vi "Beampointing_Multi_Pico3.vi"() -> ()   [LabVIEW 2013]
uses:
  shared programs/GUI_Template/GUI_master/tcp new data cluster.ctl
  <vilib>/Analysis/NI_AALBase.lvlib
  <userlib>/_OpenG.lib/array/array.llb/Filter 1D Array with Scalar (String)__ogtk.vi
  Ctrs/beam detection.ctl
  GUI_Beampointing_single_TRA/Ctrs/move.ctl
  <vilib>/Utility/file.llb/Write To Spreadsheet File (string).vi
  <userlib>/_OpenG.lib/array/array.llb/Filter 1D Array (String)__ogtk.vi
  <vilib>/Utility/file.llb/Read From Spreadsheet File (string).vi
  <vilib>/Utility/error.llb/DialogType.ctl
  shared programs/GUI_Template/GUI_master/tcp_new_data_event.ctl
panel:
  out "x-y*floor(x/y)":dbl
  out "error out":errorcluster
  out "config path":string
  out "Array 3":bool[](array[boolean])
  out "Array 2":u16[](array[numeric])
  out "Array":u16[](array[numeric])
  out "Moving Y":string
  out "Moving X":string
  out "particles":T1(array[cluster])
  out "millisecond timer value":u32
  out "appended path":path
  out "millisecond timer 2":u32
  in  "GUIdevice 98":string="PicoPad4"
  in  "Position.Axis 111::98":dbl=77.0 caption="Motor Axis 1" min=-30000.0 max=30000.0 format="%#_6f"
  in  "Position.Axis 112::98":dbl=77.0 caption="Motor Axis 1" min=-20000.0 max=20000.0 format="%#_6f"
  in  "Position.Axis 113::98":dbl=77.0 caption="Motor Axis 1" min=-20000.0 max=20000.0 format="%#_6f"
  in  "Position.Axis 121::98":dbl=77.0 caption="Motor Axis 1" min=-999999.0 max=999999.0 format="%#_6f"
  in  "Position.Axis 122::98":dbl=77.0 caption="Motor Axis 1" min=-999999.0 max=999999.0 format="%#_6f"
  in  "Position.Axis 123::98":dbl=77.0 caption="Motor Axis 1" min=-999999.0 max=999999.0 format="%#_6f"
  in  "Position.Axis 131::98":dbl=77.0 caption="Motor Axis 1" min=-999999.0 max=999999.0 format="%#_6f"
  in  "Position.Axis 132::98":dbl=77.0 caption="Motor Axis 1" min=-999999.0 max=999999.0 format="%#_6f"
  in  "Position.Axis 133::98":dbl=77.0 caption="Motor Axis 1" min=-999999.0 max=999999.0 format="%#_6f"
  in  "Position.Axis 141::98":dbl=77.0 caption="Motor Axis 1" min=-999999.0 max=999999.0 format="%#_6f"
  in  "Position.Axis 142::98":dbl=77.0 caption="Motor Axis 1" min=-999999.0 max=999999.0 format="%#_6f"
  in  "Position.Axis 143::98":dbl=77.0 caption="Motor Axis 1" min=-999999.0 max=999999.0 format="%#_6f"
  in  "Position.Axis 211::98":dbl=77.0 caption="Motor Axis 1" min=-999999.0 max=999999.0 format="%#_6f"
  in  "Position.Axis 212::98":dbl=77.0 caption="Motor Axis 1" min=-999999.0 max=999999.0 format="%#_6f"
  in  "Position.Axis 213::98":dbl=77.0 caption="Motor Axis 1" min=-999999.0 max=999999.0 format="%#_6f"
  in  "Position.Axis 221::98":dbl=77.0 caption="Motor Axis 1" min=-999999.0 max=999999.0 format="%#_6f"
  in  "Position.Axis 222::98":dbl=77.0 caption="Motor Axis 1" min=-999999.0 max=999999.0 format="%#_6f"
  in  "Position.Axis 223::98":dbl=77.0 caption="Motor Axis 1" min=-999999.0 max=999999.0 format="%#_6f"
  in  "Position.Axis 231::98":dbl=77.0 caption="Motor Axis 1" min=-999999.0 max=999999.0 format="%#_6f"
  in  "Position.Axis 232::98":dbl=77.0 caption="Motor Axis 1" min=-999999.0 max=999999.0 format="%#_6f"
  in  "Position.Axis 233::98":dbl=77.0 caption="Motor Axis 1" min=-999999.0 max=999999.0 format="%#_6f"
  in  "Position.Axis 241::98":dbl=77.0 caption="Motor Axis 1" min=-999999.0 max=999999.0 format="%#_6f"
  in  "Position.Axis 242::98":dbl=77.0 caption="Motor Axis 1" min=-999999.0 max=999999.0 format="%#_6f"
  in  "Position.Axis 243::98":dbl=77.0 caption="Motor Axis 1" min=-999999.0 max=999999.0 format="%#_6f"
  in  "Position.Axis 311::98":dbl=77.0 caption="Motor Axis 1" min=-999999.0 max=999999.0 format="%#_6f"
  in  "Position.Axis 312::98":dbl=77.0 caption="Motor Axis 1" min=-999999.0 max=999999.0 format="%#_6f"
  in  "Position.Axis 313::98":dbl=77.0 caption="Motor Axis 1" min=-999999.0 max=999999.0 format="%#_6f"
  in  "Position.Axis 321::98":dbl=77.0 caption="Motor Axis 1" min=-999999.0 max=999999.0 format="%#_6f"
  in  "Position.Axis 322::98":dbl=77.0 caption="Motor Axis 1" min=-999999.0 max=999999.0 format="%#_6f"
  in  "Position.Axis 323::98":dbl=77.0 caption="Motor Axis 1" min=-999999.0 max=999999.0 format="%#_6f"
  in  "Position.Axis 331::98":dbl=77.0 caption="Motor Axis 1" min=-999999.0 max=999999.0 format="%#_6f"
  in  "Position.Axis 332::98":dbl=77.0 caption="Motor Axis 1" min=-999999.0 max=999999.0 format="%#_6f"
  in  "Position.Axis 333::98":dbl=77.0 caption="Motor Axis 1" min=-999999.0 max=999999.0 format="%#_6f"
  in  "Position.Axis 341::98":dbl=77.0 caption="Motor Axis 1" min=-999999.0 max=999999.0 format="%#_6f"
  in  "Position.Axis 342::98":dbl=77.0 caption="Motor Axis 1" min=-999999.0 max=999999.0 format="%#_6f"
  in  "Position.Axis 343::98":dbl=77.0 caption="Motor Axis 1" min=-999999.0 max=999999.0 format="%#_6f"
  in  "Position.Axis 411::98":dbl=77.0 caption="Motor Axis 1" min=-999999.0 max=999999.0 format="%#_6f"
  in  "Position.Axis 412::98":dbl=77.0 caption="Motor Axis 1" min=-999999.0 max=999999.0 format="%#_6f"
  in  "Position.Axis 413::98":dbl=77.0 caption="Motor Axis 1" min=-999999.0 max=999999.0 format="%#_6f"
  in  "Position.Axis 421::98":dbl=77.0 caption="Motor Axis 1" min=-999999.0 max=999999.0 format="%#_6f"
  in  "Position.Axis 422::98":dbl=77.0 caption="Motor Axis 1" min=-999999.0 max=999999.0 format="%#_6f"
  in  "Position.Axis 423::98":dbl=77.0 caption="Motor Axis 1" min=-999999.0 max=999999.0 format="%#_6f"
  in  "Position.Axis 431::98":dbl=77.0 caption="Motor Axis 1" min=-999999.0 max=999999.0 format="%#_6f"
  in  "Position.Axis 432::98":dbl=77.0 caption="Motor Axis 1" min=-999999.0 max=999999.0 format="%#_6f"
  in  "Position.Axis 433::98":dbl=77.0 caption="Motor Axis 1" min=-999999.0 max=999999.0 format="%#_6f"
  in  "Position.Axis 441::98":dbl=77.0 caption="Motor Axis 1" min=-999999.0 max=999999.0 format="%#_6f"
  in  "Position.Axis 442::98":dbl=77.0 caption="Motor Axis 1" min=-999999.0 max=999999.0 format="%#_6f"
  in  "Position.Axis 443::98":dbl=77.0 caption="Motor Axis 1" min=-999999.0 max=999999.0 format="%#_6f"
  in  "Position.Axis 511::98":dbl=77.0 caption="Motor Axis 1" min=-999999.0 max=999999.0 format="%#_6f"
  in  "Position.Axis 512::98":dbl=77.0 caption="Motor Axis 1" min=-999999.0 max=999999.0 format="%#_6f"
  in  "Position.Axis 513::98":dbl=77.0 caption="Motor Axis 1" min=-999999.0 max=999999.0 format="%#_6f"
  in  "Position.Axis 521::98":dbl=77.0 caption="Motor Axis 1" min=-999999.0 max=999999.0 format="%#_6f"
  in  "Position.Axis 522::98":dbl=77.0 caption="Motor Axis 1" min=-999999.0 max=999999.0 format="%#_6f"
  in  "Position.Axis 523::98":dbl=77.0 caption="Motor Axis 1" min=-999999.0 max=999999.0 format="%#_6f"
  in  "Position.Axis 531::98":dbl=77.0 caption="Motor Axis 1" min=-999999.0 max=999999.0 format="%#_6f"
  in  "Position.Axis 532::98":dbl=77.0 caption="Motor Axis 1" min=-999999.0 max=999999.0 format="%#_6f"
  in  "Position.Axis 533::98":dbl=77.0 caption="Motor Axis 1" min=-999999.0 max=999999.0 format="%#_6f"
  in  "Position.Axis 541::98":dbl=77.0 caption="Motor Axis 1" min=-999999.0 max=999999.0 format="%#_6f"
  in  "Position.Axis 542::98":dbl=77.0 caption="Motor Axis 1" min=-999999.0 max=999999.0 format="%#_6f"
  in  "Position.Axis 543::98":dbl=77.0 caption="Motor Axis 1" min=-999999.0 max=999999.0 format="%#_6f"
  in  "Numeric":dbl
  out "Current State":string
  in  "output cluster 2":T5 {"detection para"."smal para"."Measurement Parameter" items=["Center of Mass X", "Center of Mass Y", "First Pixel X", "First Pixel Y", "Bounding Rect Left", "Bounding Rect Top", "Bounding Rect Right", "Bounding Rect Bottom", "Max Feret Diameter Start X", "Max Feret Diameter Start Y", "Max Feret Diameter End X", "Max Feret Diameter End Y", "Max Horiz. Segment Length Left", "Max Horiz. Segment Length Right", "Max Horiz. Segment Length Row", "-", "Bounding Rect Width", "Bounding Rect Height", "Bounding Rect Diagonal", "Perimeter", "Convex Hull Perimeter", "Holes' Perimeter", "Max Feret Diameter", "Equivalent Ellipse Major Axis", "Equivalent Ellipse Minor Axis", "Equivalent Ellipse Minor Axis (Feret)", "Equivalent Rect Long Side", "Equivalent Rect Short Side", "Equivalent Rect Diagonal", "Equivalent Rect Short Side (Feret)", "Average Horiz. Segment Length", "Average Vert. Segment Length", "Hydraulic Radius", "Waddel Disk Diameter", "-", "Area", "Holes' Area", "Particle & Holes' Area", "Convex Hull Area", "Image Area", "-", "Number of Holes", "Number of Horiz. Segments", "Number of Vert. Segments", "-", "Orientation", "Max Feret Diameter Orientation", "-", "% Area/Image Area", "% Area/(Particle & Holes' Area)", "Ratio of Equivalent Ellipse Axes", "Ratio of Equivalent Rect Sides", "-", "Elongation Factor", "Compactness Factor", "Heywood Circularity Factor", "Type Factor", "-", "Sum X", "Sum Y", "Sum XX", "Sum XY", "Sum YY", "Sum XXX", "Sum XXY", "Sum XYY", "Sum YYY", "-", "Moment of Inertia XX", "Moment of Inertia XY", "Moment of Inertia YY", "Moment of Inertia XXX", "Moment of Inertia XXY", "Moment of Inertia XYY", "Moment of Inertia YYY", "Norm. Moment of Inertia XX", "Norm. Moment of Inertia XY", "Norm. Moment of Inertia YY", "Norm. Moment of Inertia XXX", "Norm. Moment of Inertia XXY", "Norm. Moment of Inertia XYY", "Norm. Moment of Inertia YYY", "Hu Moment 1", "Hu Moment 2", "Hu Moment 3", "Hu Moment 4", "Hu Moment 5", "Hu Moment 6", "Hu Moment 7"]; "detection para"."smal para"."Range Lower Value" format="%.2f"; "detection para"."smal para"."Range Upper Value" format="%.2f"; "detection para"."detection method" items=["clustering", "entropy", "metric", "moments", "inter-class variance"]; "detection para"."Filter" items=["No Filter", "Median Filter", "Low Pass Filter"]}
  out "CCDs":string[](array[string])
  in  "GUIdevice 12":string
  in  "GUIdevice 11":string
  in  "GUIdevice 10":string
  in  "GUIdevice 9":string
  out "error out 2":errorcluster
  in  "active cams":string[](array[string])
  in  "Motor Y":dbl[][](array[numeric])
  in  "Motor X":dbl[][](array[numeric])
  out "Names":string[](array[string])
  in  "Offset X stats":dbl[][](array[numeric])
  in  "Offset Y stats":dbl[][](array[numeric])
  out "Box":T6(array[cluster])
  in  "Tab Control 2":enum32{"Config ", "Main", "History"}(tab)=enum."Main"
  out "Waveform Chart":u32(graph)
  in  "associated motors":T7
  out "Cameras":T8
  out "Status":cluster{i32, i32, "Centroid X":dbl[][]}(graph)
  in  "Exposure:12":dbl=0.095 min=0.0001 max=1.0 format="%#_6f"
  in  "Triggerdelay::12":dbl=0.003 min=0.0 max=0.09 format="%#_6f"
  in  "Exposure::11":dbl=0.095 min=0.0001 max=1.0 format="%#_6f"
  in  "Triggerdelay::11":dbl=0.003 min=0.0 max=0.09 format="%#_6f"
  in  "Exposure::10":dbl=0.095 min=0.0001 max=1.0 format="%#_6f"
  in  "Triggerdelay::10":dbl=0.003 min=0.0 max=0.09 format="%#_6f"
  in  "Exposure::9":dbl=0.095 min=0.0001 max=1.0 format="%#_6f"
  in  "Triggerdelay::9":dbl=0.003 min=0.0 max=0.09 format="%#_6f"
  in  "Trigger::9":bool
  in  "Trigger::10":bool caption="Trigger:10"
  in  "Trigger::11":bool
  in  "Trigger::12":bool
  in  "Target.Y::9":dbl=45.0 caption="T9y" min=0.0 max=2000.0 format="%#_6f"
  in  "Target.X::9":dbl=47.0 caption="Tx9" min=0.0 max=2000.0 format="%#_6f"
  in  "Target.Y::10":dbl=45.0 caption="T10y" min=0.0 max=2000.0 format="%#_6f"
  in  "Target.X::10":dbl=47.0 caption="T10x" min=0.0 max=2000.0 format="%#_6f"
  in  "Target.Y::11":dbl=45.0 caption="T11y" min=0.0 max=2000.0 format="%#_6f"
  in  "Target.X::11":dbl=47.0 caption="T11x" min=0.0 max=2000.0 format="%#_6f"
  in  "Target.Y::12":dbl=45.0 caption="T12y" min=0.0 max=2000.0 format="%#_6f"
  in  "Target.X::12":dbl=47.0 caption="T12x" min=0.0 max=2000.0 format="%#_6f"
  in  "Exposure::8":dbl=0.095 min=0.01 max=1.0 format="%#_6f"
  in  "Triggerdelay::8":dbl=0.003 min=0.0 max=0.09 format="%#_6f"
  in  "Trigger::8":bool
  in  "Target.Y::8":dbl=45.0 caption="T8y" min=0.0 max=2000.0 format="%#_6f"
  in  "Target.X::8":dbl=47.0 caption="T8x" min=0.0 max=2000.0 format="%#_6f"
  in  "Target.Y::7":dbl=45.0 caption="T7x" min=0.0 max=2000.0 format="%#_6f"
  in  "Target.X::7":dbl=47.0 caption="T7y" min=0.0 max=2000.0 format="%#_6f"
  in  "Target.Y::6":dbl=45.0 caption="T6y" min=0.0 max=2000.0 format="%#_6f"
  in  "Target.X::6":dbl=47.0 caption="T6x" min=0.0 max=2000.0 format="%#_6f"
  in  "Target.Y::5":dbl=45.0 caption="T5y" min=0.0 max=2000.0 format="%#_6f"
  in  "Target.X::5":dbl=47.0 caption="T5x" min=0.0 max=2000.0 format="%#_6f"
  in  "Target.Y::4":dbl=45.0 caption="T4y" min=0.0 max=2000.0 format="%#_6f"
  in  "Target.X::4":dbl=47.0 caption="T4x" min=0.0 max=2000.0 format="%#_6f"
  in  "Target.Y::3":dbl=163.0 caption="T3y" min=0.0 max=2000.0 format="%#_6f"
  in  "Target.X::3":dbl=152.0 caption="T3x" min=0.0 max=2000.0 format="%#_6f"
  in  "Target.Y::2":dbl=74.0 caption="T2y" min=1.0 max=600.0 format="%#_6f"
  in  "Target.X::2":dbl=75.0 caption="T2x" min=1.0 max=800.0 format="%#_6f"
  in  "Target.Y::1":dbl=61.0 caption="T1y" min=1.0 max=600.0 format="%#_6f"
  in  "Target.X::1":dbl=77.0 caption="T1x" min=1.0 max=800.0 format="%#_6f"
  in  "Exposure::7":dbl=0.095 min=0.0001 max=1.0 format="%#_6f"
  in  "Triggerdelay::7":dbl=0.003 min=0.0 max=0.09 format="%#_6f"
  in  "Trigger::7":bool
  in  "Exposure::6":dbl=0.095 min=0.0001 max=1.0 format="%#_6f"
  in  "Triggerdelay::6":dbl=0.003 min=0.0 max=0.09 format="%#_6f"
  in  "Trigger::6":bool
  in  "Exposure::5":dbl=0.095 min=0.0001 max=1.0 format="%#_6f"
  in  "Triggerdelay::5":dbl=0.003 min=0.0 max=0.09 format="%#_6f"
  in  "Trigger::5":bool
  in  "Exposure::4":dbl=0.095 min=0.0001 max=1.0 format="%#_6f"
  in  "Triggerdelay::4":dbl=0.003 min=0.0 max=0.09 format="%#_6f"
  in  "Trigger::4":bool
  in  "Exposure::3":dbl=0.095 min=0.0001 max=1.0 format="%#_6f"
  in  "Triggerdelay::3":dbl=0.003 min=0.0 max=0.09 format="%#_6f"
  in  "Trigger::3":bool
  in  "Exposure::2":dbl=0.095 min=0.0001 max=1.0 format="%#_6f"
  in  "Triggerdelay::2":dbl=0.003 min=0.0 max=0.09 format="%#_6f"
  in  "Trigger::2":bool
  out "image::1":T9(plugin-control) caption="PA2_Input1"
  out "image::2":T9(plugin-control) caption="PA2_Input2"
  out "image::3":T9(plugin-control) caption="L1_TelInpNear"
  out "image::4":T9(plugin-control) caption="L2_TelInpFar"
  out "image::5":T9(plugin-control) caption="L4_TREXpass1"
  out "image::6":T9(plugin-control) caption="L5_TREXPass2"
  out "image::7":T9(plugin-control) caption="L6_TREXpass3"
  out "image::8":T9(plugin-control) caption="L7_TREXPass4"
  in  "Exposure::1":dbl=0.095 min=0.0001 max=1.0 format="%#_6f"
  in  "Triggerdelay::1":dbl=0.003 min=0.0 max=0.09 format="%#_6f"
  in  "Trigger::1":bool
  in  "UDP error message":string
  out "required Y":bool[](array[boolean])
  out "required X":bool[](array[boolean])
  out "detected":bool[](array[boolean])
  out "name array":string[](array[string])
  out "image::9":T9(plugin-control) caption="L8_M10Leak"
  out "image::10":T9(plugin-control) caption="B1_TelInput"
  out "image::11":T9(plugin-control) caption="B2_TelLens1"
  out "image::12":T9(plugin-control) caption="B3_TelLens2"
  out "speedmode X":bool[](array[boolean])
  out "speedmode Y":bool[](array[boolean])
  out "CCD 9":cluster{timestamp[], dbl[]}[](graph)
  out "CCD 10":cluster{timestamp[], dbl[]}[](graph)
  out "CCD 11":cluster{timestamp[], dbl[]}[](graph)
  out "CCD 12":cluster{timestamp[], dbl[]}[](graph)
  out "CCD 5":cluster{timestamp[], dbl[]}[](graph)
  out "CCD 6":cluster{timestamp[], dbl[]}[](graph)
  out "CCD 7":cluster{timestamp[], dbl[]}[](graph)
  out "CCD 8":cluster{timestamp[], dbl[]}[](graph)
  out "CCD 2":cluster{timestamp[], dbl[]}[](graph)
  out "CCD 1":cluster{timestamp[], dbl[]}[](graph)
  out "CCD 3":cluster{timestamp[], dbl[]}[](graph)
  out "CCD 4":cluster{timestamp[], dbl[]}[](graph)
  out "History index":i32
  in  "History Size":i32=500
  out "Particle Reports (Pixels)":T10(array[cluster])
  in  "Feedback Global":bool
  in  "detection para":T3[](array[typedef])=[{"Filter"=1, "Filter Para"={"X Size"=5, "Y Size"=5, "% Tolerance"=1}, "detection method"=4, "smal para"=[{"Measurement Parameter"=35, "Range Lower Value"=0.0, "Range Upper Value"=0.0, "Range"=TRUE, "Measurement Type"=FALSE}], "Remove small Objects"=TRUE, "Restrict to round Objects"=FALSE}, {"Filter"=1, "Filter Para"={"X Size"=5, "Y Size"=5, "% Tolerance"=1}, "detection method"=4, "smal para"=[{"Measurement Parameter"=35, "Range Lower Value"=0.0, "Range Upper Value"=500.0, "Range"=FALSE, "Measurement Type"=FALSE}], "Remove small Objects"=TRUE, "Restrict to round Objects"=FALSE}, {"Filter"=1, "Filter Para"={"X Size"=5, "Y Size"=5, "% Tolerance"=1}, "detection method"=4, "smal para"=[{"Measurement Parameter"=35, "Range Lower Value"=0.0, "Range Upper Value"=500.0, "Range"=TRUE, "Measurement Type"=FALSE}], "Remove small Objects"=TRUE, "Restrict to round Objects"=FALSE}, {"Filter"=1, "Filter Para"={"X Size"=5, "Y Size"=5, "% Tolerance"=1}, "detection method"=4, "smal para"=[{"Measurement Parameter"=35, "Range Lower Value"=0.0, "Range Upper Value"=500.0, "Range"=TRUE, "Measurement Type"=FALSE}], "Remove small Objects"=TRUE, "Restrict to round Objects"=FALSE}, {"Filter"=1, "Filter Para"={"X Size"=5, "Y Size"=5, "% Tolerance"=1}, "detection method"=4, "smal para"=[{"Measurement Parameter"=35, "Range Lower Value"=0.0, "Range Upper Value"=500.0, "Range"=TRUE, "Measurement Type"=FALSE}], "Remove small Objects"=TRUE, "Restrict to round Objects"=FALSE}, {"Filter"=1, "Filter Para"={"X Size"=5, "Y Size"=5, "% Tolerance"=1}, "detection method"=4, "smal para"=[{"Measurement Parameter"=35, "Range Lower Value"=0.0, "Range Upper Value"=500.0, "Range"=TRUE, "Measurement Type"=FALSE}], "Remove small Objects"=TRUE, "Restrict to round Objects"=FALSE}, {"Filter"=1, "Filter Para"={"X Size"=5, "Y Size"=5, "% Tolerance"=1}, "detection method"=4, "smal para"=[{"Measurement Parameter"=35, "Range Lower Value"=0.0, "Range Upper Value"=500.0, "Range"=TRUE, "Measurement Type"=FALSE}], "Remove small Objects"=TRUE, "Restrict to round Objects"=FALSE}, {"Filter"=1, "Filter Para"={"X Size"=5, "Y Size"=5, "% Tolerance"=1}, "detection method"=3, "smal para"=[{"Measurement Parameter"=35, "Range Lower Value"=0.0, "Range Upper Value"=0.0, "Range"=FALSE, "Measurement Type"=FALSE}], "Remove small Objects"=TRUE, "Restrict to round Objects"=FALSE}, {"Filter"=1, "Filter Para"={"X Size"=5, "Y Size"=5, "% Tolerance"=1}, "detection method"=4, "smal para"=[{"Measurement Parameter"=35, "Range Lower Value"=0.0, "Range Upper Value"=0.0, "Range"=FALSE, "Measurement Type"=FALSE}], "Remove small Objects"=TRUE, "Restrict to round Objects"=FALSE}, {"Filter"=1, "Filter Para"={"X Size"=5, "Y Size"=5, "% Tolerance"=1}, "detection method"=4, "smal para"=[{"Measurement Parameter"=35, "Range Lower Value"=0.0, "Range Upper Value"=500.0, "Range"=TRUE, "Measurement Type"=FALSE}], "Remove small Objects"=TRUE, "Restrict to round Objects"=FALSE}, {"Filter"=1, "Filter Para"={"X Size"=5, "Y Size"=5, "% Tolerance"=1}, "detection method"=4, "smal para"=[{"Measurement Parameter"=35, "Range Lower Value"=0.0, "Range Upper Value"=500.0, "Range"=TRUE, "Measurement Type"=FALSE}], "Remove small Objects"=TRUE, "Restrict to round Objects"=FALSE}, {"Filter"=1, "Filter Para"={"X Size"=5, "Y Size"=5, "% Tolerance"=1}, "detection method"=4, "smal para"=[{"Measurement Parameter"=35, "Range Lower Value"=0.0, "Range Upper Value"=500.0, "Range"=TRUE, "Measurement Type"=FALSE}], "Remove small Objects"=TRUE, "Restrict to round Objects"=FALSE}] {"smal para"."Measurement Parameter" items=["Center of Mass X", "Center of Mass Y", "First Pixel X", "First Pixel Y", "Bounding Rect Left", "Bounding Rect Top", "Bounding Rect Right", "Bounding Rect Bottom", "Max Feret Diameter Start X", "Max Feret Diameter Start Y", "Max Feret Diameter End X", "Max Feret Diameter End Y", "Max Horiz. Segment Length Left", "Max Horiz. Segment Length Right", "Max Horiz. Segment Length Row", "-", "Bounding Rect Width", "Bounding Rect Height", "Bounding Rect Diagonal", "Perimeter", "Convex Hull Perimeter", "Holes' Perimeter", "Max Feret Diameter", "Equivalent Ellipse Major Axis", "Equivalent Ellipse Minor Axis", "Equivalent Ellipse Minor Axis (Feret)", "Equivalent Rect Long Side", "Equivalent Rect Short Side", "Equivalent Rect Diagonal", "Equivalent Rect Short Side (Feret)", "Average Horiz. Segment Length", "Average Vert. Segment Length", "Hydraulic Radius", "Waddel Disk Diameter", "-", "Area", "Holes' Area", "Particle & Holes' Area", "Convex Hull Area", "Image Area", "-", "Number of Holes", "Number of Horiz. Segments", "Number of Vert. Segments", "-", "Orientation", "Max Feret Diameter Orientation", "-", "% Area/Image Area", "% Area/(Particle & Holes' Area)", "Ratio of Equivalent Ellipse Axes", "Ratio of Equivalent Rect Sides", "-", "Elongation Factor", "Compactness Factor", "Heywood Circularity Factor", "Type Factor", "-", "Sum X", "Sum Y", "Sum XX", "Sum XY", "Sum YY", "Sum XXX", "Sum XXY", "Sum XYY", "Sum YYY", "-", "Moment of Inertia XX", "Moment of Inertia XY", "Moment of Inertia YY", "Moment of Inertia XXX", "Moment of Inertia XXY", "Moment of Inertia XYY", "Moment of Inertia YYY", "Norm. Moment of Inertia XX", "Norm. Moment of Inertia XY", "Norm. Moment of Inertia YY", "Norm. Moment of Inertia XXX", "Norm. Moment of Inertia XXY", "Norm. Moment of Inertia XYY", "Norm. Moment of Inertia YYY", "Hu Moment 1", "Hu Moment 2", "Hu Moment 3", "Hu Moment 4", "Hu Moment 5", "Hu Moment 6", "Hu Moment 7"]; "smal para"."Range Lower Value" format="%.2f"; "smal para"."Range Upper Value" format="%.2f"; "detection method" items=["clustering", "entropy", "metric", "moments", "inter-class variance"]; "Filter" items=["No Filter", "Median Filter", "Low Pass Filter"]}
  in  "GUIdevice 8":string="B5_CompressorOut"
  in  "Tab Control":T11(tab)
  in  "Center":bool
  in  "Save Stats":bool
  in  "Save Config":bool
  in  "Load Config":bool
  in  "update speed [ms]":i32=200
  in  "Img to avg":i32=20 min=3 max=200
  in  "Reset History":bool
  in  "save path":path=path "W:/BP_DATA"
  in  "autodetect":bool
  in  "Detection Rate":dbl=0.8 min=0.001 max=1.0
  in  "new tdms":bool
  in  "Speedmode @":dbl=3.0 min=1.0 max=20.0
  in  "Align":bool
  in  "deivice ini":bool
  in  "beam detection para":T3={"Filter"=1, "Filter Para"={"X Size"=5, "Y Size"=5, "% Tolerance"=1}, "detection method"=4, "smal para"=[{"Measurement Parameter"=35, "Range Lower Value"=0.0, "Range Upper Value"=500.0, "Range"=FALSE, "Measurement Type"=FALSE}], "Remove small Objects"=TRUE, "Restrict to round Objects"=FALSE} {"smal para"."Measurement Parameter" items=["Center of Mass X", "Center of Mass Y", "First Pixel X", "First Pixel Y", "Bounding Rect Left", "Bounding Rect Top", "Bounding Rect Right", "Bounding Rect Bottom", "Max Feret Diameter Start X", "Max Feret Diameter Start Y", "Max Feret Diameter End X", "Max Feret Diameter End Y", "Max Horiz. Segment Length Left", "Max Horiz. Segment Length Right", "Max Horiz. Segment Length Row", "-", "Bounding Rect Width", "Bounding Rect Height", "Bounding Rect Diagonal", "Perimeter", "Convex Hull Perimeter", "Holes' Perimeter", "Max Feret Diameter", "Equivalent Ellipse Major Axis", "Equivalent Ellipse Minor Axis", "Equivalent Ellipse Minor Axis (Feret)", "Equivalent Rect Long Side", "Equivalent Rect Short Side", "Equivalent Rect Diagonal", "Equivalent Rect Short Side (Feret)", "Average Horiz. Segment Length", "Average Vert. Segment Length", "Hydraulic Radius", "Waddel Disk Diameter", "-", "Area", "Holes' Area", "Particle & Holes' Area", "Convex Hull Area", "Image Area", "-", "Number of Holes", "Number of Horiz. Segments", "Number of Vert. Segments", "-", "Orientation", "Max Feret Diameter Orientation", "-", "% Area/Image Area", "% Area/(Particle & Holes' Area)", "Ratio of Equivalent Ellipse Axes", "Ratio of Equivalent Rect Sides", "-", "Elongation Factor", "Compactness Factor", "Heywood Circularity Factor", "Type Factor", "-", "Sum X", "Sum Y", "Sum XX", "Sum XY", "Sum YY", "Sum XXX", "Sum XXY", "Sum XYY", "Sum YYY", "-", "Moment of Inertia XX", "Moment of Inertia XY", "Moment of Inertia YY", "Moment of Inertia XXX", "Moment of Inertia XXY", "Moment of Inertia XYY", "Moment of Inertia YYY", "Norm. Moment of Inertia XX", "Norm. Moment of Inertia XY", "Norm. Moment of Inertia YY", "Norm. Moment of Inertia XXX", "Norm. Moment of Inertia XXY", "Norm. Moment of Inertia XYY", "Norm. Moment of Inertia YYY", "Hu Moment 1", "Hu Moment 2", "Hu Moment 3", "Hu Moment 4", "Hu Moment 5", "Hu Moment 6", "Hu Moment 7"]; "smal para"."Range Lower Value" format="%.2f"; "smal para"."Range Upper Value" format="%.2f"; "detection method" items=["clustering", "entropy", "metric", "moments", "inter-class variance"]; "Filter" items=["No Filter", "Median Filter", "Low Pass Filter"]}
  in  "move config":T2={"Tolerance [%]"=0.1, "Stepsize"=0.0001, "Invert Axis"=TRUE, "Invert Direction X"=FALSE, "Invert Direction Y"=TRUE, "enable feedback"=FALSE, "Set Centriod Target"=FALSE}
  in  "ActiveMotor":u16(ring)=7 items=["PA2_Input1", "PA2_Input2", "L2_TelInpFar", "L1_TelInpNear", "L4_TREXPASS1", "L5_TREXPass2", "L6_TREXPass3", "L7_TREXPass4", "L8_M10Leak", "B1_TelInput", "B2_TelLens1", "NoName", "NoName", "NoName", "MBeamSplitterL", "Mdiode", "NoName", "NoName", "NoName", "NoName"]
  in  "ActiveMotorName::99":string
  in  "RelativeMove.Axis 1.CCW::99":bool caption="RelativeMove.Axis 1.CCW::1"
  in  "RelativeMove.Axis 1.CW::99":bool caption="RelativeMove.Axis 1.CW::1"
  in  "RelativeMove.Axis 2.CCW::99":bool caption="RelativeMove.Axis. 2.CCW::1"
  in  "RelativeMove.Axis 2.CW::99":bool caption="RelativeMove.Axis 2.CW::1"
  in  "RelativeSettings.Axis 1.Position::99":dbl caption="Axis 1 Position" min=-999999.0 max=999999.0 format="%_4p"
  in  "RelativeSettings.Axis 2.Position::99":dbl caption="Axis 2 Position" min=-999999.0 max=999999.0 format="%_4p"
  in  "RelativeSettings.Axis 2.StepSize::99":dbl=50.0 caption="Axis 2 StepSize" min=0.0 max=999999.0 format="%_4p"
  in  "RelativeSettings.Axis 1.StepSize::99":dbl=50.0 caption="Axis 1 Stepsize" min=0.0 max=999999.0 format="%_4p"
  in  "ActiveMotor 2":u16(ring)=7
  in  "ActiveMotorName::98":string
  in  "RelativeMove.Axis 1.CCW::98":bool caption="RelativeMove.Axis 1.CCW::1"
  in  "RelativeMove.Axis 1.CW::98":bool caption="RelativeMove.Axis 1.CW::1"
  in  "RelativeMove.Axis 2.CCW::98":bool caption="RelativeMove.Axis. 2.CCW::1"
  in  "RelativeMove.Axis 2.CW::98":bool caption="RelativeMove.Axis 2.CW::1"
  in  "RelativeSettings.Axis 1.Position::98":dbl caption="Axis 1 Position" min=-999999.0 max=999999.0 format="%_4p"
  in  "RelativeSettings.Axis 2.Position::98":dbl caption="Axis 2 Position" min=-999999.0 max=999999.0 format="%_4p"
  in  "RelativeSettings.Axis 2.StepSize::98":dbl=50.0 caption="Axis 2 StepSize" min=0.0 max=999999.0 format="%_4p"
  in  "RelativeSettings.Axis 1.StepSize::98":dbl=50.0 caption="Axis 1 Stepsize" min=0.0 max=999999.0 format="%_4p"
  out "Arguments Y":string
  in  "active axis refs 2":T12(array[cluster])
  in  "active Axis ref":cluster{"Ref X":refnum<vi>, "Ref Y":refnum<vi>}
  in  "CCDs":u16(ring) items=["PA2_Input1", "PA2_Input2", "L1_TelInpNear", "L2_TelInpFar", "L4_TREXpass1", "L5_TREXPass2", "L6_TREXpass3", "L7_TREXPass4", "L8_M10Leak", "B1_TelInput", "B2_TelLens1", "B3_TelLens2"]
  out "motor refs":refnum<vi>[](array[refnum])
  in  "Position.Axis 511::99":dbl=77.0 caption="Motor Axis 1" min=-20000.0 max=20000.0 format="%#_6f"
  in  "Position.Axis 512::99":dbl=77.0 caption="Motor Axis 1" min=-20000.0 max=20000.0 format="%#_6f"
  in  "Position.Axis 513::99":dbl=77.0 caption="Motor Axis 1" min=-20000.0 max=20000.0 format="%#_6f"
  in  "Position.Axis 521::99":dbl=77.0 caption="Motor Axis 1" min=-20000.0 max=20000.0 format="%#_6f"
  in  "Position.Axis 522::99":dbl=77.0 caption="Motor Axis 1" min=-20000.0 max=20000.0 format="%#_6f"
  in  "Position.Axis 523::99":dbl=77.0 caption="Motor Axis 1" min=-20000.0 max=20000.0 format="%#_6f"
  in  "Position.Axis 531::99":dbl=77.0 caption="Motor Axis 1" min=-20000.0 max=20000.0 format="%#_6f"
  in  "Position.Axis 532::99":dbl=77.0 caption="Motor Axis 1" min=-20000.0 max=20000.0 format="%#_6f"
  in  "Position.Axis 533::99":dbl=77.0 caption="Motor Axis 1" min=-20000.0 max=20000.0 format="%#_6f"
  in  "Position.Axis 541::99":dbl=77.0 caption="Motor Axis 1" min=-20000.0 max=20000.0 format="%#_6f"
  in  "Position.Axis 542::99":dbl=77.0 caption="Motor Axis 1" min=-20000.0 max=20000.0 format="%#_6f"
  in  "Position.Axis 543::99":dbl=77.0 caption="Motor Axis 1" min=-20000.0 max=20000.0 format="%#_6f"
  in  "Position.Axis 411::99":dbl=77.0 caption="Motor Axis 1" min=-20000.0 max=20000.0 format="%#_6f"
  in  "Position.Axis 412::99":dbl=77.0 caption="Motor Axis 1" min=-20000.0 max=20000.0 format="%#_6f"
  in  "Position.Axis 413::99":dbl=77.0 caption="Motor Axis 1" min=-20000.0 max=20000.0 format="%#_6f"
  in  "Position.Axis 421::99":dbl=77.0 caption="Motor Axis 1" min=-20000.0 max=20000.0 format="%#_6f"
  in  "Position.Axis 422::99":dbl=77.0 caption="Motor Axis 1" min=-20000.0 max=20000.0 format="%#_6f"
  in  "Position.Axis 423::99":dbl=77.0 caption="Motor Axis 1" min=-20000.0 max=20000.0 format="%#_6f"
  in  "Position.Axis 431::99":dbl=77.0 caption="Motor Axis 1" min=-20000.0 max=20000.0 format="%#_6f"
  in  "Position.Axis 432::99":dbl=77.0 caption="Motor Axis 1" min=-20000.0 max=20000.0 format="%#_6f"
  in  "Position.Axis 433::99":dbl=77.0 caption="Motor Axis 1" min=-20000.0 max=20000.0 format="%#_6f"
  in  "Position.Axis 441::99":dbl=77.0 caption="Motor Axis 1" min=-20000.0 max=20000.0 format="%#_6f"
  in  "Position.Axis 442::99":dbl=77.0 caption="Motor Axis 1" min=-20000.0 max=20000.0 format="%#_6f"
  in  "Position.Axis 443::99":dbl=77.0 caption="Motor Axis 1" min=-20000.0 max=20000.0 format="%#_6f"
  in  "Position.Axis 311::99":dbl=77.0 caption="Motor Axis 1" min=-50000.0 max=50000.0 format="%#_6f"
  in  "Position.Axis 312::99":dbl=77.0 caption="Motor Axis 1" min=-50000.0 max=50000.0 format="%#_6f"
  in  "Position.Axis 313::99":dbl=77.0 caption="Motor Axis 1" min=-999999.0 max=999999.0 format="%#_6f"
  in  "Position.Axis 321::99":dbl=77.0 caption="Motor Axis 1" min=-20000.0 max=20000.0 format="%#_6f"
  in  "Position.Axis 322::99":dbl=77.0 caption="Motor Axis 1" min=-20000.0 max=20000.0 format="%#_6f"
  in  "Position.Axis 323::99":dbl=77.0 caption="Motor Axis 1" min=-20000.0 max=20000.0 format="%#_6f"
  in  "Position.Axis 331::99":dbl=77.0 caption="Motor Axis 1" min=-20000.0 max=20000.0 format="%#_6f"
  in  "Position.Axis 332::99":dbl=77.0 caption="Motor Axis 1" min=-20000.0 max=20000.0 format="%#_6f"
  in  "Position.Axis 333::99":dbl=77.0 caption="Motor Axis 1" min=-20000.0 max=20000.0 format="%#_6f"
  in  "Position.Axis 341::99":dbl=77.0 caption="Motor Axis 1" min=-20000.0 max=20000.0 format="%#_6f"
  in  "Position.Axis 342::99":dbl=77.0 caption="Motor Axis 1" min=-20000.0 max=20000.0 format="%#_6f"
  in  "Position.Axis 343::99":dbl=77.0 caption="Motor Axis 1" min=-20000.0 max=20000.0 format="%#_6f"
  in  "Position.Axis 241::99":dbl=77.0 caption="Motor Axis 1" min=-20000.0 max=20000.0 format="%#_6f"
  in  "Position.Axis 242::99":dbl=77.0 caption="Motor Axis 1" min=-20000.0 max=20000.0 format="%#_6f"
  in  "Position.Axis 243::99":dbl=77.0 caption="Motor Axis 1" min=-20000.0 max=20000.0 format="%#_6f"
  in  "Position.Axis 231::99":dbl=77.0 caption="Motor Axis 1" min=-20000.0 max=20000.0 format="%#_6f"
  in  "Position.Axis 232::99":dbl=77.0 caption="Motor Axis 1" min=-20000.0 max=20000.0 format="%#_6f"
  in  "Position.Axis 233::99":dbl=77.0 caption="Motor Axis 1" min=-20000.0 max=20000.0 format="%#_6f"
  in  "Position.Axis 221::99":dbl=77.0 caption="Motor Axis 1" min=-20000.0 max=20000.0 format="%#_6f"
  in  "Position.Axis 222::99":dbl=77.0 caption="Motor Axis 1" min=-20000.0 max=200000.0 format="%#_6f"
  in  "Position.Axis 223::99":dbl=77.0 caption="Motor Axis 1" min=-20000.0 max=20000.0 format="%#_6f"
  in  "Position.Axis 211::99":dbl=77.0 caption="Motor Axis 1" min=-20000.0 max=200000.0 format="%#_6f"
  in  "Position.Axis 212::99":dbl=77.0 caption="Motor Axis 1" min=-20000.0 max=20000.0 format="%#_6f"
  in  "Position.Axis 213::99":dbl=77.0 caption="Motor Axis 1" min=-20000.0 max=20000.0 format="%#_6f"
  in  "Position.Axis 141::99":dbl=77.0 caption="Motor Axis 1" min=-20000.0 max=20000.0 format="%#_6f"
  in  "Position.Axis 142::99":dbl=77.0 caption="Motor Axis 1" min=-20000.0 max=20000.0 format="%#_6f"
  in  "Position.Axis 143::99":dbl=77.0 caption="Motor Axis 1" min=-20000.0 max=20000.0 format="%#_6f"
  in  "Position.Axis 131::99":dbl=77.0 caption="Motor Axis 1" min=-20000.0 max=20000.0 format="%#_6f"
  in  "Position.Axis 132::99":dbl=77.0 caption="Motor Axis 1" min=-20000.0 max=20000.0 format="%#_6f"
  in  "Position.Axis 133::99":dbl=77.0 caption="Motor Axis 1" min=-20000.0 max=20000.0 format="%#_6f"
  in  "Position.Axis 121::99":dbl=77.0 caption="Motor Axis 1" min=-20000.0 max=20000.0 format="%#_6f"
  in  "Position.Axis 122::99":dbl=77.0 caption="Motor Axis 1" min=-20000.0 max=20000.0 format="%#_6f"
  in  "Position.Axis 123::99":dbl=77.0 caption="Motor Axis 1" min=-20000.0 max=20000.0 format="%#_6f"
  in  "Position.Axis 113::99":dbl=77.0 caption="Motor Axis 1" min=-20000.0 max=20000.0 format="%#_6f"
  in  "Position.Axis 112::99":dbl=77.0 caption="Motor Axis 1" min=-20000.0 max=20000.0 format="%#_6f"
  in  "Position.Axis 111::99":dbl=77.0 caption="Motor Axis 1" min=-20000.0 max=20000.0 format="%#_6f"
  out "Arguments X":string
  in  "GUIdevice 99":string="PicoPad3"
  in  "move properties":T2[](array[typedef])=[{"Tolerance [%]"=0.1, "Stepsize"=0.0001, "Invert Axis"=TRUE, "Invert Direction X"=FALSE, "Invert Direction Y"=TRUE, "enable feedback"=FALSE, "Set Centriod Target"=FALSE}, {"Tolerance [%]"=0.1, "Stepsize"=0.0001, "Invert Axis"=TRUE, "Invert Direction X"=FALSE, "Invert Direction Y"=TRUE, "enable feedback"=FALSE, "Set Centriod Target"=FALSE}, {"Tolerance [%]"=0.1, "Stepsize"=0.0001, "Invert Axis"=TRUE, "Invert Direction X"=FALSE, "Invert Direction Y"=TRUE, "enable feedback"=FALSE, "Set Centriod Target"=FALSE}, {"Tolerance [%]"=0.1, "Stepsize"=0.0001, "Invert Axis"=TRUE, "Invert Direction X"=FALSE, "Invert Direction Y"=TRUE, "enable feedback"=FALSE, "Set Centriod Target"=FALSE}, {"Tolerance [%]"=0.1, "Stepsize"=0.0001, "Invert Axis"=TRUE, "Invert Direction X"=FALSE, "Invert Direction Y"=TRUE, "enable feedback"=FALSE, "Set Centriod Target"=FALSE}, {"Tolerance [%]"=0.1, "Stepsize"=0.0001, "Invert Axis"=TRUE, "Invert Direction X"=FALSE, "Invert Direction Y"=TRUE, "enable feedback"=FALSE, "Set Centriod Target"=FALSE}, {"Tolerance [%]"=0.1, "Stepsize"=0.0001, "Invert Axis"=TRUE, "Invert Direction X"=FALSE, "Invert Direction Y"=TRUE, "enable feedback"=FALSE, "Set Centriod Target"=FALSE}, {"Tolerance [%]"=0.1, "Stepsize"=0.0001, "Invert Axis"=TRUE, "Invert Direction X"=FALSE, "Invert Direction Y"=TRUE, "enable feedback"=FALSE, "Set Centriod Target"=FALSE}, {"Tolerance [%]"=0.1, "Stepsize"=0.0001, "Invert Axis"=TRUE, "Invert Direction X"=FALSE, "Invert Direction Y"=TRUE, "enable feedback"=FALSE, "Set Centriod Target"=FALSE}, {"Tolerance [%]"=0.1, "Stepsize"=0.0001, "Invert Axis"=TRUE, "Invert Direction X"=FALSE, "Invert Direction Y"=TRUE, "enable feedback"=FALSE, "Set Centriod Target"=FALSE}, {"Tolerance [%]"=0.1, "Stepsize"=0.0001, "Invert Axis"=TRUE, "Invert Direction X"=FALSE, "Invert Direction Y"=TRUE, "enable feedback"=FALSE, "Set Centriod Target"=FALSE}, {"Tolerance [%]"=0.1, "Stepsize"=0.0001, "Invert Axis"=TRUE, "Invert Direction X"=FALSE, "Invert Direction Y"=TRUE, "enable feedback"=FALSE, "Set Centriod Target"=FALSE}, {"Tolerance [%]"=0.1, "Stepsize"=0.0001, "Invert Axis"=TRUE, "Invert Direction X"=FALSE, "Invert Direction Y"=TRUE, "enable feedback"=FALSE, "Set Centriod Target"=FALSE}]
  in  "Time":timestamp[][](array[timestamp])
  in  "Mean Size":dbl[][](array[numeric])
  in  "Size":dbl[][](array[numeric])
  in  "active CCDs":i32(listbox)=1
  in  "Offset Y":dbl[][](array[numeric])
  in  "Offset X":dbl[][](array[numeric])
  in  "Mean Centroid X":dbl[][](array[numeric])
  in  "Mean Centroid Y":dbl[][](array[numeric])
  in  "Centroid Y":dbl[][](array[numeric])
  in  "Centroid X":dbl[][](array[numeric])
  in  "GUIdevice 7":string="B2_TelLens1"
  in  "GUIdevice 6":string="B1_TelInput"
  in  "GUIdevice 5":string="L8_M10Leak"
  in  "GUIdevice 4":string="L7_TREXPass4"
  in  "GUIdevice 3":string="L6_TREXpass3"
  in  "GUIdevice 2":string="L5_TREXPass2"
  in  "insert tag":bool=TRUE
  in  "stop":bool
  in  "GUIdevice 1":string="L4_TREXpass1"
  out "tcp data event":T13
  out "error IO 2":errorcluster
  # "x [Tolerance]"
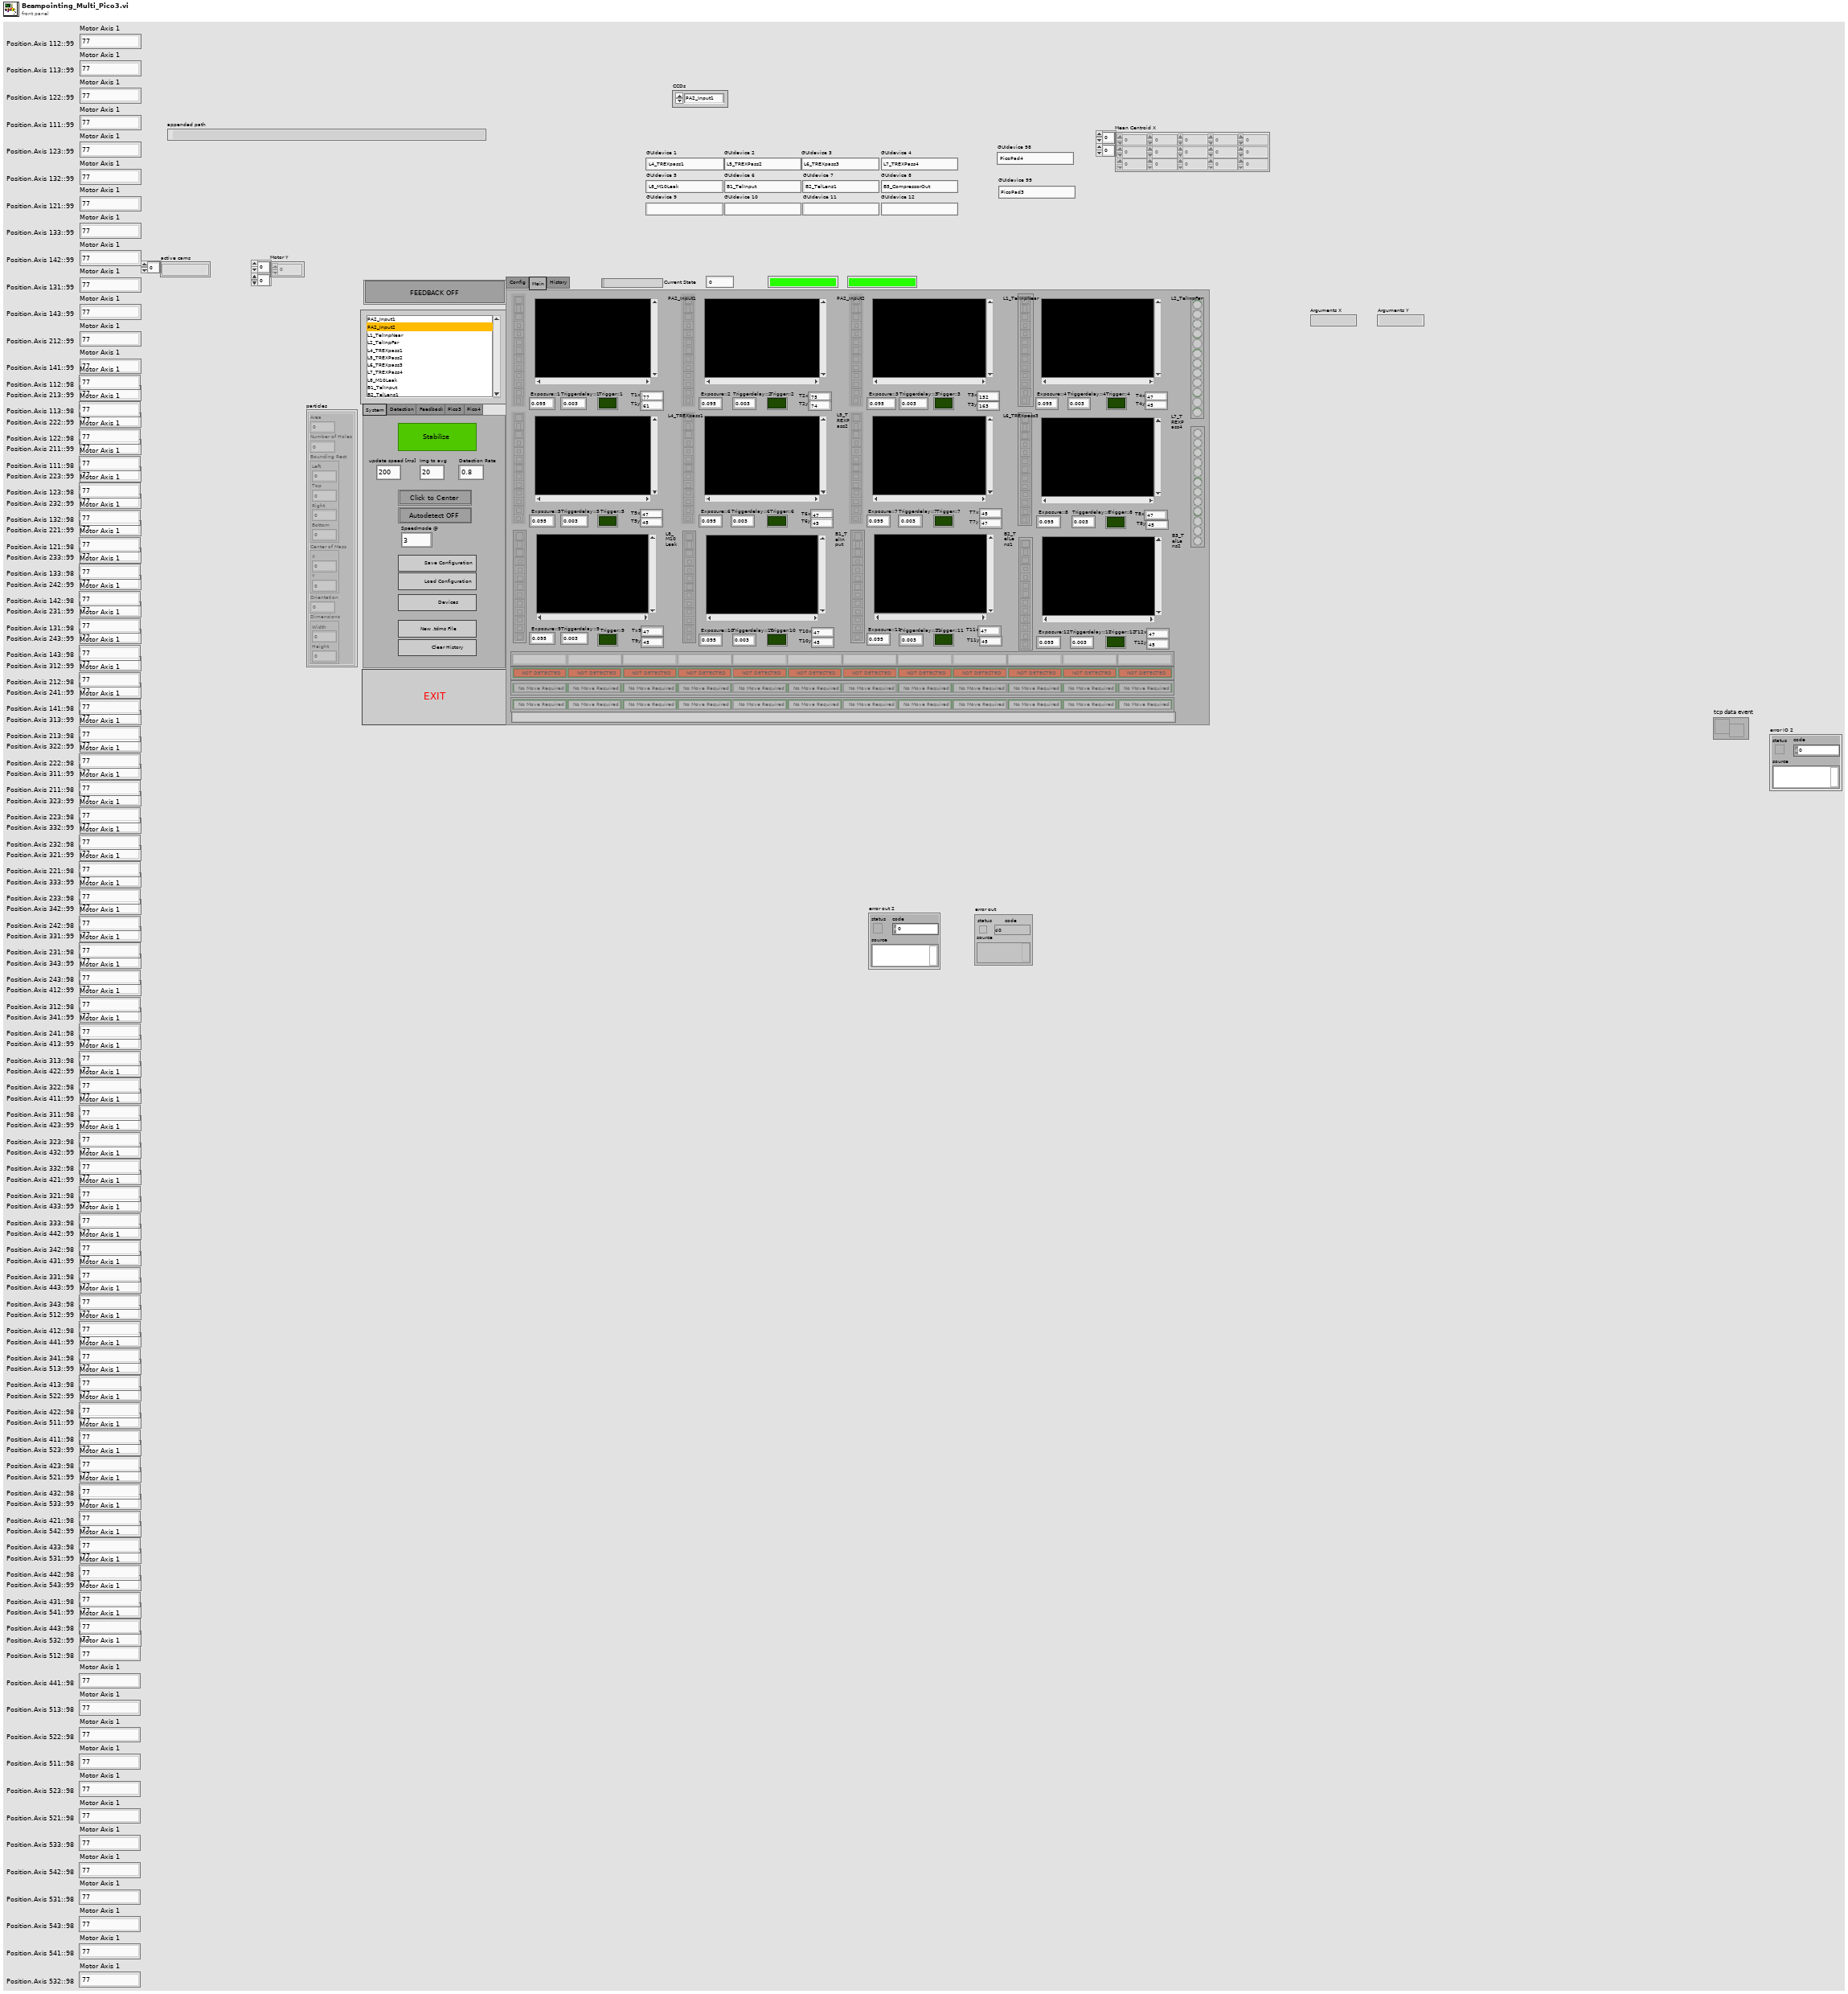
[diagram p1: front panel]
types:
  T1 = cluster{"Area":dbl, "Number of Holes":dbl, "Bounding Rect":cluster{"Left":dbl, "Top":dbl, "Right":dbl, "Bottom":dbl}, "Center of Mass":cluster{"X":dbl, "Y":dbl}, "Orientation":dbl, "Dimensions":cluster{"Width":dbl, "Height":dbl}}[]
  T2 = typedef "move.ctl" = cluster{"Tolerance [%]":dbl, "Stepsize":dbl, "Invert Axis":bool, "Invert Direction X":bool, "Invert Direction Y":bool, "enable feedback":bool, "Set Centriod Target":bool}
  T3 = typedef "beam detection.ctl" = cluster{"Filter":u16, "Filter Para":cluster{"X Size":i32, "Y Size":i32, "% Tolerance":i32}, "detection method":i32, "smal para":cluster{"Measurement Parameter":T4, "Range Lower Value":dbl, "Range Upper Value":dbl, "Range":bool, "Measurement Type":bool}[], "Remove small Objects":bool, "Restrict to round Objects":bool}
  T4 = typedef "Particle Parameters" = i32
  T5 = cluster{"CCDs":string[], "move properties":T2[], "detection para":T3[], "thresholds":cluster{"Lower value":sgl, "Upper value":sgl}[], "Value":cluster{"Motor CCD 1":u16, "Motor CCD 2":u16, "Motor CCD 3":u16, "Motor CCD 4":u16, "Motor CCD 5":u16, "Motor CCD 6":u16, "Motor CCD 7":u16, "Motor CCD 8":u16, "Motor CCD 9":u16, "Motor CCD 10":u16, "Motor CCD 11":u16, "Motor CCD 12":u16}}
  T6 = cluster{"Left":dbl, "Top":dbl, "Right":dbl, "Bottom":dbl}[]
  T7 = cluster{"Motor CCD 1":u16, "Motor CCD 2":u16, "Motor CCD 3":u16, "Motor CCD 4":u16, "Motor CCD 5":u16, "Motor CCD 6":u16, "Motor CCD 7":u16, "Motor CCD 8":u16, "Motor CCD 9":u16, "Motor CCD 10":u16, "Motor CCD 11":u16, "Motor CCD 12":u16}
  T8 = cluster{"[0]":string, "[1]":string, "[2]":string, "[3]":string, "[4]":string, "[5]":string, "[6]":string, "[7]":string, "[8]":string, "[8] 2":string, "[8] 3":string, "[8] 4":string}
  T9 = typedef "IMAQ Image.ctl" = refnum<image>
  T10 = cluster{"Area":dbl, "Number of Holes":dbl, "Bounding Rect":cluster{"Left":dbl, "Top":dbl, "Right":dbl, "Bottom":dbl}, "Center of Mass":cluster{"X":dbl, "Y":dbl}, "Orientation":dbl, "Dimensions":cluster{"Width":dbl, "Height":dbl}}[][]
  T11 = enum32{"System", "Detection", "Feedback", "Pico3", "Pico4"}
  T12 = cluster{"Ref X":refnum<vi>, "Ref Y":refnum<vi>}[]
  T13 = typedef "tcp_new_data_event.ctl" = refnum<user-event>
  T14 = typedef "tcp new data cluster.ctl" = cluster{"EventEnum":enum16{"new data", "connection status update"}, "Device name":string}
  T15 = cluster{"Left":i32, "Top":i32, "Right":i32, "Bottom":i32}
  T16 = enum32{"invalid app kind", "Development System", "Run Time System", "Student Edition", "Embedded LabVIEW", "Evaluation", "Custom"}
  T17 = enum16{"open", "open or create", "create or replace", "create", "open (read-only)"}
  T18 = enum32{"Invalid", "Standard", "Closed", "Hidden", "Minimized", "Maximized"}
  T19 = enum16{"open", "replace", "create", "open or create", "replace or create", "replace or create with confirmation"}
  T20 = typedef "Image Type" = u32
  T21 = cluster{"[0]":string, "[1]":string, "[2]":string, "[3]":string, "[4]":string, "[5]":string, "[6]":string, "[7]":string, "[8]":string, "[9]":string, "[10]":string, "[11]":string}
  T22 = cluster{"Target.X::1":refnum<vi>, "Target.Y::1":refnum<vi>}
  T23 = cluster{"Target.X::2":refnum<vi>, "Target.Y::2":refnum<vi>}
  T24 = cluster{"Target.X::3":refnum<vi>, "Target.Y::3":refnum<vi>}
  T25 = cluster{"Target.X::4":refnum<vi>, "Target.Y::4":refnum<vi>}
  T26 = cluster{"Target.X::5":refnum<vi>, "Target.Y::5":refnum<vi>}
  T27 = cluster{"Target.X::6":refnum<vi>, "Target.Y::6":refnum<vi>}
  T28 = cluster{"Target.X::7":refnum<vi>, "Target.Y::7":refnum<vi>}
  T29 = cluster{"Target.X::8":refnum<vi>, "Target.Y::8":refnum<vi>}
  T30 = cluster{"Target.X::12":refnum<vi>, "Target.Y::12":refnum<vi>}
  T31 = cluster{"Target.X::9":refnum<vi>, "Target.Y::9":refnum<vi>}
  T32 = cluster{"Target.X::10":refnum<vi>, "Target.Y::10":refnum<vi>}
  T33 = cluster{"Target.X::11":refnum<vi>, "Target.Y::11":refnum<vi>}
  T34 = cluster{"Target.X::12":refnum<vi>, "Target.Y::12":refnum<vi>}[]
  T35 = cluster{"Left":dbl, "Top":dbl, "Right":dbl, "Bottom":dbl}
  T36 = cluster{"Core":cluster{"Current VI Reference":refnum<vi>, "Close Panel on Exit?":bool}, "detection para":T3[], "thresholds":cluster{"Lower value":sgl, "Upper value":sgl}[], "Centroid X":dbl[][], "Centroid Y":dbl[][], "img to avg":i32, "Mean Centroid X":dbl[][], "Mean Centroid Y":dbl[][], "Offset X":dbl[][], "Offset Y":dbl[][], "Offset X stats ":dbl[][], "Offset Y stats ":dbl[][], "Size":dbl[][], "Mean Size":dbl[][], "Time":timestamp[][], "move properties":T2[], "active axis refs 2":cluster{"Ref X":refnum<vi>, "Ref Y":refnum<vi>}[], "active ccd":i32, "Feedback global":bool, "Motor X":dbl[][], "Motor Y":dbl[][], "active cams":string[], "Data Value Reference out":refnum<k34>, "detected":bool[], "speedmode X":bool[], "speedmode Y":bool[]}
  T37 = typedef "DialogType.ctl" = u16
  T38 = cluster{"Current VI Reference":refnum<vi>, "Close Panel on Exit?":bool}
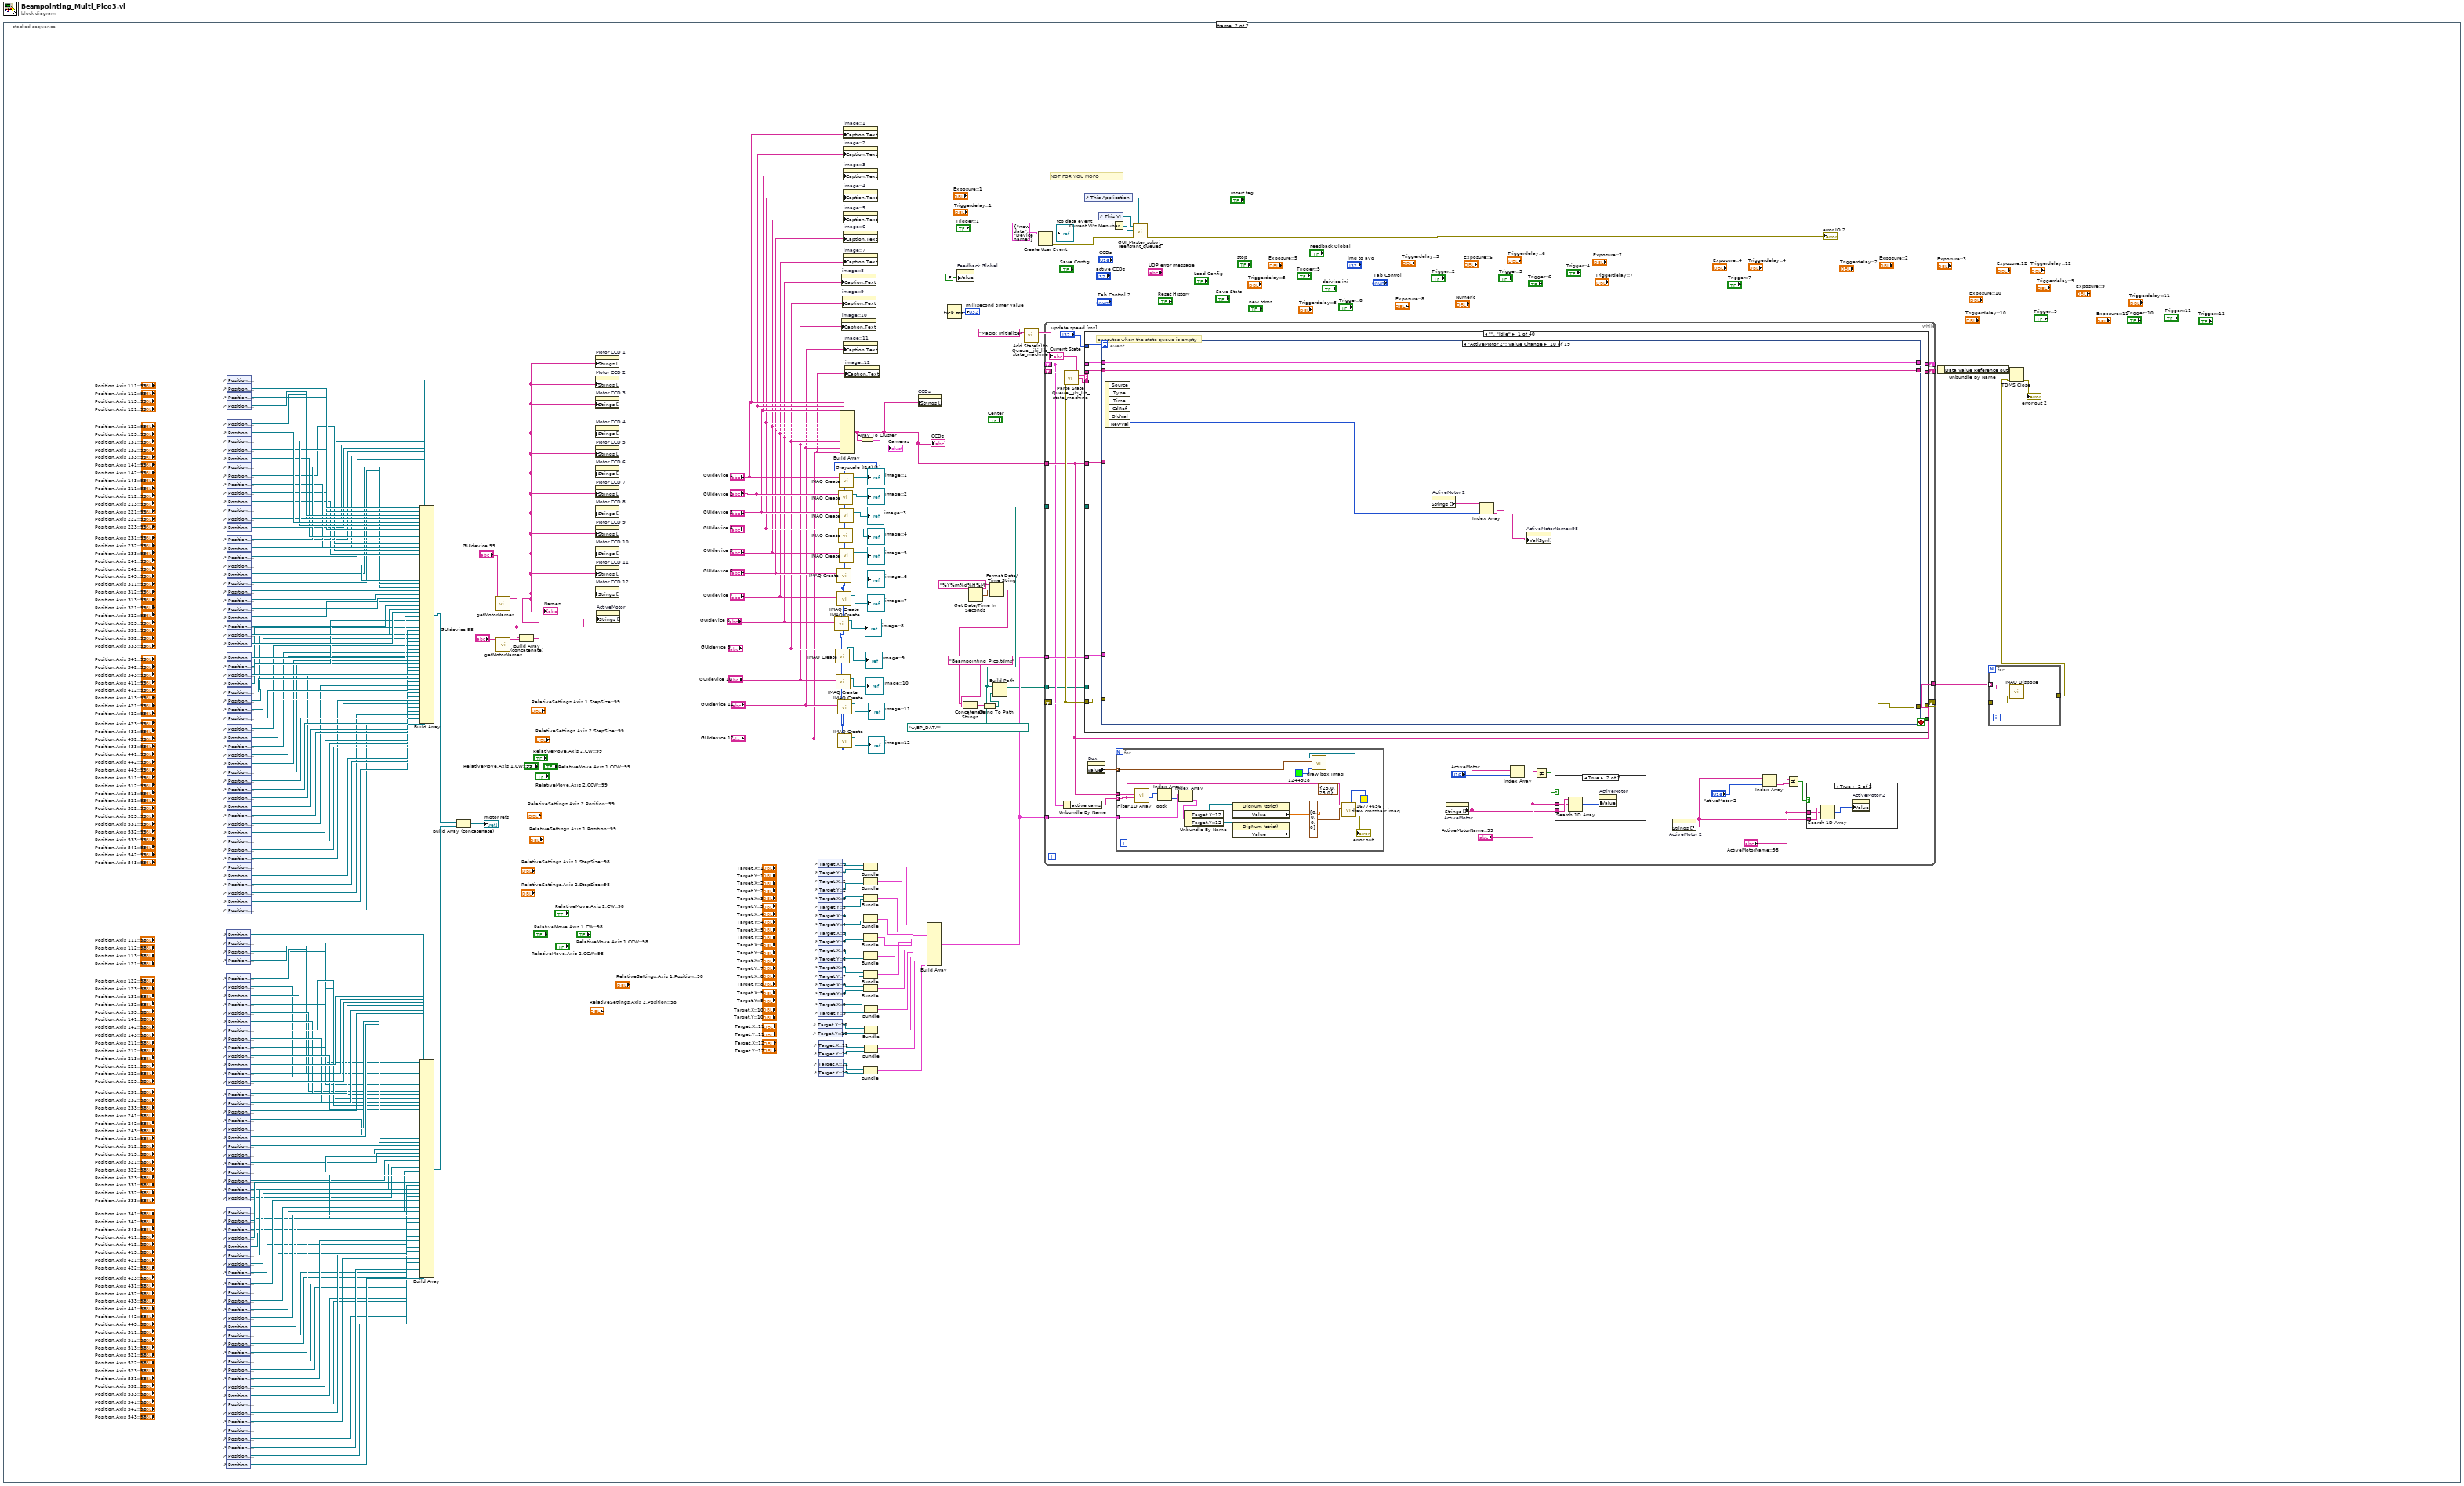
[diagram p0: block diagram]
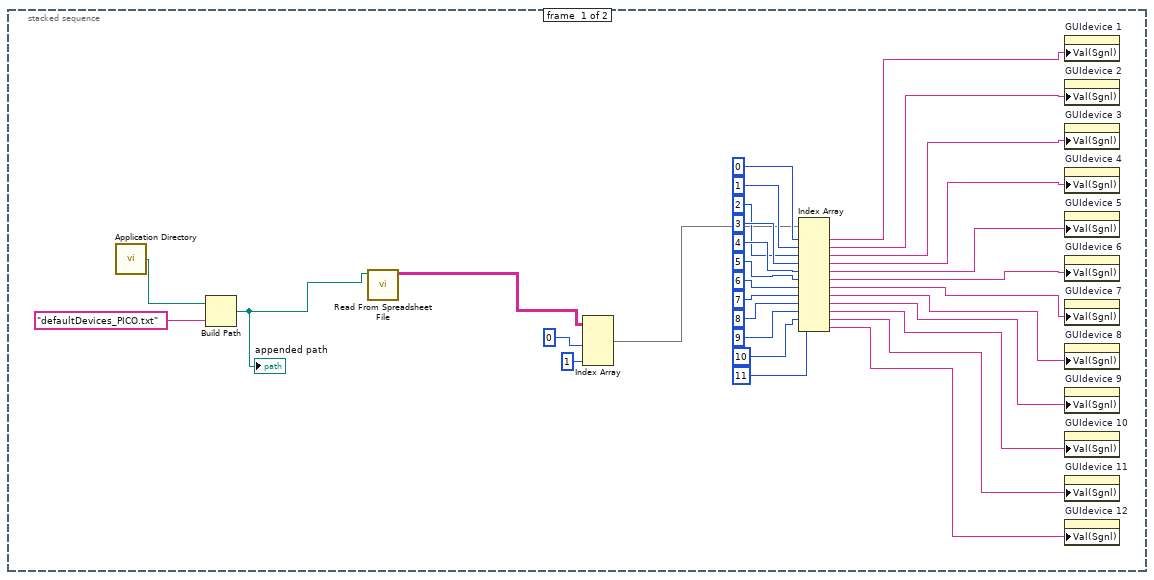
[diagram p2: hidden frame]
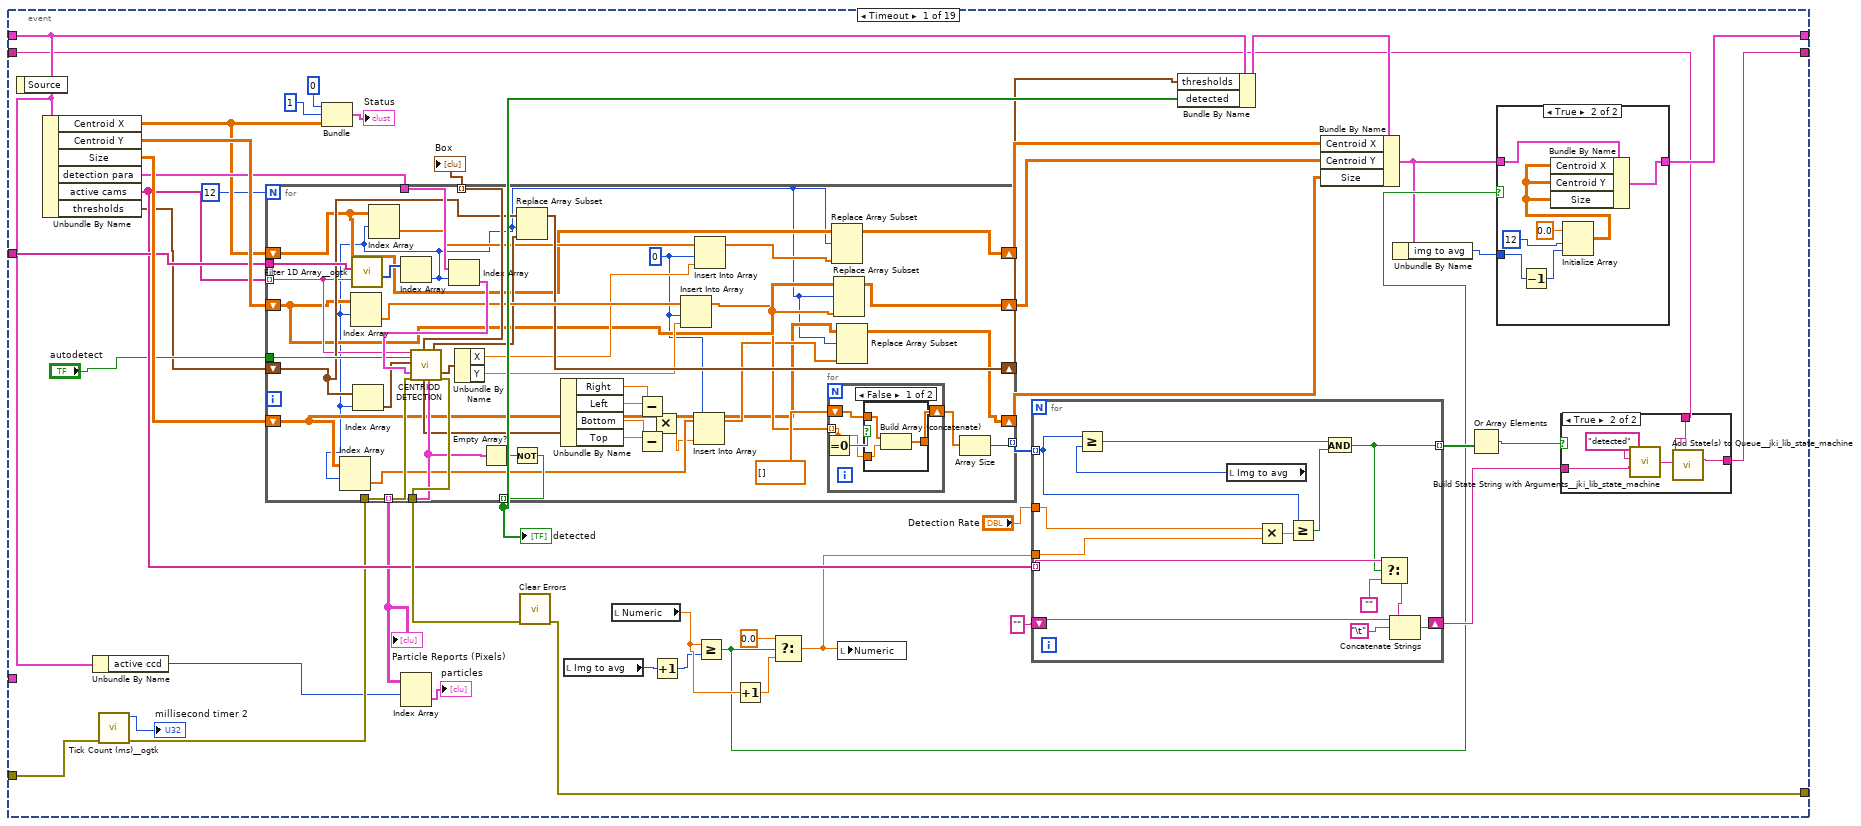
[diagram p5: hidden frame]
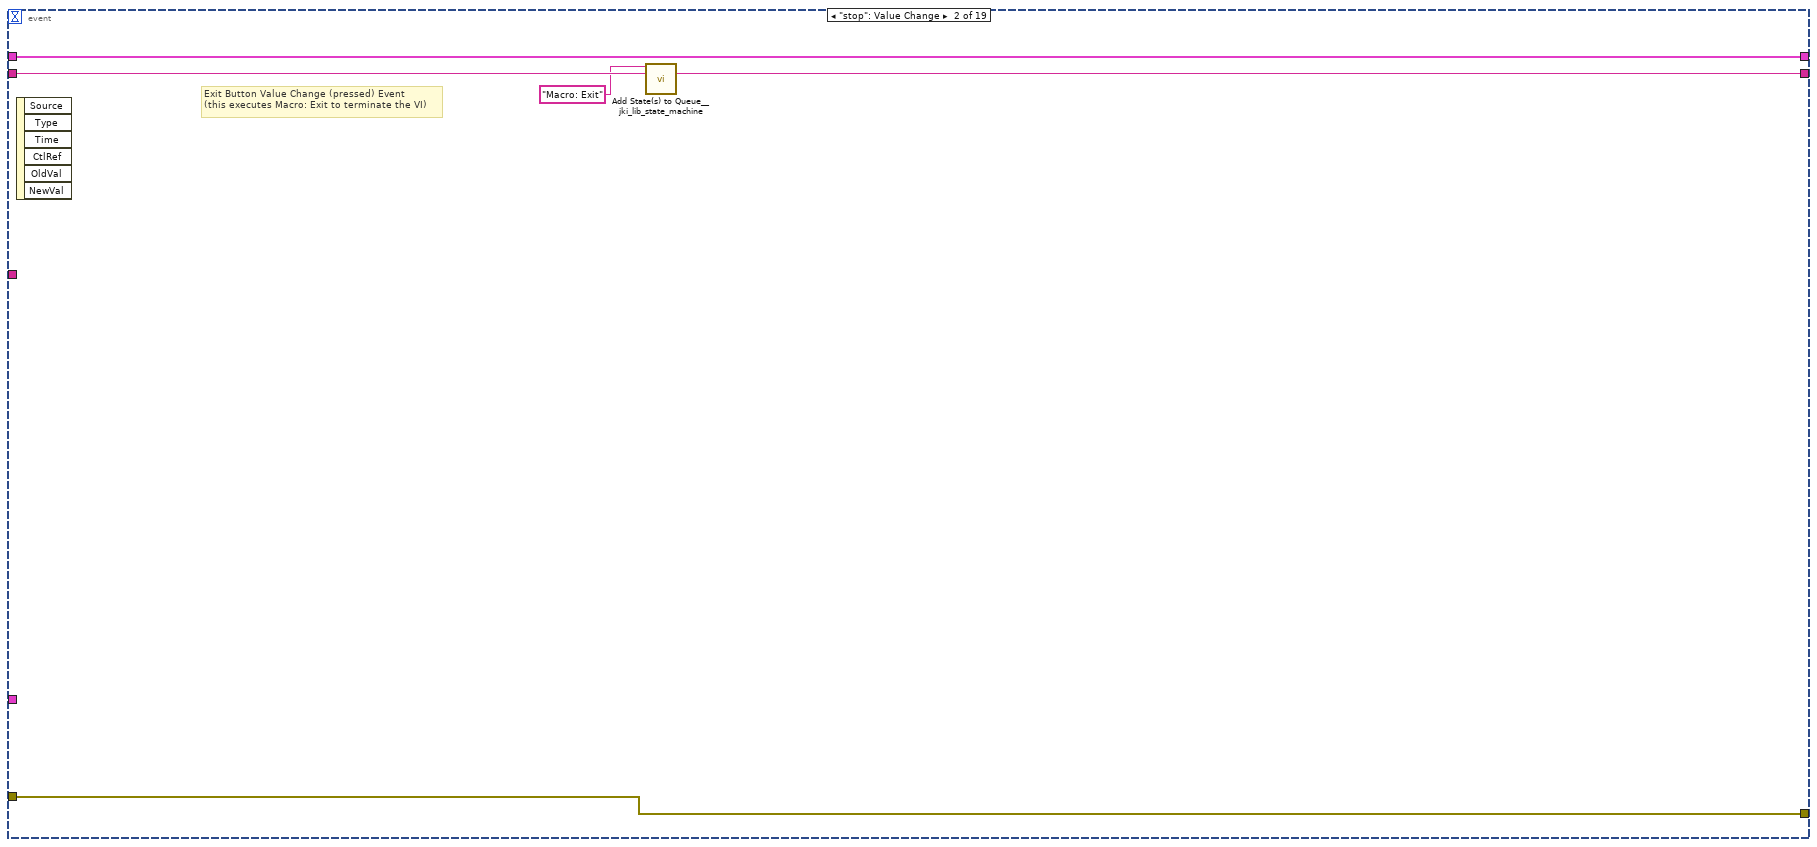
[diagram p9: hidden frame]
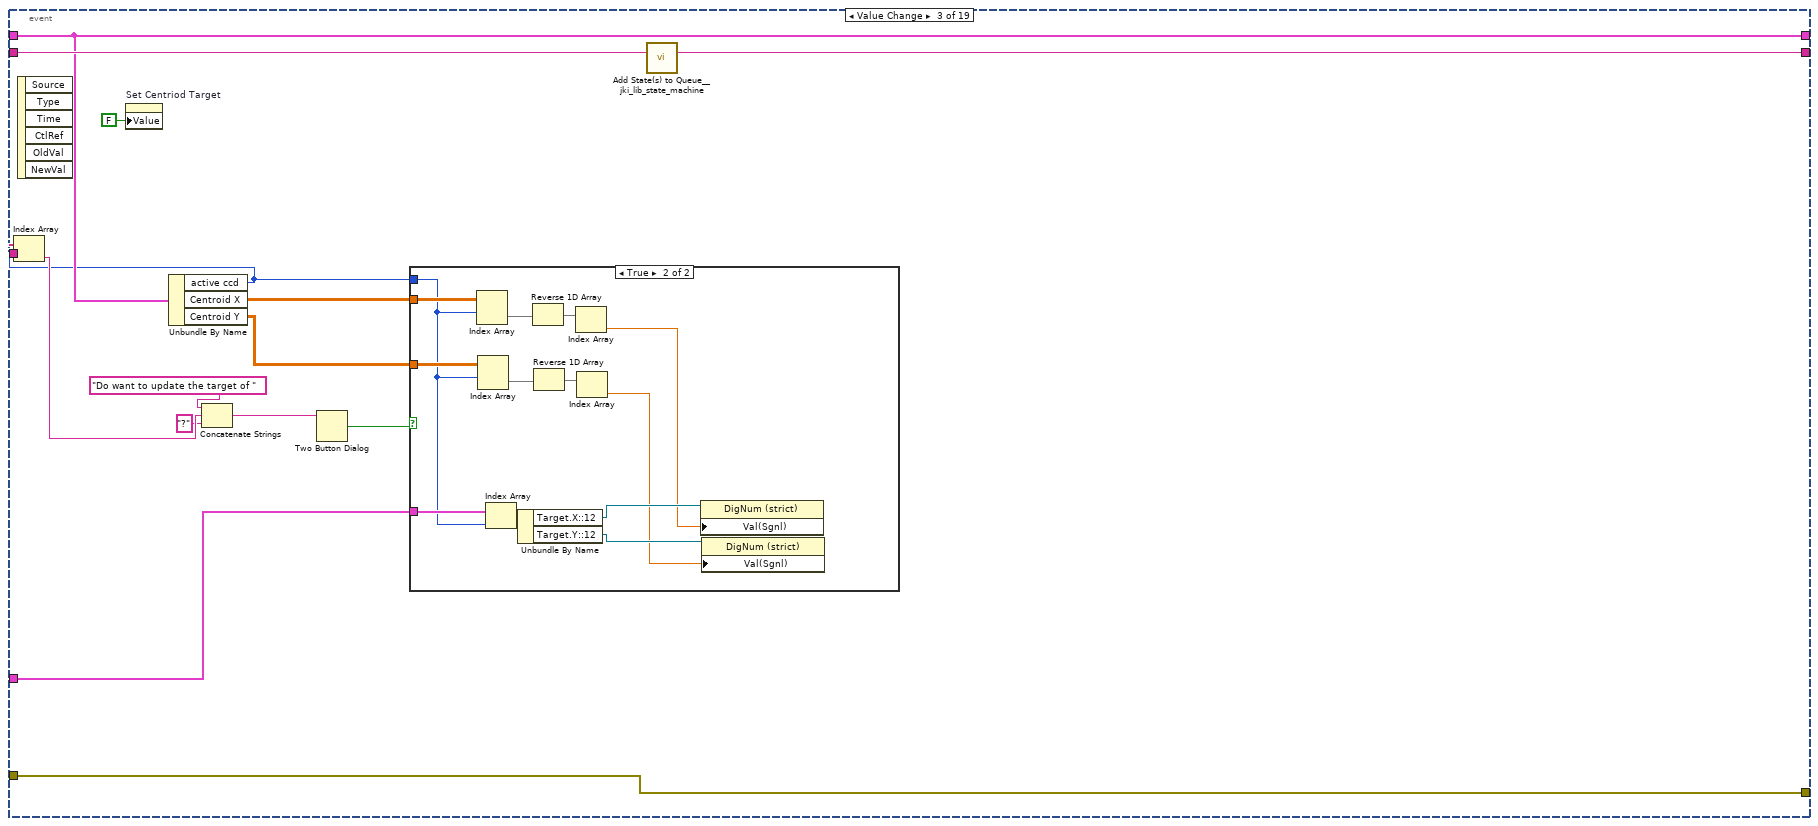
[diagram p10: hidden frame]
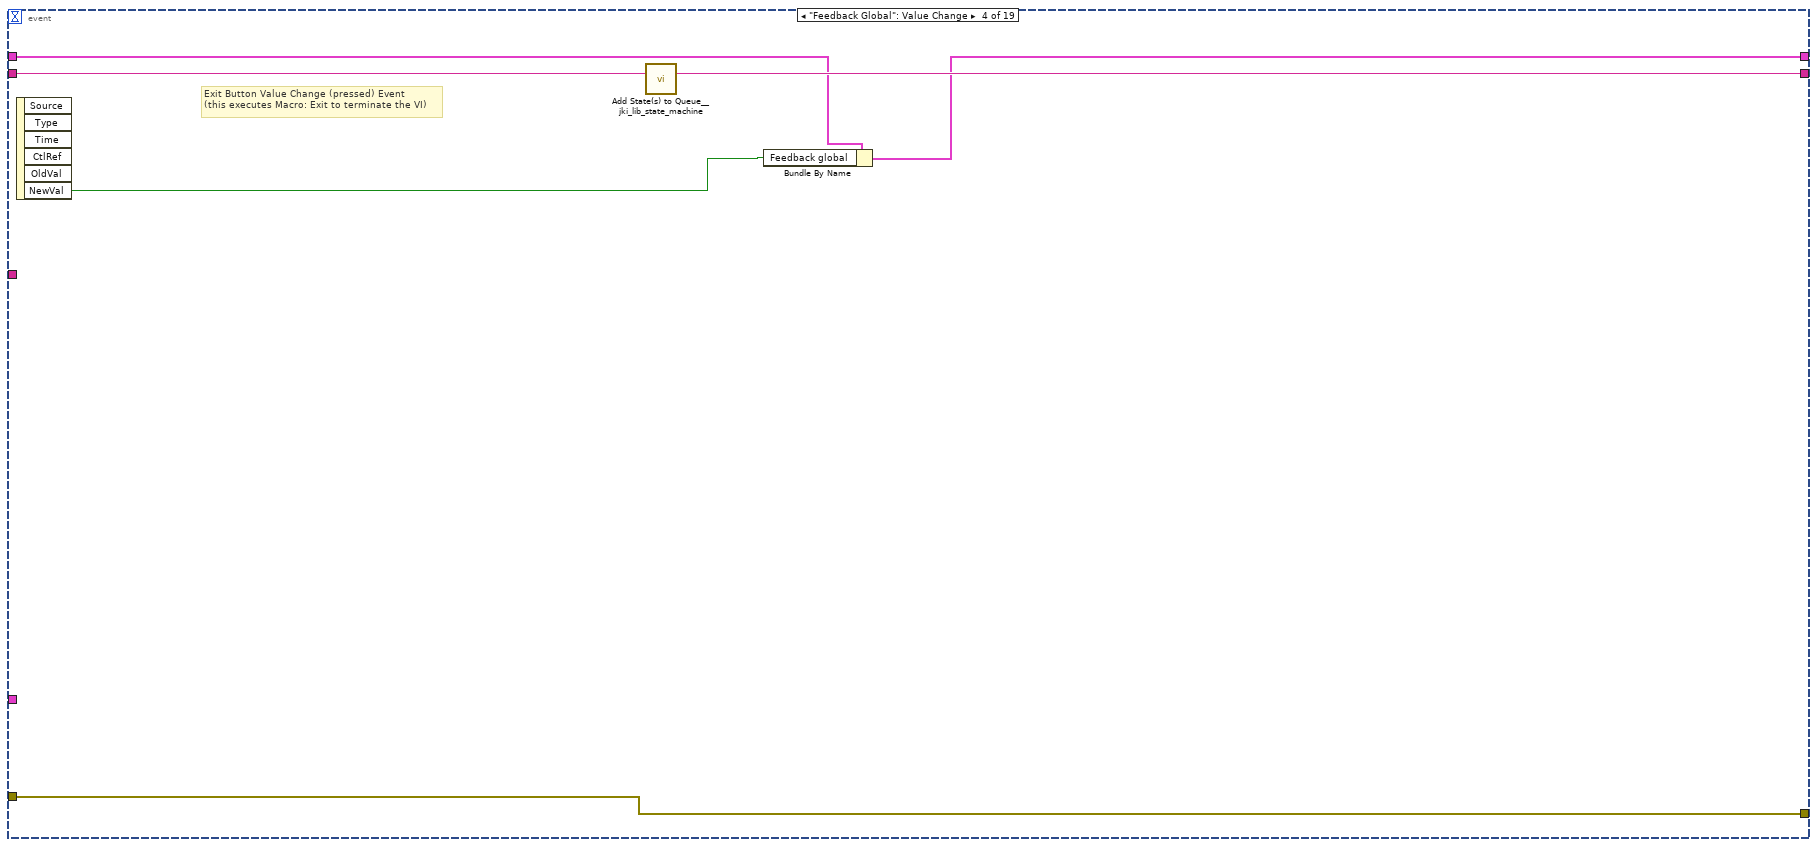
[diagram p12: hidden frame]
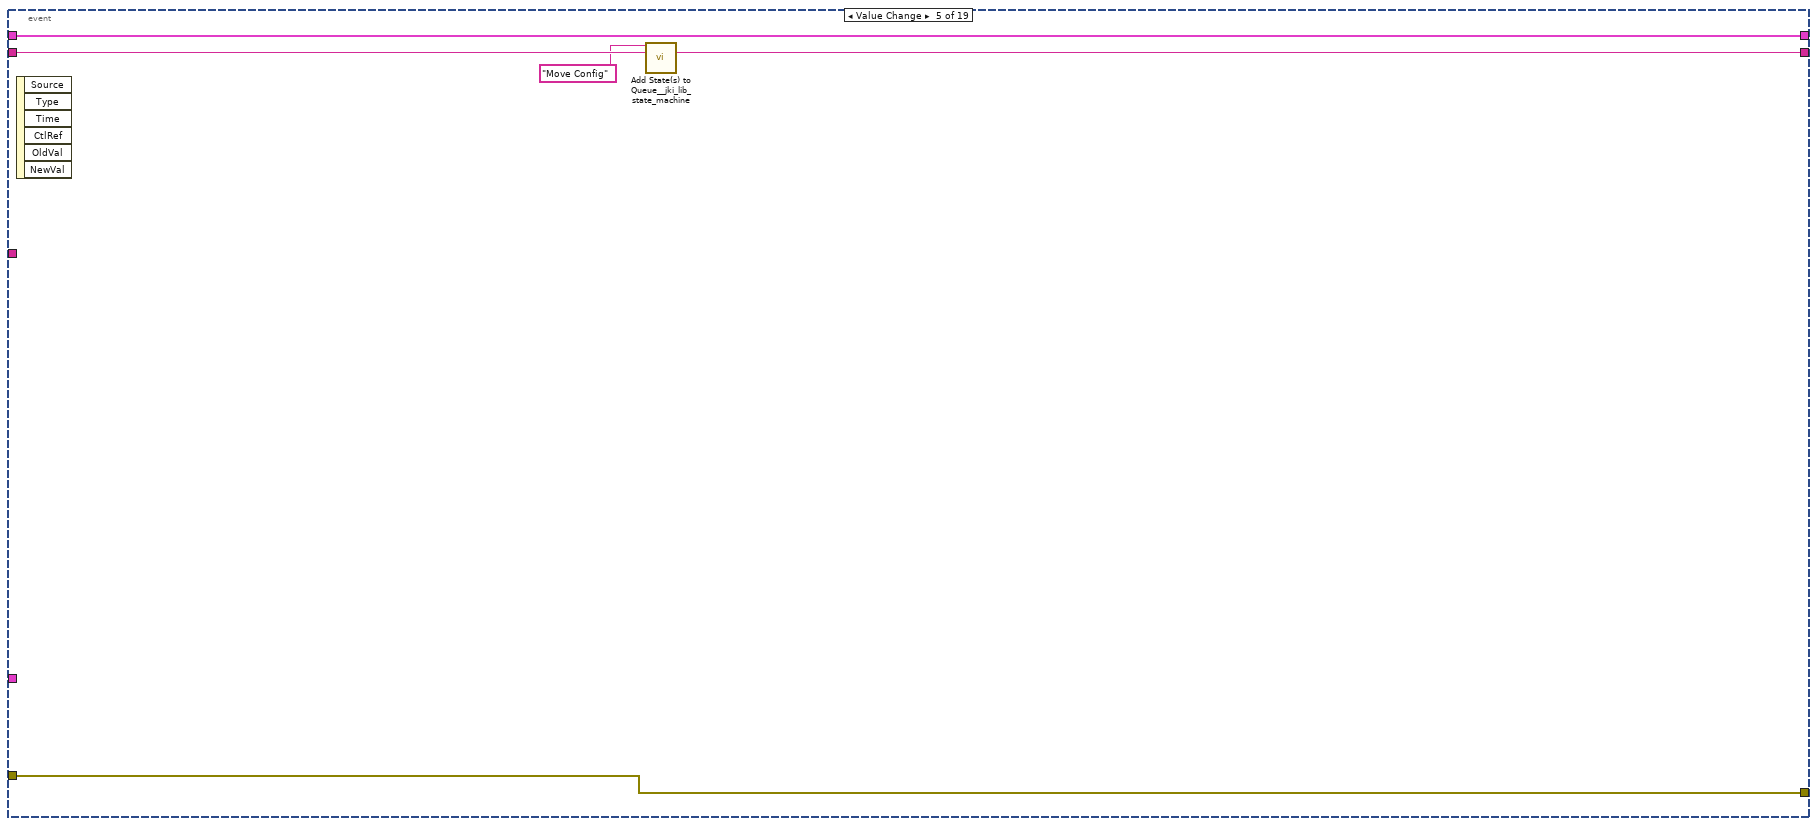
[diagram p13: hidden frame]
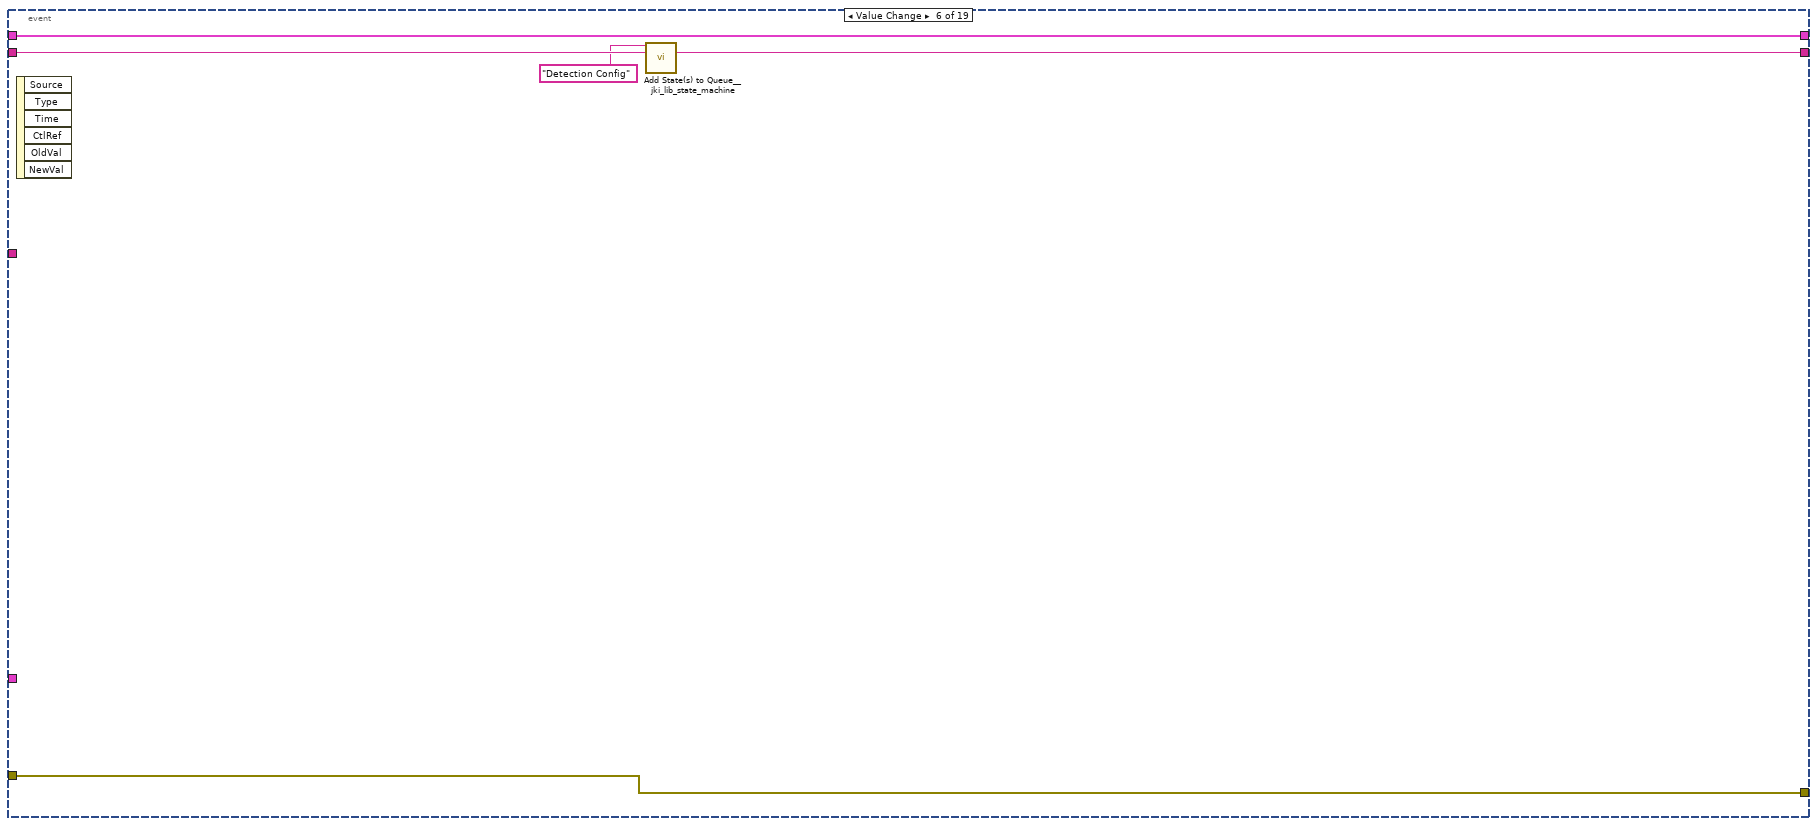
[diagram p14: hidden frame]
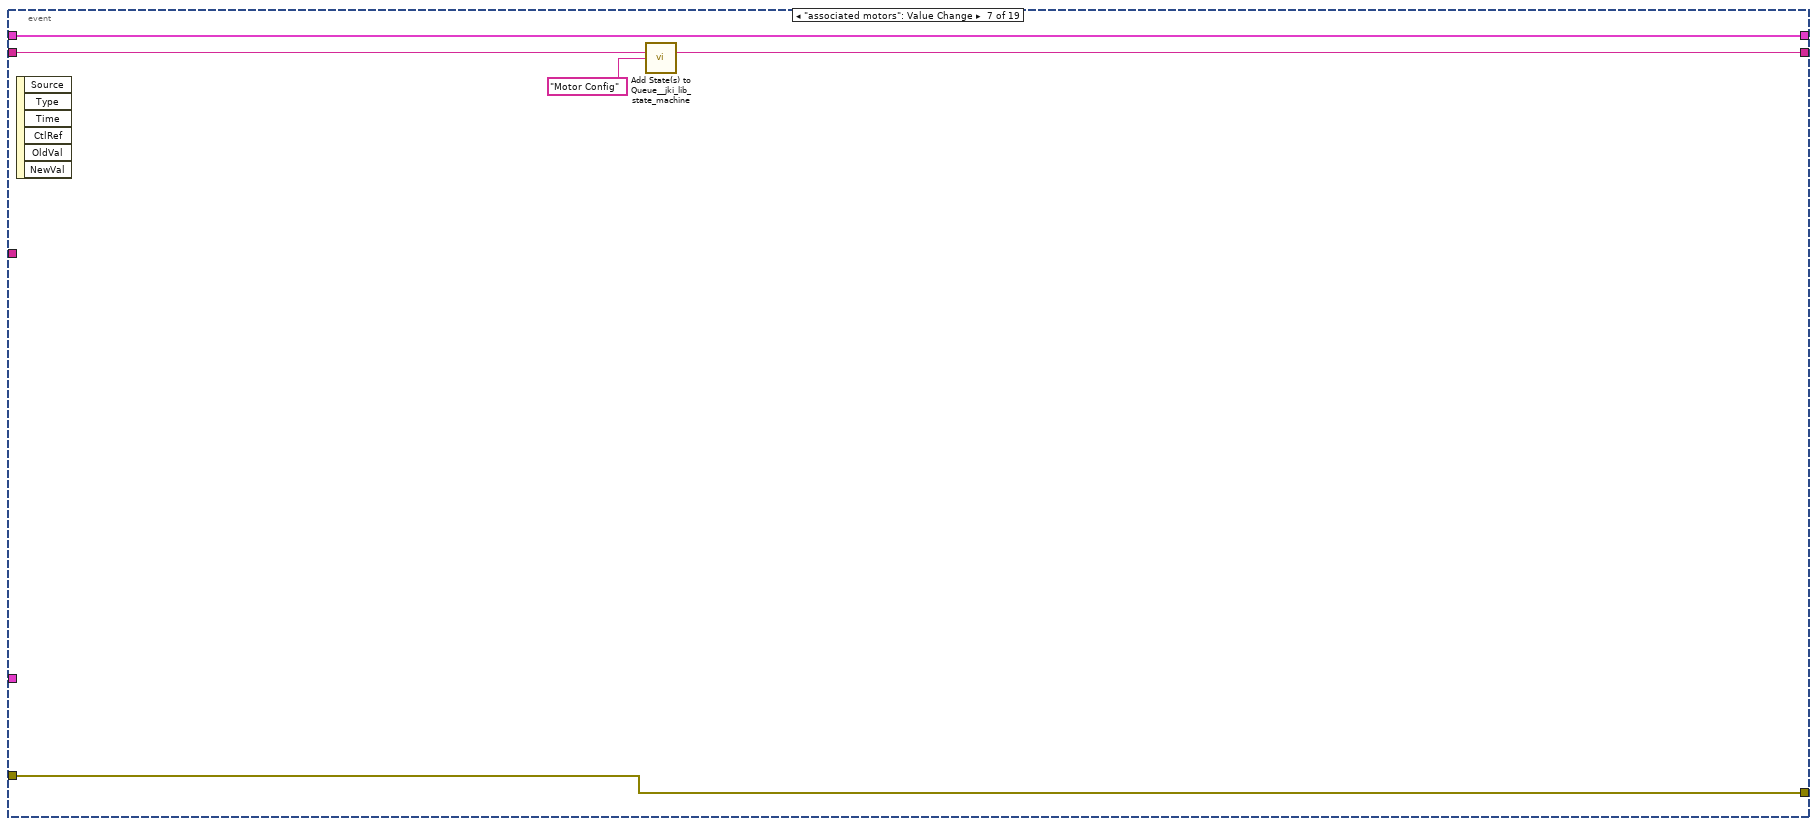
[diagram p15: hidden frame]
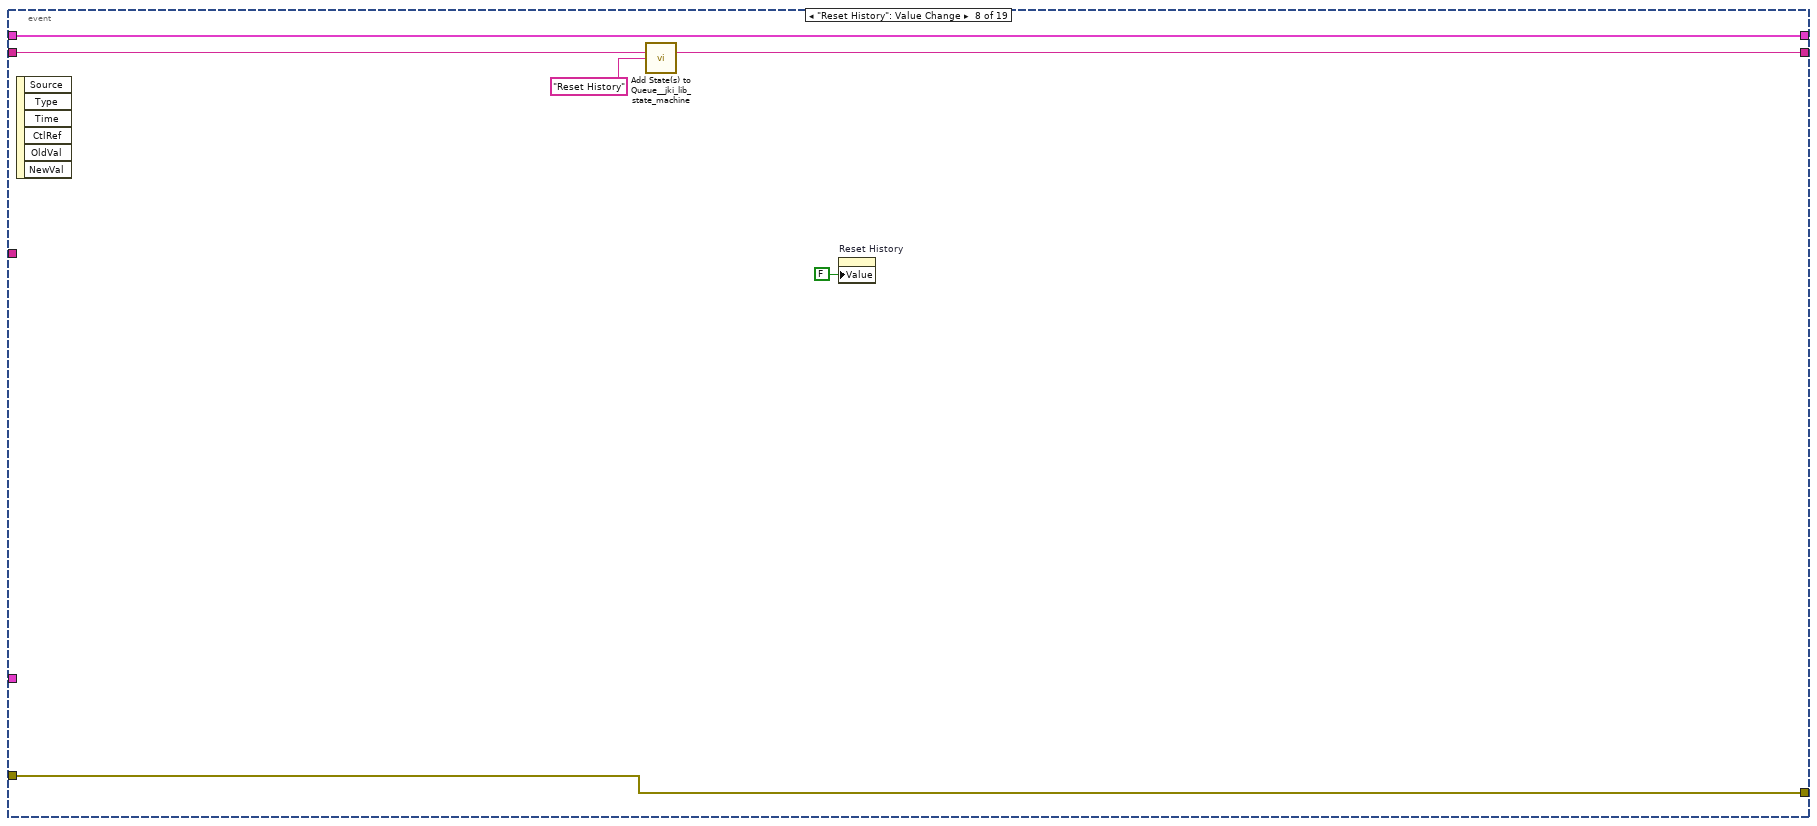
[diagram p16: hidden frame]
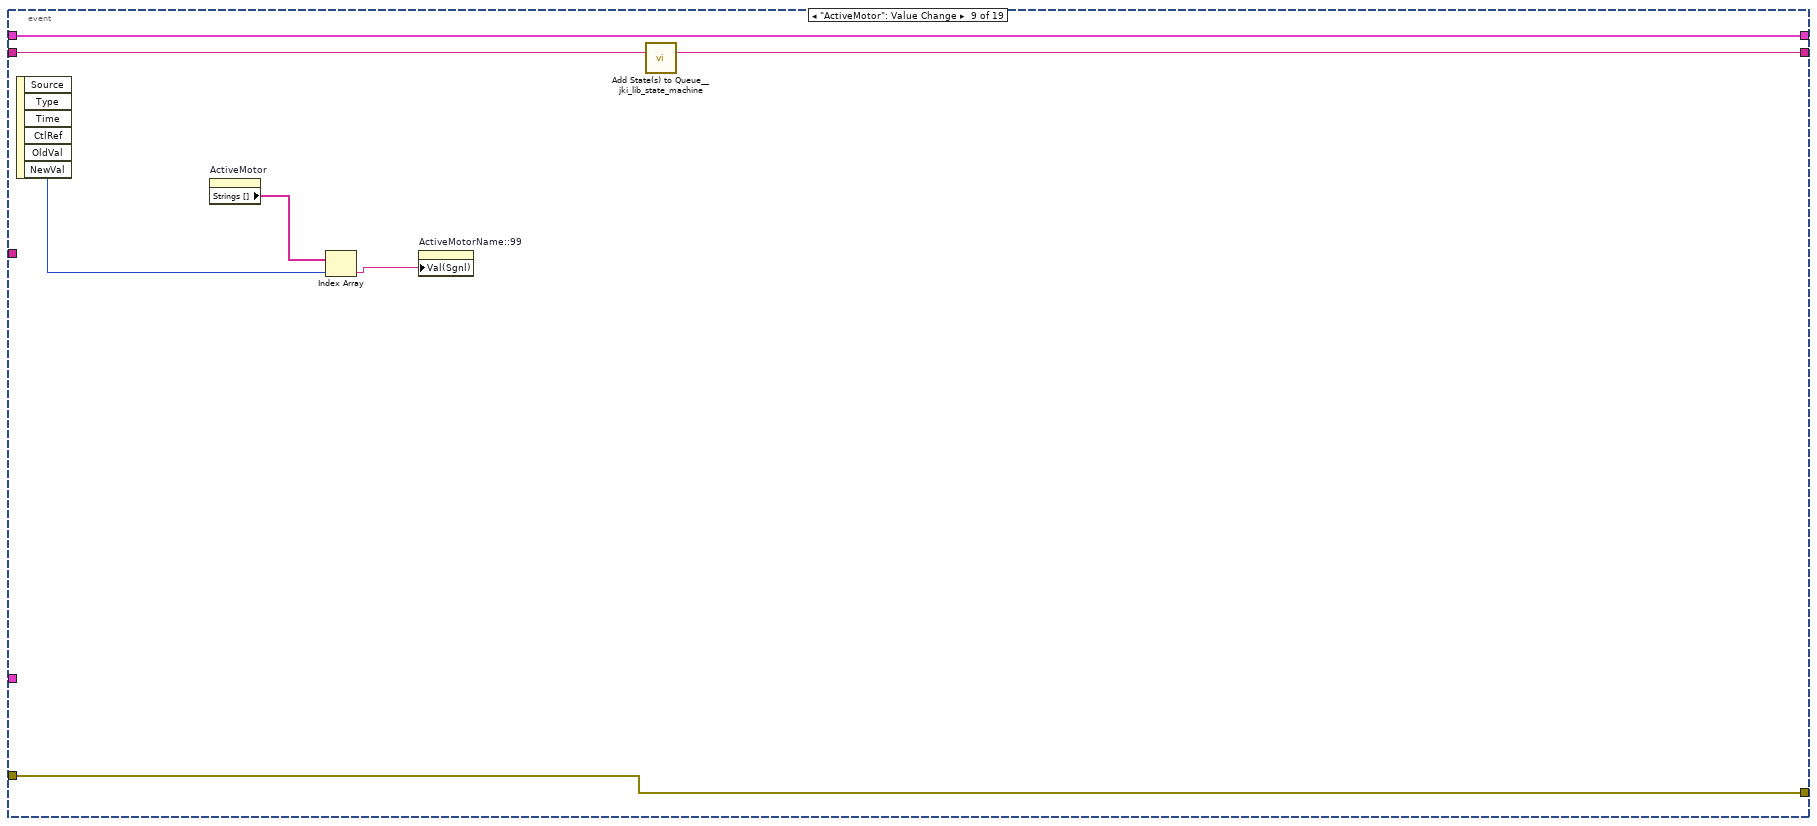
[diagram p17: hidden frame]
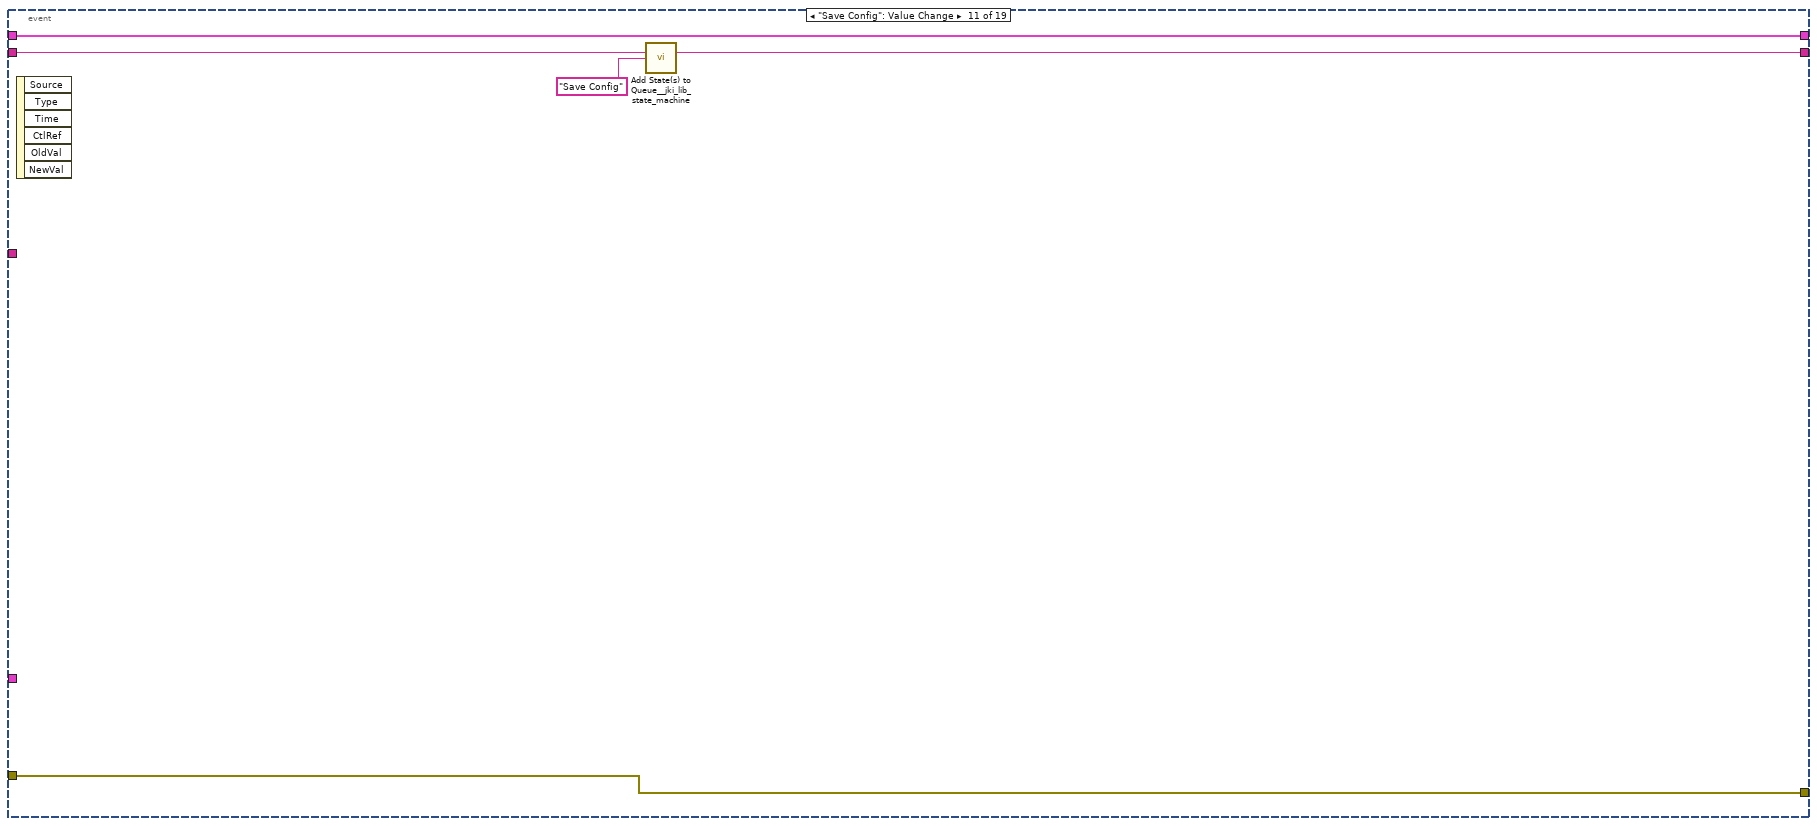
[diagram p18: hidden frame]
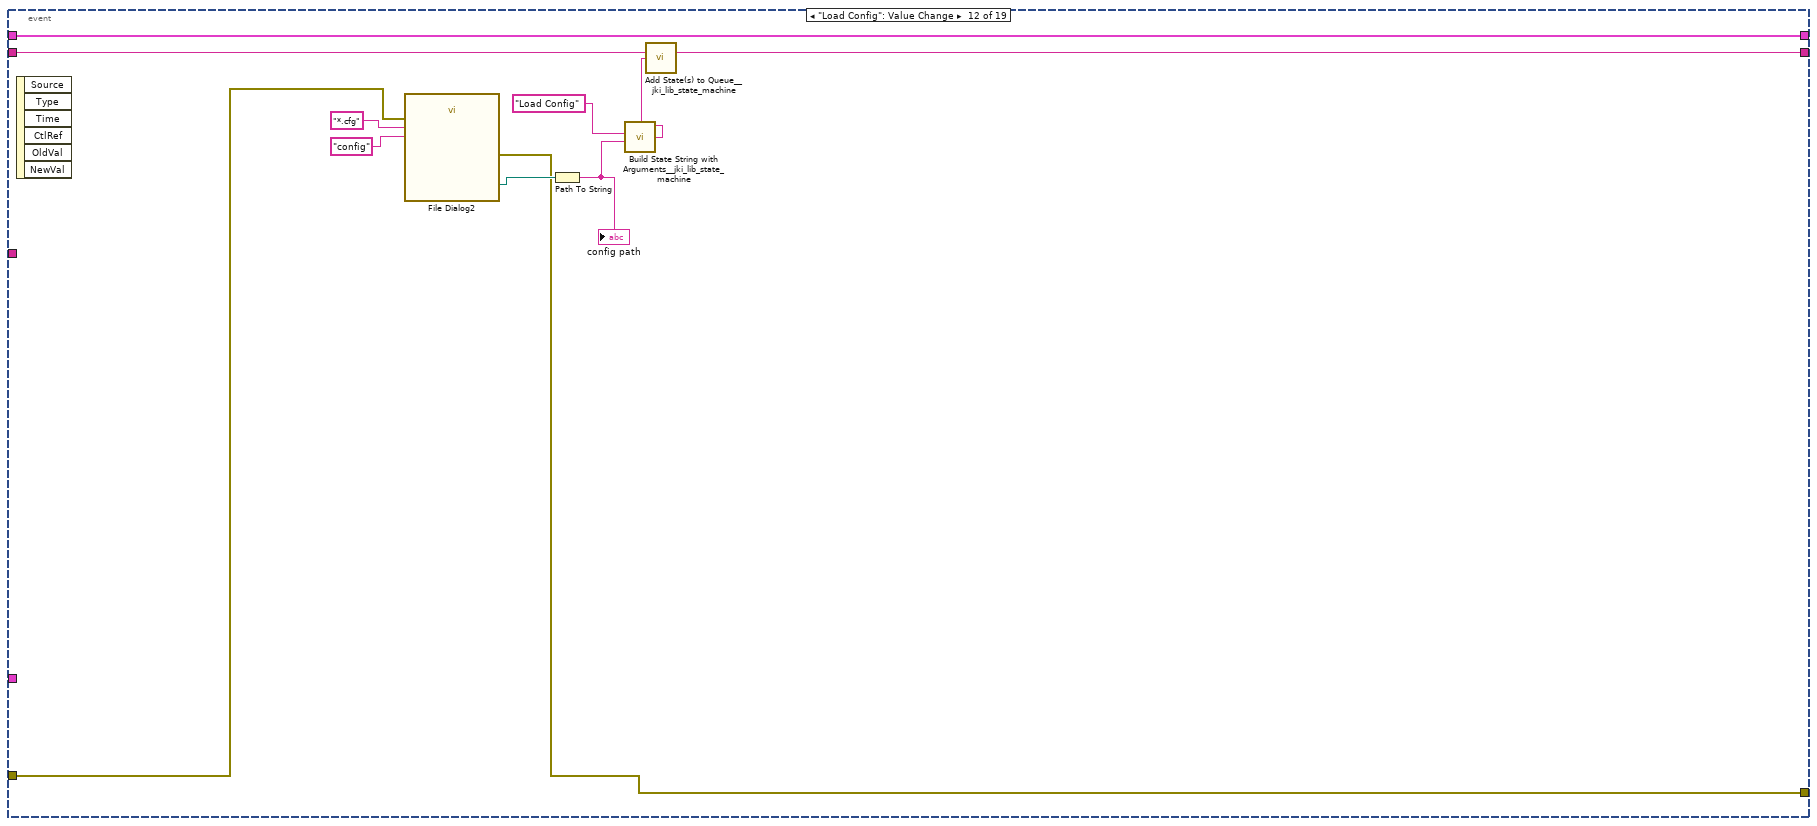
[diagram p19: hidden frame]
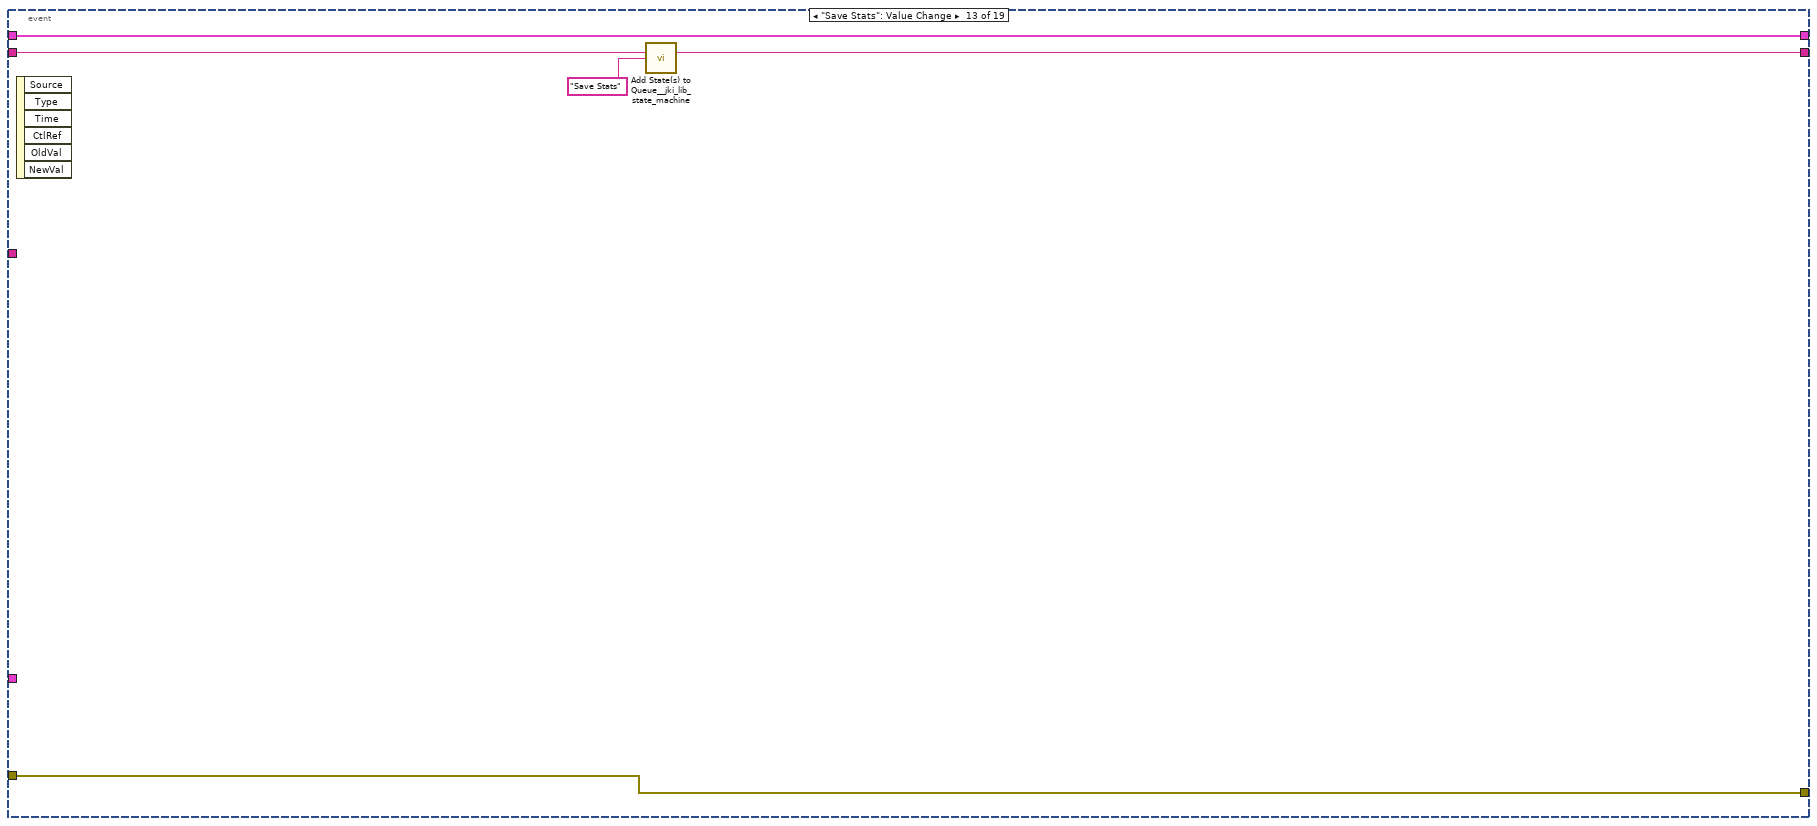
[diagram p20: hidden frame]
diagram:
  n1 = stacked-sequence {
    frame #0 {
      n2 = call <vilib>:"Application Directory.vi"() -> ("Application Directory"=w13:path)
      n3 = Build Path(base path=w13, name or relative path="defaultDevices_PICO.txt") -> (appended path=w15:path)
      "appended path" <- w15
      n4 = call-poly <vilib>:"Read From Spreadsheet File.vi"("file path (dialog if empty)"=w15) -> ("all rows"=w16:string[][])  [unwired: 6 in, 4 out]
      n5 = Index Array(array=w16, index (col) #1=0 ("disabled index (col)"), index (col) #2=1 ("index (col)")) -> (element #1=w19:string[])  [unwired: 2 in, 1 out]
      n6 = Index Array(array=w19, index #1=0 ("index"), index #2=1 ("index"), index #3=2 ("index"), index #4=3 ("index"), index #5=4 ("index"), index #6=5 ("index"), index #7=6 ("index"), index #8=7 ("index"), index #9=8 ("index"), index #10=9 ("index"), index #11=10 ("index"), index #12=11 ("index")) -> (element #1=w12:string, element #2=w11:string, element #3=w10:string, element #4=w9:string, element #5=w8:string, element #6=w7:string, element #7=w6:string, element #8=w5:string, element #9=w4:string, element #10=w3:string, element #11=w2:string, element #12=w1:string)
      n7 = property on="GUIdevice 1" class="Str"("Val(Sgnl)"=w12) -> ()  [unwired: 2 in, 2 out]
      n8 = property on="GUIdevice 2" class="Str"("Val(Sgnl)"=w11) -> ()  [unwired: 2 in, 2 out]
      n9 = property on="GUIdevice 3" class="Str"("Val(Sgnl)"=w10) -> ()  [unwired: 2 in, 2 out]
      n10 = property on="GUIdevice 4" class="Str"("Val(Sgnl)"=w9) -> ()  [unwired: 2 in, 2 out]
      n11 = property on="GUIdevice 5" class="Str"("Val(Sgnl)"=w8) -> ()  [unwired: 2 in, 2 out]
      n12 = property on="GUIdevice 6" class="Str"("Val(Sgnl)"=w7) -> ()  [unwired: 2 in, 2 out]
      n13 = property on="GUIdevice 7" class="Str"("Val(Sgnl)"=w6) -> ()  [unwired: 2 in, 2 out]
      n14 = property on="GUIdevice 8" class="Str"("Val(Sgnl)"=w5) -> ()  [unwired: 2 in, 2 out]
      n15 = property on="GUIdevice 9" class="Str"("Val(Sgnl)"=w4) -> ()  [unwired: 2 in, 2 out]
      n16 = property on="GUIdevice 10" class="Str"("Val(Sgnl)"=w3) -> ()  [unwired: 2 in, 2 out]
      n17 = property on="GUIdevice 11" class="Str"("Val(Sgnl)"=w2) -> ()  [unwired: 2 in, 2 out]
      n18 = property on="GUIdevice 12" class="Str"("Val(Sgnl)"=w1) -> ()  [unwired: 2 in, 2 out]
    }
    frame #1 {
      w32 = path "w:/BP_DATA" ("base path")
      w104 = T20 1 items=["Grayscale (U8)", "Grayscale (I16)", "Grayscale (SGL)", "Complex (CSG)", "RGB (U32)", "HSL (U32)", "RGB (U64)", "Grayscale (U16)"] ("Image Type")
      # "NOT FOR YOU MOFO"
      n19 = control-ref of="Position.Axis 111::98"() -> (w41:refnum<vi>)
      n20 = control-ref of="Position.Axis 112::98"() -> (w42:refnum<vi>)
      n21 = control-ref of="Position.Axis 113::98"() -> (w43:refnum<vi>)
      n22 = control-ref of="Position.Axis 121::98"() -> (w44:refnum<vi>)
      n23 = control-ref of="Position.Axis 122::98"() -> (w45:refnum<vi>)
      n24 = control-ref of="Position.Axis 123::98"() -> (w46:refnum<vi>)
      n25 = control-ref of="Position.Axis 131::98"() -> (w47:refnum<vi>)
      n26 = control-ref of="Position.Axis 132::98"() -> (w48:refnum<vi>)
      n27 = control-ref of="Position.Axis 133::98"() -> (w49:refnum<vi>)
      n28 = control-ref of="Position.Axis 141::98"() -> (w50:refnum<vi>)
      n29 = control-ref of="Position.Axis 142::98"() -> (w51:refnum<vi>)
      n30 = control-ref of="Position.Axis 143::98"() -> (w52:refnum<vi>)
      n31 = control-ref of="Position.Axis 211::98"() -> (w53:refnum<vi>)
      n32 = control-ref of="Position.Axis 212::98"() -> (w54:refnum<vi>)
      n33 = control-ref of="Position.Axis 213::98"() -> (w55:refnum<vi>)
      n34 = control-ref of="Position.Axis 221::98"() -> (w56:refnum<vi>)
      n35 = control-ref of="Position.Axis 222::98"() -> (w57:refnum<vi>)
      n36 = control-ref of="Position.Axis 223::98"() -> (w58:refnum<vi>)
      n37 = control-ref of="Position.Axis 231::98"() -> (w59:refnum<vi>)
      n38 = control-ref of="Position.Axis 232::98"() -> (w60:refnum<vi>)
      n39 = control-ref of="Position.Axis 233::98"() -> (w61:refnum<vi>)
      n40 = control-ref of="Position.Axis 241::98"() -> (w62:refnum<vi>)
      n41 = control-ref of="Position.Axis 242::98"() -> (w63:refnum<vi>)
      n42 = control-ref of="Position.Axis 243::98"() -> (w64:refnum<vi>)
      n43 = control-ref of="Position.Axis 311::98"() -> (w65:refnum<vi>)
      n44 = control-ref of="Position.Axis 312::98"() -> (w66:refnum<vi>)
      n45 = control-ref of="Position.Axis 313::98"() -> (w67:refnum<vi>)
      n46 = control-ref of="Position.Axis 321::98"() -> (w68:refnum<vi>)
      n47 = control-ref of="Position.Axis 322::98"() -> (w69:refnum<vi>)
      n48 = control-ref of="Position.Axis 323::98"() -> (w70:refnum<vi>)
      n49 = control-ref of="Position.Axis 331::98"() -> (w71:refnum<vi>)
      n50 = control-ref of="Position.Axis 332::98"() -> (w72:refnum<vi>)
      n51 = control-ref of="Position.Axis 333::98"() -> (w73:refnum<vi>)
      n52 = control-ref of="Position.Axis 341::98"() -> (w74:refnum<vi>)
      n53 = control-ref of="Position.Axis 342::98"() -> (w75:refnum<vi>)
      n54 = control-ref of="Position.Axis 343::98"() -> (w76:refnum<vi>)
      n55 = control-ref of="Position.Axis 411::98"() -> (w77:refnum<vi>)
      n56 = control-ref of="Position.Axis 412::98"() -> (w78:refnum<vi>)
      n57 = control-ref of="Position.Axis 413::98"() -> (w79:refnum<vi>)
      n58 = control-ref of="Position.Axis 421::98"() -> (w80:refnum<vi>)
      n59 = control-ref of="Position.Axis 422::98"() -> (w81:refnum<vi>)
      n60 = control-ref of="Position.Axis 423::98"() -> (w82:refnum<vi>)
      n61 = control-ref of="Position.Axis 431::98"() -> (w83:refnum<vi>)
      n62 = control-ref of="Position.Axis 432::98"() -> (w84:refnum<vi>)
      n63 = control-ref of="Position.Axis 433::98"() -> (w85:refnum<vi>)
      n64 = control-ref of="Position.Axis 441::98"() -> (w86:refnum<vi>)
      n65 = control-ref of="Position.Axis 442::98"() -> (w87:refnum<vi>)
      n66 = control-ref of="Position.Axis 443::98"() -> (w88:refnum<vi>)
      n67 = control-ref of="Position.Axis 511::98"() -> (w89:refnum<vi>)
      n68 = control-ref of="Position.Axis 512::98"() -> (w90:refnum<vi>)
      n69 = control-ref of="Position.Axis 513::98"() -> (w91:refnum<vi>)
      n70 = control-ref of="Position.Axis 521::98"() -> (w92:refnum<vi>)
      n71 = control-ref of="Position.Axis 522::98"() -> (w93:refnum<vi>)
      n72 = control-ref of="Position.Axis 523::98"() -> (w94:refnum<vi>)
      n73 = control-ref of="Position.Axis 531::98"() -> (w95:refnum<vi>)
      n74 = control-ref of="Position.Axis 532::98"() -> (w96:refnum<vi>)
      n75 = control-ref of="Position.Axis 533::98"() -> (w97:refnum<vi>)
      n76 = control-ref of="Position.Axis 541::98"() -> (w98:refnum<vi>)
      n77 = control-ref of="Position.Axis 542::98"() -> (w99:refnum<vi>)
      n78 = control-ref of="Position.Axis 543::98"() -> (w100:refnum<vi>)
      n79 = control-ref of="Position.Axis 111::99"() -> (w232:refnum<vi>)
      n80 = control-ref of="Position.Axis 112::99"() -> (w231:refnum<vi>)
      n81 = control-ref of="Position.Axis 113::99"() -> (w230:refnum<vi>)
      n82 = control-ref of="Position.Axis 121::99"() -> (w229:refnum<vi>)
      n83 = control-ref of="Position.Axis 122::99"() -> (w228:refnum<vi>)
      n84 = control-ref of="Position.Axis 123::99"() -> (w227:refnum<vi>)
      n85 = control-ref of="Position.Axis 131::99"() -> (w226:refnum<vi>)
      n86 = control-ref of="Position.Axis 132::99"() -> (w225:refnum<vi>)
      n87 = control-ref of="Position.Axis 133::99"() -> (w224:refnum<vi>)
      n88 = control-ref of="Position.Axis 141::99"() -> (w223:refnum<vi>)
      n89 = control-ref of="Position.Axis 142::99"() -> (w222:refnum<vi>)
      n90 = control-ref of="Position.Axis 143::99"() -> (w221:refnum<vi>)
      n91 = control-ref of="Position.Axis 211::99"() -> (w220:refnum<vi>)
      n92 = control-ref of="Position.Axis 212::99"() -> (w219:refnum<vi>)
      n93 = control-ref of="Position.Axis 213::99"() -> (w218:refnum<vi>)
      n94 = control-ref of="Position.Axis 221::99"() -> (w217:refnum<vi>)
      n95 = control-ref of="Position.Axis 222::99"() -> (w216:refnum<vi>)
      n96 = control-ref of="Position.Axis 223::99"() -> (w215:refnum<vi>)
      n97 = control-ref of="Position.Axis 231::99"() -> (w214:refnum<vi>)
      n98 = control-ref of="Position.Axis 232::99"() -> (w213:refnum<vi>)
      n99 = control-ref of="Position.Axis 233::99"() -> (w212:refnum<vi>)
      n100 = control-ref of="Position.Axis 241::99"() -> (w211:refnum<vi>)
      n101 = control-ref of="Position.Axis 242::99"() -> (w210:refnum<vi>)
      n102 = control-ref of="Position.Axis 243::99"() -> (w209:refnum<vi>)
      n103 = control-ref of="Position.Axis 311::99"() -> (w208:refnum<vi>)
      n104 = control-ref of="Position.Axis 312::99"() -> (w207:refnum<vi>)
      n105 = control-ref of="Position.Axis 313::99"() -> (w206:refnum<vi>)
      n106 = control-ref of="Position.Axis 321::99"() -> (w205:refnum<vi>)
      n107 = control-ref of="Position.Axis 322::99"() -> (w204:refnum<vi>)
      n108 = control-ref of="Position.Axis 323::99"() -> (w203:refnum<vi>)
      n109 = control-ref of="Position.Axis 331::99"() -> (w202:refnum<vi>)
      n110 = control-ref of="Position.Axis 332::99"() -> (w201:refnum<vi>)
      n111 = control-ref of="Position.Axis 333::99"() -> (w200:refnum<vi>)
      n112 = control-ref of="Position.Axis 341::99"() -> (w199:refnum<vi>)
      n113 = control-ref of="Position.Axis 342::99"() -> (w198:refnum<vi>)
      n114 = control-ref of="Position.Axis 343::99"() -> (w197:refnum<vi>)
      n115 = control-ref of="Position.Axis 411::99"() -> (w196:refnum<vi>)
      n116 = control-ref of="Position.Axis 412::99"() -> (w195:refnum<vi>)
      n117 = control-ref of="Position.Axis 413::99"() -> (w194:refnum<vi>)
      n118 = control-ref of="Position.Axis 421::99"() -> (w193:refnum<vi>)
      n119 = control-ref of="Position.Axis 422::99"() -> (w192:refnum<vi>)
      n120 = control-ref of="Position.Axis 423::99"() -> (w191:refnum<vi>)
      n121 = control-ref of="Position.Axis 431::99"() -> (w190:refnum<vi>)
      n122 = control-ref of="Position.Axis 432::99"() -> (w189:refnum<vi>)
      n123 = control-ref of="Position.Axis 433::99"() -> (w188:refnum<vi>)
      n124 = control-ref of="Position.Axis 441::99"() -> (w187:refnum<vi>)
      n125 = control-ref of="Position.Axis 442::99"() -> (w186:refnum<vi>)
      n126 = control-ref of="Position.Axis 443::99"() -> (w185:refnum<vi>)
      n127 = control-ref of="Position.Axis 511::99"() -> (w184:refnum<vi>)
      n128 = control-ref of="Position.Axis 512::99"() -> (w183:refnum<vi>)
      n129 = control-ref of="Position.Axis 513::99"() -> (w182:refnum<vi>)
      n130 = control-ref of="Position.Axis 521::99"() -> (w181:refnum<vi>)
      n131 = control-ref of="Position.Axis 522::99"() -> (w180:refnum<vi>)
      n132 = control-ref of="Position.Axis 523::99"() -> (w179:refnum<vi>)
      n133 = control-ref of="Position.Axis 531::99"() -> (w178:refnum<vi>)
      n134 = control-ref of="Position.Axis 532::99"() -> (w177:refnum<vi>)
      n135 = control-ref of="Position.Axis 533::99"() -> (w176:refnum<vi>)
      n136 = control-ref of="Position.Axis 541::99"() -> (w175:refnum<vi>)
      n137 = control-ref of="Position.Axis 542::99"() -> (w174:refnum<vi>)
      n138 = control-ref of="Position.Axis 543::99"() -> (w173:refnum<vi>)
      n139 = Build Array(w41, w42, w43, w44, w45, w46, w47, w48, w49, w50, w51, w52, w53, w54, w55, w56, w57, w58, w59, w60, w61, w62, w63, w64, w65, w66, w67, w68, w69, w70, w71, w72, w73, w74, w75, w76, w77, w78, w79, w80, w81, w82, w83, w84, w85, w86, w87, w88, w89, w90, w91, w92, w93, w94, w95, w96, w97, w98, w99, w100) -> (w38:refnum<vi>[])
      n140 = Build Array(w232, w231, w230, w229, w228, w227, w226, w225, w224, w223, w222, w221, w220, w219, w218, w217, w216, w215, w214, w213, w212, w211, w210, w209, w208, w207, w206, w205, w204, w203, w202, w201, w200, w199, w198, w197, w196, w195, w194, w193, w192, w191, w190, w189, w188, w187, w186, w185, w184, w183, w182, w181, w180, w179, w178, w177, w176, w175, w174, w173) -> (w37:refnum<vi>[])
      n141 = Build Array (concatenate)(w37, w38) -> (→"motor refs":refnum<vi>[])
      n142 = call "getMotorNames.vi"("DeviceName"="GUIdevice 99") -> ("elements"=w35:string[])  [unwired: 10 in]
      n143 = call "getMotorNames.vi"("DeviceName"="GUIdevice 98") -> ("elements"=w34:string[])  [unwired: 10 in]
      n144 = Build Array (concatenate)(w35, w34) -> (w39:string[])
      "Names" <- w39
      n145 = property on="Motor CCD 1" class="Ring (strict)"("Strings []"=w39) -> ()  [unwired: 2 in, 2 out]
      n146 = property on="Motor CCD 2" class="Ring (strict)"("Strings []"=w39) -> ()  [unwired: 2 in, 2 out]
      n147 = property on="Motor CCD 3" class="Ring (strict)"("Strings []"=w39) -> ()  [unwired: 2 in, 2 out]
      n148 = property on="Motor CCD 4" class="Ring (strict)"("Strings []"=w39) -> ()  [unwired: 2 in, 2 out]
      n149 = property on="Motor CCD 5" class="Ring (strict)"("Strings []"=w39) -> ()  [unwired: 2 in, 2 out]
      n150 = property on="Motor CCD 6" class="Ring (strict)"("Strings []"=w39) -> ()  [unwired: 2 in, 2 out]
      n151 = property on="Motor CCD 7" class="Ring (strict)"("Strings []"=w39) -> ()  [unwired: 2 in, 2 out]
      n152 = property on="Motor CCD 8" class="Ring (strict)"("Strings []"=w39) -> ()  [unwired: 2 in, 2 out]
      n153 = property on="Motor CCD 9" class="Ring (strict)"("Strings []"=w39) -> ()  [unwired: 2 in, 2 out]
      n154 = property on="Motor CCD 10" class="Ring (strict)"("Strings []"=w39) -> ()  [unwired: 2 in, 2 out]
      n155 = property on="Motor CCD 11" class="Ring (strict)"("Strings []"=w39) -> ()  [unwired: 2 in, 2 out]
      n156 = property on="Motor CCD 12" class="Ring (strict)"("Strings []"=w39) -> ()  [unwired: 2 in, 2 out]
      n157 = property on="ActiveMotor" class="Ring (strict)"("Strings []"=w35) -> ()  [unwired: 2 in, 2 out]
      n158 = control-ref of="Target.X::1"() -> (w159:refnum<vi>)
      n159 = control-ref of="Target.Y::1"() -> (w158:refnum<vi>)
      n160 = control-ref of="Target.X::2"() -> (w157:refnum<vi>)
      n161 = control-ref of="Target.Y::2"() -> (w156:refnum<vi>)
      n162 = control-ref of="Target.X::3"() -> (w155:refnum<vi>)
      n163 = control-ref of="Target.Y::3"() -> (w154:refnum<vi>)
      n164 = control-ref of="Target.X::4"() -> (w153:refnum<vi>)
      n165 = control-ref of="Target.Y::4"() -> (w152:refnum<vi>)
      n166 = control-ref of="Target.X::5"() -> (w151:refnum<vi>)
      n167 = control-ref of="Target.Y::5"() -> (w150:refnum<vi>)
      n168 = control-ref of="Target.X::6"() -> (w149:refnum<vi>)
      n169 = control-ref of="Target.Y::6"() -> (w148:refnum<vi>)
      n170 = control-ref of="Target.X::7"() -> (w147:refnum<vi>)
      n171 = control-ref of="Target.Y::7"() -> (w146:refnum<vi>)
      n172 = control-ref of="Target.X::8"() -> (w145:refnum<vi>)
      n173 = control-ref of="Target.Y::8"() -> (w144:refnum<vi>)
      n174 = control-ref of="Target.X::9"() -> (w121:refnum<vi>)
      n175 = control-ref of="Target.Y::9"() -> (w120:refnum<vi>)
      n176 = control-ref of="Target.X::10"() -> (w119:refnum<vi>)
      n177 = control-ref of="Target.Y::10"() -> (w118:refnum<vi>)
      n178 = control-ref of="Target.X::11"() -> (w117:refnum<vi>)
      n179 = control-ref of="Target.Y::11"() -> (w116:refnum<vi>)
      n180 = control-ref of="Target.X::12"() -> (w115:refnum<vi>)
      n181 = control-ref of="Target.Y::12"() -> (w114:refnum<vi>)
      n182 = call "IMAQ Create"("Image Name"="GUIdevice 8", "Image Type"=w104) -> ("New Image"=→"image::8":T9)  [unwired: 3 in, 1 out]
      n183 = call "IMAQ Create"("Image Name"="GUIdevice 9", "Image Type"=w104) -> ("New Image"=→"image::9":T9)  [unwired: 3 in, 1 out]
      n184 = call "IMAQ Create"("Image Name"="GUIdevice 10", "Image Type"=w104) -> ("New Image"=→"image::10":T9)  [unwired: 3 in, 1 out]
      n185 = call "IMAQ Create"("Image Name"="GUIdevice 6", "Image Type"=w104) -> ("New Image"=→"image::6":T9)  [unwired: 3 in, 1 out]
      n186 = call "IMAQ Create"("Image Name"="GUIdevice 7", "Image Type"=w104) -> ("New Image"=→"image::7":T9)  [unwired: 3 in, 1 out]
      n187 = call "IMAQ Create"("Image Name"="GUIdevice 11", "Image Type"=w104) -> ("New Image"=→"image::11":T9)  [unwired: 3 in, 1 out]
      n188 = call "IMAQ Create"("Image Name"="GUIdevice 12", "Image Type"=w104) -> ("New Image"=→"image::12":T9)  [unwired: 3 in, 1 out]
      n189 = call "IMAQ Create"("Image Name"="GUIdevice 2") -> ("New Image"=→"image::2":T9)  [unwired: 4 in, 1 out]
      n190 = call "IMAQ Create"("Image Name"="GUIdevice 4", "Image Type"=w104) -> ("New Image"=→"image::4":T9)  [unwired: 3 in, 1 out]
      n191 = call "IMAQ Create"("Image Name"="GUIdevice 1", "Image Type"=w104) -> ("New Image"=→"image::1":T9)  [unwired: 3 in, 1 out]
      n192 = call "IMAQ Create"("Image Name"="GUIdevice 3", "Image Type"=w104) -> ("New Image"=→"image::3":T9)  [unwired: 3 in, 1 out]
      n193 = call "IMAQ Create"("Image Name"="GUIdevice 5", "Image Type"=w104) -> ("New Image"=→"image::5":T9)  [unwired: 3 in, 1 out]
      n194 = Build Array("GUIdevice 1", "GUIdevice 2", "GUIdevice 3", "GUIdevice 4", "GUIdevice 5", "GUIdevice 6", "GUIdevice 7", "GUIdevice 8", "GUIdevice 9", "GUIdevice 10", "GUIdevice 11", "GUIdevice 12") -> (w133:string[])
      "CCDs" <- w133
      n195 = property on="image::8" class="ImageControl"("Caption.Text"="GUIdevice 8") -> ()  [unwired: 2 in, 2 out]
      n196 = property on="image::10" class="ImageControl"("Caption.Text"="GUIdevice 10") -> ()  [unwired: 2 in, 2 out]
      n197 = property on="image::9" class="ImageControl"("Caption.Text"="GUIdevice 9") -> ()  [unwired: 2 in, 2 out]
      n198 = property on="image::1" class="ImageControl"("Caption.Text"="GUIdevice 1") -> ()  [unwired: 2 in, 2 out]
      n199 = property on="image::2" class="ImageControl"("Caption.Text"="GUIdevice 2") -> ()  [unwired: 2 in, 2 out]
      n200 = property on="image::3" class="ImageControl"("Caption.Text"="GUIdevice 3") -> ()  [unwired: 2 in, 2 out]
      n201 = property on="image::4" class="ImageControl"("Caption.Text"="GUIdevice 4") -> ()  [unwired: 2 in, 2 out]
      n202 = property on="image::5" class="ImageControl"("Caption.Text"="GUIdevice 5") -> ()  [unwired: 2 in, 2 out]
      n203 = property on="image::6" class="ImageControl"("Caption.Text"="GUIdevice 6") -> ()  [unwired: 2 in, 2 out]
      n204 = property on="image::7" class="ImageControl"("Caption.Text"="GUIdevice 7") -> ()  [unwired: 2 in, 2 out]
      n205 = property on="image::11" class="ImageControl"("Caption.Text"="GUIdevice 11") -> ()  [unwired: 2 in, 2 out]
      n206 = property on="image::12" class="ImageControl"("Caption.Text"="GUIdevice 12") -> ()  [unwired: 2 in, 2 out]
      n207 = Array To Cluster(array=w133) -> (cluster=→"Cameras":T21)
      n208 = Bundle("Target.X::1"=w159, "Target.Y::1"=w158) -> (w143:T22)  [unwired: 1 in]
      n209 = Bundle("Target.X::2"=w157, "Target.Y::2"=w156) -> (w142:T23)  [unwired: 1 in]
      n210 = Bundle("Target.X::3"=w155, "Target.Y::3"=w154) -> (w141:T24)  [unwired: 1 in]
      n211 = Bundle("Target.X::4"=w153, "Target.Y::4"=w152) -> (w134:T25)  [unwired: 1 in]
      n212 = Bundle("Target.X::5"=w151, "Target.Y::5"=w150) -> (w140:T26)  [unwired: 1 in]
      n213 = Bundle("Target.X::6"=w149, "Target.Y::6"=w148) -> (w139:T27)  [unwired: 1 in]
      n214 = Bundle("Target.X::7"=w147, "Target.Y::7"=w146) -> (w138:T28)  [unwired: 1 in]
      n215 = Bundle("Target.X::8"=w145, "Target.Y::8"=w144) -> (w137:T29)  [unwired: 1 in]
      n216 = Bundle("Target.X::12"=w115, "Target.Y::12"=w114) -> (w110:T30)  [unwired: 1 in]
      n217 = Bundle("Target.X::9"=w121, "Target.Y::9"=w120) -> (w113:T31)  [unwired: 1 in]
      n218 = Bundle("Target.X::10"=w119, "Target.Y::10"=w118) -> (w112:T32)  [unwired: 1 in]
      n219 = Bundle("Target.X::11"=w117, "Target.Y::11"=w116) -> (w111:T33)  [unwired: 1 in]
      n220 = property on="CCDs" class="Ring (strict)"("Strings []"=w133) -> ()  [unwired: 2 in, 2 out]
      n221 = Build Array(w143, w142, w141, w134, w140, w139, w138, w137, w113, w112, w111, w110) -> (w136:T34)
      n222 = Tick Count (ms)() -> (millisecond timer value=→"millisecond timer value":u32)
      n223 = property on="Feedback Global" class="Bool (strict)"("Value"=FALSE ("Feedback Global")) -> ()  [unwired: 2 in, 2 out]
      n224 = Get Date/Time In Seconds() -> (seconds since 1Jan1904=w123:timestamp)
      n225 = Format Date/Time String(time format string (%c)="%Y%m%d%H%M", seconds (now)=w123) -> (date/time string=w122:string)  [unwired: 1 in]
      n226 = Concatenate Strings(w122, "Beampointing_Pico.tdms" ("string")) -> (w126:string)
      n227 = String To Path(string=w126) -> (path=w125:path)
      n228 = Build Path(base path=w32, name or relative path=w125) -> (appended path=w128:path)
      n229 = call <vilib>:"Add State(s) to Queue__jki_lib_state_machine.vi"("State(s) in (\"\")"="Macro: Initialize") -> ("States Out"=w234:string)  [unwired: 14 in]
      n230 = Create User Event(user event datatype=T14 {"EventEnum"=enum."new data", "Device name"="Device name"} ("New Event")) -> (user event=w242:refnum<user-event>, error out=w244:errorcluster)  [unwired: 1 in]
      "tcp data event" <- w242
      n231 = while "JKI - String-Based Queued State Machine (Basic) v1.0" {
        shift-right: [w272] -> w132
        shift-left: _ -> [w260]
        shift-right: [w275] -> w160
        shift-left: _ -> [w271]
        shift-right: [w274] -> _
        shift-left: w234 -> [w276]
        tunnel: w136 -> [w269]
        tunnel: w133 -> [w267]
        tunnel: [w267] -> w161
        tunnel: w136 -> [w268]
        tunnel: w128 -> [w258]
        tunnel: w32 -> [w257]
        stop <- w273 stop-if-true
        n232 = Unbundle By Name(w260) -> ("active cams"=w259:string[])
        n233 = call <vilib>:"Parse State Queue__jki_lib_state_machine.vi"("State Queue"=w276, "Error In (no error)"=w271) -> ("Remaining States"=w278:string, "Current State"=w279:string, "Arguments"=w277:string)  [unwired: 11 in]
        "Current State" <- w279
        n234 = case shown="\"\", \"Idle\"" w279 {
          selector: w279 -> [_ _ w575 _ _ _ _ _ _ _ _ _ _ _ _ _ _ _ _ _ _ _ _ _ _ _ _ _ _ _ _ _ _ _ _ _ _ _ _ _]
          tunnel: w278 -> [w311 w574 w579 w597 w604 w609 w613 w650 w668 w672 w676 w682 w693 w717 w727 w737 w741 w763 w865 w918 w931 w940 w967 w988 w992 w1011 w1150 w1304 w1395 w1461 w1499 w1519 w1534 w1623 w1675 w1685 w1692 w1725 w1751 w1778]
          tunnel: w277 -> [_ _ _ _ _ _ _ _ _ _ _ w677 w688 _ _ _ _ w758 w816 _ w928 _ _ _ _ w1013 _ w1282 w1372 _ _ _ _ _ _ _ w1689 _ _ _]
          tunnel: w260 -> [w309 w571 w577 w587 w601 w607 w610 _ w664 w669 w674 w680 w687 w714 w725 w729 w738 w755 w817 w916 w923 w936 w959 w981 w989 w995 w1144 w1297 w1388 w1458 w1470 w1516 w1531 w1597 w1672 w1682 w1688 w1713 w1748 w1769]
          tunnel: [w308 w572 w581 w595 errorcluster {"status"=FALSE, "code"=0, "source"=""} ("error out") w606 w611 w622 w661 w670 w673 w678 w690 w715 w726 w735 w739 w759 w821 w908 w929 w938 w965 w986 w990 w1015 w1174 w1302 w1393 w1459 w1497 w1517 w1532 w1582 w1673 w1683 w1690 w1695 w1749 w1776] -> w275
          tunnel: w271 -> [w307 w572 w580 w595 w600 w606 w611 w628 w666 w670 w673 w679 w691 w715 w726 w735 w739 w759 w819 w899 w929 w938 w965 w986 w990 w1015 w1174 w1302 w1393 w1459 w1497 w1517 w1532 w1618 w1673 w1683 w1690 w1711 w1749 w1776]
          tunnel: [w310 w573 w578 w596 w603 w608 w612 w649 w667 w671 w675 w681 w692 w716 w718 w736 w740 w749 w864 w917 w930 w939 w966 w987 w991 w1018 w1175 w1303 w1394 w1460 w1498 w1518 w1533 w1585 w1674 w1684 w1691 w1724 w1750 w1777] -> w274
          tunnel: [_ _ _ _ _ TRUE _ _ _ _ _ _ _ _ _ _ _ _ _ _ _ _ _ _ _ _ _ _ _ _ _ _ _ _ _ _ _ _ _ _] -> w273
          tunnel: [w304 w571 w577 w586 w601 w607 w610 w616 w664 w669 w674 w680 w687 w714 w725 w729 w738 w760 w854 w916 w922 w935 w958 w980 w989 w1040 w1143 w1297 w1388 w1457 w1470 w1516 w1531 w1597 w1671 w1682 w1687 w1714 w1748 w1768] -> w272
          tunnel: "update speed [ms]" -> [w306 _ _ _ _ _ _ _ _ _ _ _ _ _ _ _ _ _ _ _ _ _ _ _ _ _ _ _ _ _ _ _ _ _ _ _ _ _ _ _]
          tunnel: w269 -> [w303 _ _ _ _ _ _ _ _ _ _ _ _ _ _ _ _ _ _ _ _ _ _ _ _ w1038 _ _ _ _ _ _ _ _ _ _ _ _ w1732 _]
          tunnel: w267 -> [w305 _ _ _ _ _ _ w621 _ _ _ _ _ _ _ _ _ w762 w818 _ w924 _ _ _ _ w1003 w1140 w1301 w1392 _ w1471 _ w1520 w1621 _ _ _ _ _ _]
          tunnel: w258 -> [_ _ _ _ _ _ _ w626 _ _ _ _ _ _ _ _ _ _ _ _ _ _ _ _ _ _ _ _ _ _ _ _ _ _ _ _ _ _ _ _]
          tunnel: w257 -> [_ _ _ _ _ _ _ _ _ _ _ _ _ _ _ _ _ _ _ _ _ _ _ _ _ _ _ _ _ _ _ _ _ _ _ _ _ w1704 _ _]
          frame "", "Idle" {
            # "executes when the state queue is empty"
            n235 = event shown="[9] \"ActiveMotor 2\": Value Change" {
              selector: _ -> [_ _ _ _ _ _ _ _ _ _ _ _ _ _ _ _ _ _ _]
              dyn-events: _ -> [_ _ _ _ _ _ _ _ _ _ _ _ _ _ _ _ _ _ _]
              timeout: w306 -> [_ _ _ _ _ _ _ _ _ _ _ _ _ _ _ _ _ _ _]
              tunnel: w311 -> [w314 w441 w456 w475 w480 w485 w490 w496 w503 w506 w514 w525 w530 w539 w544 w550 w556 w564 w570]
              tunnel: [w329 w440 w455 w474 w479 w484 w489 w495 w502 w506 w513 w524 w529 w538 w543 w549 w555 w563 w569] -> w310
              tunnel: w309 -> [w319 w438 w452 w471 w477 w482 w487 w493 w500 w507 w511 w523 w527 w532 w541 w547 w553 w561 w567]
              tunnel: [w323 w439 w454 w473 w478 w483 w488 w494 w501 w505 w512 w515 w528 w537 w542 w548 w554 w562 w568] -> w308
              tunnel: w307 -> [w326 w439 w454 w473 w478 w483 w488 w494 w501 w505 w512 w516 w528 w537 w542 w548 w554 w562 w568]
              tunnel: [w328 w438 w452 w470 w477 w482 w487 w493 w500 w507 w511 w523 w527 w532 w541 w547 w553 w561 w567] -> w304
              tunnel: w305 -> [w346 _ w448 _ _ _ _ _ _ _ _ _ _ _ _ _ _ _ _]
              tunnel: w303 -> [_ _ w450 _ _ _ _ _ _ _ _ _ _ _ _ _ _ _ _]
              event Timeout {
                n236 = event-data() -> ()  [unwired: 1 in, 1 out]
                n237 = Unbundle By Name(w319) -> ("Centroid X"=w316:dbl[][], "Centroid Y"=w356:dbl[][], "Size"=w349:dbl[][], "detection para"=w345:T3[], "active cams"=w340:string[], "thresholds"=w337:cluster{"Lower value":sgl, "Upper value":sgl}[])
                n238 = Unbundle By Name(w319) -> ("active ccd"=w318:i32)
                n239 = call <userlib>:"Tick Count (ms)__ogtk.vi"("error in (no error)"=w326) -> ("error out"=w325:errorcluster, "millisecond timer value"=→"millisecond timer 2":u32)  [unwired: 9 in]
                n240 = for {
                  N: 12 ("Numeric 2") -> [_]
                  tunnel: w340 -> [w401] mode=indexing
                  tunnel: [w402] -> w354 mode=indexing
                  tunnel: w346 -> [w425]
                  tunnel: w345 -> [w423]
                  tunnel: [w421] -> w322 mode=indexing
                  tunnel: [w420] -> w320 mode=indexing
                  tunnel: [w418] -> w341 mode=indexing
                  tunnel: "autodetect" -> [w412]
                  tunnel: w325 -> [w426]
                  tunnel: [w427] -> w347
                  shift-right: [w409] -> w317
                  shift-left: w337 -> [w411]
                  shift-right: [w396] -> w355
                  shift-left: w316 -> [w398]
                  shift-right: [w392] -> w357
                  shift-left: w356 -> [w394]
                  shift-right: [w386] -> w348
                  shift-left: w349 -> [w388]
                  w390 = 0 ("index")
                  n241 = call-poly <userlib>:"Filter 1D Array__ogtk.vi"("items to filter"=w401, "array"=w425) -> ("filtered item indices"=w424:i32[])  [unwired: 4 in, 1 out]
                  n242 = Index Array(array=w424) -> (element=w387:i32)  [unwired: 1 in]
                  n243 = Index Array(array=w388, index (row)=w387) -> (element=w416:dbl[])  [unwired: 1 in]
                  n244 = Index Array(array=w394, index (row)=w387) -> (element=w417:dbl[])  [unwired: 1 in]
                  n245 = Index Array(array=w411, index=w387) -> (element=w415:cluster{"Lower value":sgl, "Upper value":sgl})
                  n246 = Index Array(array=w398, index (row)=w387) -> (element=w400:dbl[])  [unwired: 1 in]
                  n247 = Index Array(array=w423, index=w387) -> (element=w419:T3)
                  n248 = call "CENTRIOD DETECTION.vi"("Refnum in"=w401, "auto threshold"=w412, "Threshold Range In"=w415, "beam detection para"=w419, "error in (no error)"=w426) -> ("Bounding Rect"=w418:T35, "Particle Reports (Pixels)"=w420:T1, "Threshold Range Out"=w410:cluster{"Lower value":sgl, "Upper value":sgl}, "Centriod"=w428:cluster{"X":dbl, "Y":dbl}, "error out"=w427:errorcluster)  [unwired: 7 in, 3 out]
                  n249 = Unbundle By Name(w428) -> ("X"=w399:dbl, "Y"=w395:dbl)
                  n250 = Empty Array?(array=w420) -> (empty?=w422:bool)
                  n251 = Not(x=w422) -> (.not. x?=w421:bool)
                  n252 = Replace Array Subset(array=w411, new element=w410, index=w387) -> (w409:cluster{"Lower value":sgl, "Upper value":sgl}[])
                  n253 = Unbundle By Name(w418) -> ("Right"=w408:dbl, "Left"=w407:dbl, "Bottom"=w406:dbl, "Top"=w405:dbl)
                  n254 = Subtract(x=w408, y=w407) -> (x-y=w403:dbl)
                  n255 = Subtract(x=w406, y=w405) -> (x-y=w404:dbl)
                  n256 = Multiply(x=w403, y=w404) -> (x*y=w391:dbl)
                  n257 = Insert Into Array(array=w417, index=w390, new element=w395) -> (w393:dbl[])
                  n258 = Insert Into Array(array=w416, index=w390, new element=w391) -> (w389:dbl[])
                  n259 = Insert Into Array(array=w400, index=w390, new element=w399) -> (w397:dbl[])
                  n260 = for {
                    shift-right: [w429] -> w413
                    shift-left: dbl[] [] ("Array 4") -> [w432]
                    tunnel: w393 -> [w430] mode=indexing
                    n261 = Equal To 0?(x=w430) -> (x = 0?=w431:bool)
                    n262 = case shown="False" w431 {
                      tunnel: w432 -> [w435 w436]
                      tunnel: w430 -> [w434 _]
                      tunnel: [w433 w436] -> w429
                      frame False {
                        n263 = Build Array (concatenate)(w435, w434) -> (w433:dbl[])
                      }
                      frame True {
                      }
                    }
                  }
                  n264 = Replace Array Subset(array=w398, new element=w397, index (row)=w387) -> (w396:dbl[][])  [unwired: 1 in]
                  n265 = Replace Array Subset(array=w394, new element=w393, index (row)=w387) -> (w392:dbl[][])  [unwired: 1 in]
                  n266 = Replace Array Subset(array=w388, new element=w389, index (row)=w387) -> (w386:dbl[][])  [unwired: 1 in]
                  n267 = Array Size(array=w413) -> (size(s)=w402:i32)
                }
                "detected" <- w322
                "Particle Reports (Pixels)" <- w320
                "Box" <- w341
                n268 = Bundle(0, 1, "Centroid X"=w316) -> (→"Status":cluster{i32, i32, "Centroid X":dbl[][]})  [unwired: 1 in]
                n269 = Index Array(array=w320, index (row)=w318) -> (element=→"particles":T1)  [unwired: 1 in]
                n270 = call <vilib>:"Clear Errors.vi"("error in (no error)"=w347) -> ("error out"=w323:errorcluster)  [unwired: 6 in]
                n271 = local read "Img to avg"() -> (w331:i32)
                n272 = local read "Numeric"() -> (w334:dbl)
                n273 = Increment(x=w331) -> (x+1=w330:i32)
                n274 = Greater Or Equal?(x=w334, y=w330) -> (x >= y?=w327:bool)
                n275 = Increment(x=w334) -> (x+1=w333:dbl)
                n276 = Select(t=0.0, s=w327, f=w333) -> (s? t:f=w332:dbl)
                n277 = local write "Numeric"(w332) -> ()
                n278 = for {
                  tunnel: w354 -> [w378] mode=indexing
                  tunnel: w340 -> [w385] mode=indexing
                  shift-right: [w380] -> w350
                  shift-left: "" ("GUIdevice 7") -> [w383]
                  tunnel: [w373] -> w352 mode=indexing
                  tunnel: "Detection Rate" -> [w377]
                  tunnel: w332 -> [w375]
                  n279 = local read "Img to avg"() -> (w379:i32)
                  n280 = Greater Or Equal?(x=w378, y=w379) -> (x >= y?=w374:bool)
                  n281 = Multiply(x=w377, y=w375) -> (x*y=w376:dbl)
                  n282 = Greater Or Equal?(x=w378, y=w376) -> (x >= y?=w372:bool)
                  n283 = And(x=w374, y=w372) -> (x .and. y?=w373:bool)
                  n284 = Select(t=w385, s=w373, f="") -> (s? t:f=w381:string)
                  n285 = Concatenate Strings(w383, "\t", w381) -> (w380:string)
                }
                n286 = Bundle By Name(cluster=w319, "thresholds"=w317, "detected"=w322) -> (w338:T36)
                n287 = Bundle By Name(cluster=w338, "Centroid X"=w355, "Centroid Y"=w357, "Size"=w348) -> (w313:T36)
                n288 = Unbundle By Name(w313) -> ("img to avg"=w312:i32)
                n289 = Or Array Elements(Boolean array=w352) -> (logical OR=w351:bool)
                n290 = case shown="True" w327 {
                  tunnel: w313 -> [w358 w365]
                  tunnel: [w358 w364] -> w328
                  tunnel: w312 -> [_ w360]
                  frame False {
                  }
                  frame True {
                    n291 = Decrement(x=w360) -> (x-1=w359:i32)
                    n292 = Initialize Array(0.0 ("element"), 12 ("dimension size"), w359) -> (w361:dbl[][])
                    n293 = Bundle By Name(cluster=w365, "Centroid X"=w361, "Centroid Y"=w361, "Size"=w361) -> (w364:T36)
                  }
                }
                n294 = case shown="True" w351 {
                  tunnel: w350 -> [_ w370]
                  tunnel: w314 -> [w366 w368]
                  tunnel: [w366 w367] -> w329
                  frame False {
                  }
                  frame True {
                    n295 = call <vilib>:"Build State String with Arguments__jki_lib_state_machine.vi"("Arguments (\"\")"=w370, "State"="detected") -> ("State with Arguments"=w369:string)  [unwired: 4 in]
                    n296 = call <vilib>:"Add State(s) to Queue__jki_lib_state_machine.vi"("State(s) in (\"\")"=w368, "State(s) at Back (\"\")"=w369) -> ("States Out"=w367:string)  [unwired: 13 in]
                  }
                }
              }
              event "stop": Value Change {
                # "Exit Button Value Change (pressed) Event\n(this executes Macro: Exit to terminate the VI)"
                n297 = event-data() -> ()  [unwired: 1 in, 6 out]
                n298 = call <vilib>:"Add State(s) to Queue__jki_lib_state_machine.vi"("State(s) in Front (\"\")"="Macro: Exit", "State(s) in (\"\")"=w441) -> ("States Out"=w440:string)  [unwired: 13 in]
              }
              event Value Change {
                n299 = event-data() -> ()  [unwired: 1 in, 6 out]
                n300 = property on="Set Centriod Target" class="Bool (strict)"("Value"=FALSE) -> ()  [unwired: 2 in, 2 out]
                n301 = Unbundle By Name(w452) -> ("active ccd"=w444:i32, "Centroid X"=w443:dbl[][], "Centroid Y"=w442:dbl[][])
                n302 = Index Array(array=w448, index=w444) -> (element=w447:string)
                n303 = Concatenate Strings("Do want to update the target of " ("message"), w447, "?" ("string")) -> (w445:string)
                n304 = Two Button Dialog(message=w445) -> (T button?=w451:bool)  [unwired: 2 in]
                n305 = case shown="True" w451 {
                  tunnel: w450 -> [_ w463]
                  tunnel: w444 -> [_ w462]
                  tunnel: w443 -> [_ w469]
                  tunnel: w442 -> [_ w464]
                  frame False {
                  }
                  frame True {
                    n306 = Index Array(array=w469, index (row)=w462) -> (element=w468:dbl[])  [unwired: 1 in]
                    n307 = Index Array(array=w464, index (row)=w462) -> (element=w465:dbl[])  [unwired: 1 in]
                    n308 = Index Array(array=w463, index=w462) -> (element=w461:T30)
                    n309 = Unbundle By Name(w461) -> ("Target.X::12"=w460:refnum<vi>, "Target.Y::12"=w458:refnum<vi>)
                    n310 = Reverse 1D Array(array=w468) -> (reversed array=w467:dbl[])
                    n311 = Reverse 1D Array(array=w465) -> (reversed array=w466:dbl[])
                    n312 = Index Array(array=w467) -> (element=w459:dbl)  [unwired: 1 in]
                    n313 = Index Array(array=w466) -> (element=w457:dbl)  [unwired: 1 in]
                    n314 = property class="DigNum (strict)"(reference=w460, "Val(Sgnl)"=w459) -> ()  [unwired: 1 in, 2 out]
                    n315 = property class="DigNum (strict)"(reference=w458, "Val(Sgnl)"=w457) -> ()  [unwired: 1 in, 2 out]
                  }
                }
                n316 = call <vilib>:"Add State(s) to Queue__jki_lib_state_machine.vi"("State(s) in (\"\")"=w456) -> ("States Out"=w455:string)  [unwired: 14 in]
              }
              event "Feedback Global": Value Change {
                # "Exit Button Value Change (pressed) Event\n(this executes Macro: Exit to terminate the VI)"
                n317 = event-data() -> ("NewVal"=w472:bool)  [unwired: 1 in, 5 out]
                n318 = call <vilib>:"Add State(s) to Queue__jki_lib_state_machine.vi"("State(s) in (\"\")"=w475) -> ("States Out"=w474:string)  [unwired: 14 in]
                n319 = Bundle By Name(cluster=w471, "Feedback global"=w472) -> (w470:T36)
              }
              event Value Change {
                n320 = event-data() -> ()  [unwired: 1 in, 6 out]
                n321 = call <vilib>:"Add State(s) to Queue__jki_lib_state_machine.vi"("State(s) in Front (\"\")"="Move Config", "State(s) in (\"\")"=w480) -> ("States Out"=w479:string)  [unwired: 13 in]
              }
              event Value Change {
                n322 = event-data() -> ()  [unwired: 1 in, 6 out]
                n323 = call <vilib>:"Add State(s) to Queue__jki_lib_state_machine.vi"("State(s) in Front (\"\")"="Detection Config", "State(s) in (\"\")"=w485) -> ("States Out"=w484:string)  [unwired: 13 in]
              }
              event "associated motors": Value Change {
                n324 = event-data() -> ()  [unwired: 1 in, 6 out]
                n325 = call <vilib>:"Add State(s) to Queue__jki_lib_state_machine.vi"("State(s) in (\"\")"=w490, "State(s) at Back (\"\")"="Motor Config" ("State(s) at Back (\"\")")) -> ("States Out"=w489:string)  [unwired: 13 in]
              }
              event "Reset History": Value Change {
                n326 = event-data() -> ()  [unwired: 1 in, 6 out]
                n327 = call <vilib>:"Add State(s) to Queue__jki_lib_state_machine.vi"("State(s) in (\"\")"=w496, "State(s) at Back (\"\")"="Reset History" ("State(s) at Back (\"\")")) -> ("States Out"=w495:string)  [unwired: 13 in]
                n328 = property on="Reset History" class="Bool (strict)"("Value"=FALSE ("Reset History")) -> ()  [unwired: 2 in, 2 out]
              }
              event "ActiveMotor": Value Change {
                n329 = event-data() -> ("NewVal"=w498:u16)  [unwired: 1 in, 5 out]
                n330 = property on="ActiveMotor" class="Ring (strict)"() -> ("Strings []"=w499:string[])  [unwired: 2 in, 2 out]
                n331 = Index Array(array=w499, index=w498) -> (element=w497:string)
                n332 = property on="ActiveMotorName::99" class="Str"("Val(Sgnl)"=w497) -> ()  [unwired: 2 in, 2 out]
                n333 = call <vilib>:"Add State(s) to Queue__jki_lib_state_machine.vi"("State(s) in (\"\")"=w503) -> ("States Out"=w502:string)  [unwired: 14 in]
              }
              event "ActiveMotor 2": Value Change {
                n334 = event-data() -> ("NewVal"=w508:u16)  [unwired: 1 in, 5 out]
                n335 = property on="ActiveMotor 2" class="Ring (strict)"() -> ("Strings []"=w509:string[])  [unwired: 2 in, 2 out]
                n336 = Index Array(array=w509, index=w508) -> (element=w504:string)
                n337 = property on="ActiveMotorName::98" class="Str"("Val(Sgnl)"=w504) -> ()  [unwired: 2 in, 2 out]
              }
              event "Save Config": Value Change {
                n338 = event-data() -> ()  [unwired: 1 in, 6 out]
                n339 = call <vilib>:"Add State(s) to Queue__jki_lib_state_machine.vi"("State(s) in (\"\")"=w514, "State(s) at Back (\"\")"="Save Config" ("State(s) at Back (\"\")")) -> ("States Out"=w513:string)  [unwired: 13 in]
              }
              event "Load Config": Value Change {
                n340 = event-data() -> ()  [unwired: 1 in, 6 out]
                n341 = call "File Dialog2"("error in"=w516, "pattern (all files)"="*.cfg", "pattern label"="config") -> ("selected path"=w520:path, "error out"=w515:errorcluster)  [unwired: 9 in, 2 out]
                n342 = Path To String(path=w520) -> (string=w518:string)
                "config path" <- w518
                n343 = call <vilib>:"Build State String with Arguments__jki_lib_state_machine.vi"("Arguments (\"\")"=w518, "State"="Load Config" ("State(s) at Back (\"\")")) -> ("State with Arguments"=w517:string)  [unwired: 4 in]
                n344 = call <vilib>:"Add State(s) to Queue__jki_lib_state_machine.vi"("State(s) in (\"\")"=w525, "State(s) at Back (\"\")"=w517) -> ("States Out"=w524:string)  [unwired: 13 in]
              }
              event "Save Stats": Value Change {
                n345 = event-data() -> ()  [unwired: 1 in, 6 out]
                n346 = call <vilib>:"Add State(s) to Queue__jki_lib_state_machine.vi"("State(s) in (\"\")"=w530, "State(s) at Back (\"\")"="Save Stats" ("State(s) at Back (\"\")")) -> ("States Out"=w529:string)  [unwired: 13 in]
              }
              event "active CCDs": Value Change {
                n347 = event-data() -> ("NewVal"=w536:i32)  [unwired: 1 in, 5 out]
                n348 = Unbundle By Name(w532) -> ("active cams"=w531:string[])
                n349 = Index Array(array=w531, index=w536) -> (element=w534:string)
                n350 = call <vilib>:"Build State String with Arguments__jki_lib_state_machine.vi"("Arguments (\"\")"=w534, "State"="active" ("State(s) at Back (\"\")")) -> ("State with Arguments"=w533:string)  [unwired: 4 in]
                n351 = call <vilib>:"Add State(s) to Queue__jki_lib_state_machine.vi"("State(s) in (\"\")"=w539, "State(s) at Back (\"\")"=w533) -> ("States Out"=w538:string)  [unwired: 13 in]
              }
              event "Center": Value Change {
                n352 = event-data() -> ()  [unwired: 1 in, 6 out]
                n353 = call <vilib>:"Add State(s) to Queue__jki_lib_state_machine.vi"("State(s) in (\"\")"=w544, "State(s) at Back (\"\")"="Center" ("State(s) at Back (\"\")")) -> ("States Out"=w543:string)  [unwired: 13 in]
              }
              event "new tdms": Value Change {
                n354 = event-data() -> ()  [unwired: 1 in, 6 out]
                n355 = property on="new tdms" class="Bool (strict)"("Value"=FALSE ("new tdms")) -> ()  [unwired: 2 in, 2 out]
                n356 = call <vilib>:"Add State(s) to Queue__jki_lib_state_machine.vi"("State(s) in (\"\")"=w550, "State(s) at Back (\"\")"="newtdms" ("State(s) at Back (\"\")")) -> ("States Out"=w549:string)  [unwired: 13 in]
              }
              event "deivice ini": Value Change {
                n357 = event-data() -> ()  [unwired: 1 in, 6 out]
                n358 = property on="deivice ini" class="Bool (strict)"("Value"=FALSE ("new tdms")) -> ()  [unwired: 2 in, 2 out]
                n359 = call <vilib>:"Add State(s) to Queue__jki_lib_state_machine.vi"("State(s) in (\"\")"=w556, "State(s) at Back (\"\")"="Device Ini" ("State(s) at Back (\"\")")) -> ("States Out"=w555:string)  [unwired: 13 in]
              }
              event "Img to avg": Value Change {
                n360 = event-data() -> ()  [unwired: 1 in, 6 out]
                n361 = property on="Img to avg" class="DigNum (strict)"() -> ("Value"=w559:i32)  [unwired: 2 in, 2 out]
                n362 = Number To Decimal String(number=w559) -> (decimal integer string=w558:string)  [unwired: 1 in]
                n363 = call <vilib>:"Build State String with Arguments__jki_lib_state_machine.vi"("Arguments (\"\")"=w558, "State"="ImgToAvg" ("State(s) at Back (\"\")")) -> ("State with Arguments"=w557:string)  [unwired: 4 in]
                n364 = call <vilib>:"Add State(s) to Queue__jki_lib_state_machine.vi"("State(s) in (\"\")"=w564, "State(s) at Back (\"\")"=w557) -> ("States Out"=w563:string)  [unwired: 13 in]
              }
              event Panel Close? {
                # "Discard the event because we'll close the front panel ourselves in Macro: Exit"
                # "Close Panel button (pressed) Event\n(this executes Macro: Exit to terminate the VI)"
                n365 = event-data() -> ()  [unwired: 1 in, 1 out]
                n366 = call <vilib>:"Add State(s) to Queue__jki_lib_state_machine.vi"("State(s) in Front (\"\")"="Macro: Exit", "State(s) in (\"\")"=w570) -> ("States Out"=w569:string)  [unwired: 13 in]
                n367 = event-data("Discard?"=TRUE) -> ()  [unwired: 1 in, 1 out]
              }
            }
          }
          frame "---------- Core ----------" {
            # "Do not put any code in this frame.\n(it is a separator no-op)"
            n368 = call <vilib>:"Add State(s) to Queue__jki_lib_state_machine.vi"("State(s) in (\"\")"=w574) -> ("States Out"=w573:string)  [unwired: 14 in]
          }
          frame Default {
            w584 = 42 items=["No error", "Argument error", "Memory is full", "Out of zone", "End of file", "File already open", "Generic file I/O error", "File not found", "File permission error", "Disk is full", "Duplicate path", "Too many files open", "System feature not enabled", "Resource file not found", "Cannot add resource", "Resource not found", "Image not found", "Image memory error", "Pen does not exist", "Config type invalid", "Config token not found", "Config parse error", "Config memory error", "Bad external code format", "Bad external code offset", "External code not present", "Null window", "Destroy window error", "Null menu", "Print aborted", "Bad print record", "Print driver error", "Windows error during printing", "Memory error during printing", "Print dialog error", "Generic print error", "Invalid device refnum", "Device not found", "Device parameter error", "Device unit error", "Cannot open device", "Device call aborted", "Generic error", "Cancelled by user", "Object ID too low", "Object ID too high", "Object not in heap", "Unknown heap", "Unknown object (invalid DefProc)", "Unknown object (DefProc not in table)", "Message out of range", "Invalid (null) method", "Unknown message", "Manager call not supported", "Bad address", "Network operation in progress", "Network operation timed out", "Connection is busy", "Network attribute not supported", "Network error", "Address in use", "System out of memory", "Connection aborted", "Connection refused", "Not connected", "Already connected", "Connection closed", "Initialization error (interapplication manager)", "Bad occurrence", "Wait on unbound occurrence handler", "Occurrence queue overflow", "Datalog type conflict", "Unused", "Unrecognized type (interapplication manager)", "Memory corrupt", "Failed to make temporary DLL", "Old CIN version", "Drag socket not found", "Failed to load drop-object", "Failed to register OLE object", "Failed to release OLE object", "Format specifier type mismatch", "Unknown format specifier", "Too few format specifiers", "Too many format specifiers", "Scan failed", "Newer CIN version", "Error converting to variant", "Runtime menu error", "Password tampered", "Variant attribute not found", "Incompatible variant data type", "Event data is not available", "Event Store is not present", "Occurrence is not found", "Event Queue is not created", "Event info is not available", "Refnum passed is NULL", "Error retrieving Class GUID", "Error retrieving CoClass GUID", "Error retrieving TypeLib GUID.", "Bad built application magic bytes.", "Specific driver is different from the specific driver associated with the Logical Name.", "There is no session opened to the class driver.", "Max Error", "MAX - Error with config objects", "MAX - Error loading configuration", "MAX - Group not supported"]
            # "Current State"
            # "Do not delete, rename, or modify this frame.\n(this is used to capture unhandled states and typos)"
            # "Handle mistyped state name (developer tool)"
            n369 = Format Into String(format string="Software Exception: Unhandled State \"%s\"." ("message"), error in=w580, w575) -> (resulting string=w583:string, error out=w582:errorcluster)  [unwired: 1 in]
            n370 = call <vilib>:"Error Cluster From Error Code.vi"("show call chain? (False)"=TRUE, "error in (no error)"=w582, "error message (\"\")"=w583, "error code (0)"=w584) -> ("error out"=w581:errorcluster)  [unwired: 5 in]
            n371 = call <vilib>:"Add State(s) to Queue__jki_lib_state_machine.vi"("State(s) in (\"\")"=w579) -> ("States Out"=w578:string)  [unwired: 14 in]
          }
          frame "Initialize Core Data" {
            # "Do not delete, rename, or modify this frame.\n(this is used to determine panel behavior on exit)"
            # "originally closed?"
            # "exe?"
            # "If panel starts closed or is an EXE, then close it when we exit"
            n372 = property class="VI"() -> ("Front Panel.Open"=w594:bool)  [unwired: 2 in, 2 out]
            n373 = property class="App"() -> ("App.Kind"=w593:T16)  [unwired: 2 in, 2 out]
            n374 = control-ref of="Current VI Reference"() -> (w588:refnum<vi>)
            n375 = Not(x=w594) -> (.not. x?=w591:bool)
            n376 = Equal?(x=w593, y=T16."Run Time System" ("Application:Kind")) -> (x = y?=w590:bool)
            n377 = Or(x=w591, y=w590) -> (x .or. y?=w589:bool)
            n378 = Bundle By Name(cluster=w587, "Core.Current VI Reference"=w588, "Core.Close Panel on Exit?"=w589) -> (w586:T36)
            n379 = call <vilib>:"Add State(s) to Queue__jki_lib_state_machine.vi"("State(s) in (\"\")"=w597) -> ("States Out"=w596:string)  [unwired: 14 in]
          }
          frame "Error Handler" {
            w598 = T37 0 items=["no dialog", "OK message", "continue or stop message", "OK message + warnings", "continue/stop + warnings"] ("type of dialog (OK msg:1)")
            # "Unhandled Error -- Display it"
            # "Handle any errors here.\nYou can also output any states to clean-up after errors occur"
            # "Clear error"
            n380 = call <vilib>:"General Error Handler.vi"("type of dialog (OK msg:1)"=w598, "error in (no error)"=w600) -> ()  [unwired: 9 in, 5 out]
            n381 = call <vilib>:"Add State(s) to Queue__jki_lib_state_machine.vi"("State(s) in Front (\"\")"="/* Post Error States", "State(s) in (\"\")"=w604) -> ("States Out"=w603:string)  [unwired: 13 in]
          }
          frame "Exit" {
            # "Do not put any code in this frame.\n(No errors that occur here will be handled.)"
            n382 = call <vilib>:"Add State(s) to Queue__jki_lib_state_machine.vi"("State(s) in (\"\")"=w609) -> ("States Out"=w608:string)  [unwired: 14 in]
          }
          frame "---------- Data ----------" {
            # "Do not put any code in this frame.\n(It is a separator no-op. You can make a copy of this frame to create a new Data frame)"
            n383 = call <vilib>:"Add State(s) to Queue__jki_lib_state_machine.vi"("State(s) in (\"\")"=w613) -> ("States Out"=w612:string)  [unwired: 14 in]
          }
          frame "Data: Initialize" {
            w623 = bool[] [FALSE, FALSE, FALSE, FALSE, FALSE, FALSE, FALSE, FALSE, FALSE, FALSE, FALSE, TRUE]  # speedmode Y
            w624 = bool[] [FALSE, FALSE, FALSE, FALSE, FALSE, FALSE, FALSE, FALSE, FALSE, FALSE, FALSE, TRUE]  # speedmode X
            w625 = bool[] [FALSE, FALSE, FALSE, FALSE, TRUE, TRUE, TRUE, FALSE, FALSE, FALSE, FALSE, FALSE]  # detected
            w627 = cluster{"Lower value":sgl, "Upper value":sgl}[] [{"Lower value"=93.0, "Upper value"=255.0}, {"Lower value"=105.0, "Upper value"=255.0}, {"Lower value"=0.0, "Upper value"=255.0}, {"Lower value"=127.0, "Upper value"=255.0}, {"Lower value"=0.0, "Upper value"=255.0}, {"Lower value"=0.0, "Upper value"=255.0}, {"Lower value"=0.0, "Upper value"=255.0}, {"Lower value"=0.0, "Upper value"=255.0}, {"Lower value"=0.0, "Upper value"=255.0}, {"Lower value"=0.0, "Upper value"=255.0}, {"Lower value"=0.0, "Upper value"=255.0}, {"Lower value"=0.0, "Upper value"=255.0}]  # thresholds
            w635 = FALSE  # Feedback global
            w637 = 0  # active ccd
            w615 = 2  # img to avg
            w648 = T38 {"Current VI Reference"=refnum, "Close Panel on Exit?"=FALSE}  # Core
            # "Initialize the shift-register data, here.\n(data names are defined by what you wire into the bundle function)"
            n384 = disable-structure shown="Disabled" {
              disable-tunnel: w628 -> [w656 w660]
              disable-tunnel: w626 -> [w655 _]
              disable-tunnel: [w653 w660] -> w622
              disable-tunnel: w621 -> [w651 _]
              frame Disabled {
                n385 = TDMS Open(6:FALSE ("disable buffering (T)"), 7:enum16{"1.0", "2.0"}."2.0" ("file format version (2.0)"), 8:w656, 10:T17."create or replace" ("operation"), 11:w655) -> (0:w654:errorcluster, 3:w652:refnum<k34>)  [unwired: 2 in]
                n386 = call "TDMSbuffersize.vi"("error in (no error)"=w654, "group names"=w651, "Data Value Reference in"=w652) -> ("error out"=w653:errorcluster)  [unwired: 7 in, 1 out]
              }
              frame Enabled {
              }
            }
            n387 = call <vilib>:"Add State(s) to Queue__jki_lib_state_machine.vi"("State(s) in (\"\")"=w650) -> ("States Out"=w649:string)  [unwired: 14 in]
            n388 = Bundle("Core"=w648, "detection para"="detection para", "thresholds"=w627, "Centroid X"="Centroid X", "Centroid Y"="Centroid Y", "img to avg"=w615, "Mean Centroid X"="Mean Centroid X", "Mean Centroid Y"="Mean Centroid Y", "Offset X"="Offset X", "Offset Y"="Offset Y", "Offset X stats"="Offset X stats", "Offset Y stats"="Offset Y stats", "Size"="Size", "Mean Size"="Mean Size", "Time"="Time", "move properties"="move properties", "active axis refs 2"="active axis refs 2", "active ccd"=w637, "Feedback global"=w635, "Motor X"="Motor X", "Motor Y"="Motor Y", "active cams"="active cams", "Data Value Reference out"=refnum<k34> refnum, "detected"=w625, "speedmode X"=w624, "speedmode Y"=w623) -> (w617:T36)  [unwired: 1 in]
            n389 = Initialize Array(0.0 ("element"), 12 ("dimension size"), w615) -> (w618:dbl[][])
            n390 = Bundle By Name(cluster=w617, "Centroid X"=w618, "Centroid Y"=w618, "Size"=w618) -> (w616:T36)
          }
          frame "Data: Cleanup" {
            # "Cleanup any data and references, here.\n(this is called automatically, by the Macro: Exit)"
            n391 = Unbundle By Name(w664) -> ("Core.Current VI Reference"=w665:refnum<vi>)
            n392 = Close Reference(reference=w665, error in (no error)=w666) -> (error out=w662:errorcluster)
            n393 = Unbundle By Name(w664) -> ("Data Value Reference out"=w663:refnum<k34>)
            n394 = TDMS Close(8:w662, 11:w663) -> (0:w661:errorcluster)  [unwired: 1 out]
            n395 = call <vilib>:"Add State(s) to Queue__jki_lib_state_machine.vi"("State(s) in (\"\")"=w668) -> ("States Out"=w667:string)  [unwired: 14 in]
          }
          frame "---------- UI ----------" {
            # "Do not put any code in this frame.\n(It is a separator no-op. You can make a copy of this frame to create a new UI frame)"
            n396 = call <vilib>:"Add State(s) to Queue__jki_lib_state_machine.vi"("State(s) in (\"\")"=w672) -> ("States Out"=w671:string)  [unwired: 14 in]
          }
          frame "UI: Initialize" {
            # "Initialize the User Interface, here.\n(this is called automatically, by the Macro: Init)"
            n397 = call <vilib>:"Add State(s) to Queue__jki_lib_state_machine.vi"("State(s) in (\"\")"=w676) -> ("States Out"=w675:string)  [unwired: 14 in]
          }
          frame "UI: Cursor Set" {
            # "Argument"
            # "Set and Unset Cursor Busy.\n(Usage: \"UI: Cursor Set >> Busy|Idle\")"
            n398 = case shown="\"Idle\", Default" w677 {
              tunnel: w679 -> [w684 w686]
              tunnel: [w683 w685] -> w678
              frame "Idle", Default {
                n399 = call <vilib>:"Unset Busy.vi"("error in (no error)"=w684) -> ("error out"=w683:errorcluster)  [unwired: 10 in]
              }
              frame "Busy" {
                n400 = call <vilib>:"Set Busy.vi"("error in (no error)"=w686) -> ("error out"=w685:errorcluster)  [unwired: 9 in, 1 out]
              }
            }
            n401 = call <vilib>:"Add State(s) to Queue__jki_lib_state_machine.vi"("State(s) in (\"\")"=w682) -> ("States Out"=w681:string)  [unwired: 14 in]
          }
          frame "UI: Front Panel State" {
            # "Argument"
            # "Set Front Panel Open or Closed\n(Usage: \"UI: Front Panel State >> Open|Close\")"
            n402 = Unbundle By Name(w687) -> ("Core.Current VI Reference"=w689:refnum<vi>)
            n403 = case shown="\"Open\", Default" w688 {
              tunnel: w691 -> [w697 w708]
              tunnel: [w698 w709] -> w690
              tunnel: w689 -> [_ _]
              frame "Open", Default {
                n404 = property class="VI"(error in=w697) -> (reference out=w695:refnum<vi>, error out=w696:errorcluster, "Front Panel.Open"=w694:bool)  [unwired: 1 in]
                n405 = case shown="False" w694 {
                  tunnel: [w701 w704] -> w698
                  tunnel: w696 -> [w700 w704]
                  tunnel: w695 -> [w699 _]
                  frame False {
                    n406 = invoke class="VI" method="FP.Open"(reference=w699, error in=w700, "Activate"=TRUE, "State"=T18."Standard") -> (error out=w701:errorcluster)  [unwired: 1 in, 4 out]
                  }
                  frame True {
                  }
                }
              }
              frame "Close" {
                n407 = property class="VI"(error in=w708) -> (reference out=w706:refnum<vi>, error out=w707:errorcluster, "Front Panel.Open"=w705:bool)  [unwired: 1 in]
                n408 = case shown="True" w705 {
                  tunnel: [w710 w713] -> w709
                  tunnel: w707 -> [w710 w712]
                  tunnel: w706 -> [_ w711]
                  frame False {
                  }
                  frame True {
                    n409 = invoke class="VI" method="FP.Close"(reference=w711, error in=w712) -> (error out=w713:errorcluster)  [unwired: 1 in, 2 out]
                  }
                }
              }
            }
            n410 = call <vilib>:"Add State(s) to Queue__jki_lib_state_machine.vi"("State(s) in (\"\")"=w693) -> ("States Out"=w692:string)  [unwired: 14 in]
          }
          frame "---------- Macro ----------" {
            # "Do not put any code in this frame.\n(It is a separator no-op. You can make a copy of this frame to create a new Macro frame)"
            n411 = call <vilib>:"Add State(s) to Queue__jki_lib_state_machine.vi"("State(s) in (\"\")"=w717) -> ("States Out"=w716:string)  [unwired: 14 in]
          }
          frame "Macro: Initialize" {
            w724 = "Data: Initialize\nInitialize Core Data\nUI: Initialize\nUI: Front Panel State >> Open\nDevice Ini >> 3000\nnewtdms"  # Data: Initialize Initialize Core Data UI: Initialize UI: Front Panel State >> Open Device Ini >> 3000 newtdms
            # "Initialization Macro\n(This is called once, when the VI starts)"
            n412 = property on="Img to avg" class="DigNum (strict)"() -> ("Value"=w722:i32)  [unwired: 2 in, 2 out]
            n413 = call <vilib>:"Add State(s) to Queue__jki_lib_state_machine.vi"("State(s) in Front (\"\")"=w724, "State(s) in (\"\")"=w727) -> ("States Out"=w719:string)  [unwired: 13 in]
            n414 = Number To Decimal String(number=w722) -> (decimal integer string=w721:string)  [unwired: 1 in]
            n415 = call <vilib>:"Build State String with Arguments__jki_lib_state_machine.vi"("Arguments (\"\")"=w721, "State"="ImgToAvg") -> ("State with Arguments"=w720:string)  [unwired: 4 in]
            n416 = call <vilib>:"Add State(s) to Queue__jki_lib_state_machine.vi"("State(s) in (\"\")"=w719, "State(s) at Back (\"\")"=w720) -> ("States Out"=w718:string)  [unwired: 13 in]
          }
          frame "Macro: Exit" {
            # "Exit Macro\n(This is called once, when the VI exits)"
            n417 = Unbundle By Name(w729) -> ("Core.Close Panel on Exit?"=w728:bool)
            n418 = Select(t="UI: Front Panel State >> Close", s=w728, f="") -> (s? t:f=w732:string)
            n419 = call <vilib>:"Add State(s) to Queue__jki_lib_state_machine.vi"("State(s) in (\"\")"=w732, "State(s) at Back (\"\")"="Data: Cleanup\nExit") -> ("States Out"=w730:string)  [unwired: 13 in]
            n420 = call <vilib>:"Add State(s) to Queue__jki_lib_state_machine.vi"("State(s) in Front (\"\")"=w730, "State(s) in (\"\")"=w737) -> ("States Out"=w736:string)  [unwired: 13 in]
          }
          frame "---------- Ini and Configure ----------" {
            # "Template Separator\n(You can make a copy of, or modify, this frame)"
            n421 = call <vilib>:"Add State(s) to Queue__jki_lib_state_machine.vi"("State(s) in (\"\")"=w741) -> ("States Out"=w740:string)  [unwired: 14 in]
          }
          frame "Device Ini" {
            # "Your code here.\n(You can make a copy of, or modify, this frame)"
            n422 = Empty String/Path?(string/path=w758) -> (empty?=w756:bool)
            n423 = case shown="False" w756 {
              tunnel: w758 -> [w795 _]
              tunnel: [w794 0] -> w757
              frame False {
                n424 = Decimal String To Number(string=w795) -> (number=w794:i32)  [unwired: 2 in, 1 out]
              }
              frame True {
              }
            }
            n425 = flat-sequence {
              tunnel: w762 -> [w798]
              tunnel: [w798] -> w761
              tunnel: w757 -> [w797]
              tunnel: w761 -> [w801]
              tunnel: [w799] -> w747
              frame #0 {
                n426 = Wait (ms)(milliseconds to wait=w797) -> ()  [unwired: 1 out]
              }
              frame #1 {
                n427 = for {
                  tunnel: w801 -> [w803] mode=indexing
                  shift-right: [w804] -> w799
                  shift-left: string[] [] -> [w805]
                  n428 = Empty String/Path?(string/path=w803) -> (empty?=w802:bool)
                  n429 = case shown="False" w802 {
                    tunnel: w805 -> [w808 w814]
                    tunnel: [w807 w814] -> w804
                    tunnel: w803 -> [w806 _]
                    frame False {
                      n430 = call "send command.vi"("Device Name"=w806) -> ("status"=w809:bool)  [unwired: 4 in]
                      n431 = case shown="True" w809 {
                        tunnel: w808 -> [w810 w813]
                        tunnel: [w810 w812] -> w807
                        tunnel: w806 -> [_ w811]
                        frame False {
                        }
                        frame True {
                          n432 = Build Array (concatenate)(w813, w811) -> (w812:string[])
                        }
                      }
                    }
                    frame True {
                    }
                  }
                }
              }
            }
            n433 = Unbundle By Name(w755) -> ("active cams"=w748:string[])
            n434 = call <vilib>:"Add State(s) to Queue__jki_lib_state_machine.vi"("State(s) in (\"\")"=w763) -> ("States Out"=w750:string)  [unwired: 14 in]
            n435 = Empty Array?(array=w748) -> (empty?=w752:bool)
            n436 = Equal?(x=w748, y=w747) -> (x = y?=w753:bool[])
            n437 = Not(x=w752) -> (.not. x?=w751:bool)
            n438 = Build Array (concatenate)(w753, w751) -> (w754:bool[])
            n439 = Array Size(array=w747) -> (size(s)=w745:i32)
            n440 = Array Size(array=w748) -> (size(s)=w746:i32)
            n441 = Equal?(x=w746, y=w745) -> (x = y?=w744:bool)
            n442 = And Array Elements(Boolean array=w754) -> (logical AND=w743:bool)
            n443 = And(x=w744, y=w743) -> (x .and. y?=w742:bool)
            n444 = case shown="False" w742 {
              tunnel: [w780 w793] -> w760
              tunnel: w755 -> [w765 w793]
              tunnel: w747 -> [w766 _]
              tunnel: w750 -> [w775 w792]
              tunnel: [w773 w792] -> w749
              frame False {
                n445 = Bundle By Name(cluster=w765, "active cams"=w766) -> (w781:T36)
                n446 = property on="active CCDs" class="LstBox (strict)"("Item Names"=w766) -> ()  [unwired: 2 in, 2 out]
                n447 = Array Size(array=w766) -> (size(s)=w784:i32)
                n448 = for {
                  N: 1 -> [_]
                  shift-right: [w786] -> w779
                  shift-left: timestamp[][] [] ("Time") -> [w788]
                  n449 = for {
                    N: 12 -> [_]
                    tunnel: w788 -> [w791] mode=indexing
                    tunnel: [w789] -> w786 mode=indexing
                    n450 = Get Date/Time In Seconds() -> (seconds since 1Jan1904=w790:timestamp)
                    n451 = Build Array (concatenate)(w791, w790) -> (w789:timestamp[])
                  }
                }
                n452 = Unbundle By Name(w765) -> ("img to avg"=w764:i32)
                n453 = Initialize Array(0.0 ("element"), w784, 0 ("dimension size")) -> (w782:dbl[][])
                n454 = Initialize Array(0.0 ("element"), 12 ("dimension size"), w764) -> (w767:dbl[][])
                n455 = Bundle By Name(cluster=w781, "Offset X stats"=w782, "Offset Y stats"=w782, "Centroid X"=w767, "Centroid Y"=w767, "Mean Centroid X"=w782, "Mean Centroid Y"=w782, "Offset X"=w782, "Offset Y"=w782, "Size"=w767, "Mean Size"=w782, "Motor X"=w782, "Motor Y"=w782) -> (w780:T36)
                n456 = property on="Time" class="Arr (strict)"("Value"=w779) -> ()  [unwired: 2 in, 2 out]
                n457 = property on="config path" class="Str"() -> ("Value"=w772:string)  [unwired: 2 in, 2 out]
                n458 = call <vilib>:"Add State(s) to Queue__jki_lib_state_machine.vi"("State(s) in Front (\"\")"="newtdms\nMove Config\nDetection Config\nactive\nCenter" ("State(s) in Front (\"\")"), "State(s) in (\"\")"=w775) -> ("States Out"=w774:string)  [unwired: 13 in]
                n459 = call <vilib>:"Build State String with Arguments__jki_lib_state_machine.vi"("Arguments (\"\")"=w772, "State"="Load Config" ("State(s) in Front (\"\")")) -> ("State with Arguments"=w770:string)  [unwired: 4 in]
                n460 = call <vilib>:"Add State(s) to Queue__jki_lib_state_machine.vi"("State(s) in Front (\"\")"=w770, "State(s) in (\"\")"=w774) -> ("States Out"=w773:string)  [unwired: 13 in]
                "name array" <- w766
              }
              frame True {
              }
            }
          }
          frame "Load Config" {
            # "Your code here.\n(You can make a copy of, or modify, this frame)"
            n461 = Unbundle By Name(w817) -> ("detection para"=w860:T3[], "move properties"=w857:T2[], "thresholds"=w852:cluster{"Lower value":sgl, "Upper value":sgl}[])
            n462 = Empty String/Path?(string/path=w816) -> (empty?=w815:bool)
            n463 = property on="Load Config" class="Bool (strict)"("Value"=FALSE ("Load Config")) -> ()  [unwired: 2 in, 2 out]
            n464 = case shown="False" w815 {
              tunnel: [w871 T5 {"CCDs"=[], "move properties"=[], "detection para"=[], "thresholds"=[], "Value"={"Motor CCD 1"=0, "Motor CCD 2"=0, "Motor CCD 3"=0, "Motor CCD 4"=0, "Motor CCD 5"=0, "Motor CCD 6"=0, "Motor CCD 7"=0, "Motor CCD 8"=0, "Motor CCD 9"=0, "Motor CCD 10"=0, "Motor CCD 11"=0, "Motor CCD 12"=0}} ("output cluster 2")] -> w862
              tunnel: [w869 w878] -> w822
              tunnel: w816 -> [w868 _]
              tunnel: w819 -> [w866 w878]
              tunnel: w817 -> [_ _]
              frame False {
                n465 = String To Path(string=w868) -> (path=w867:path)
                n466 = Open/Create/Replace File(file path (use dialog)=w867, error in=w866, operation (0:open)=T19."open or create") -> (refnum out=w873:refnum<file>, error out=w874:errorcluster)  [unwired: 3 in, 1 out]
                n467 = Read from Binary File(5:"output cluster 2", 8:w874, 11:w873) -> (0:w875:errorcluster, 2:w871:T5, 3:w876:refnum<file>)  [unwired: 3 in, 1 out]
                n468 = Close File(refnum=w876, error in=w875) -> (error out=w869:errorcluster)  [unwired: 1 out]
              }
              frame True {
              }
            }
            n469 = Unbundle By Name(w862) -> ("Value"=w849:T7, "CCDs"=w861:string[], "detection para"=w859:T3[], "move properties"=w858:T2[], "thresholds"=w853:cluster{"Lower value":sgl, "Upper value":sgl}[])
            n470 = Cluster To Array(cluster=w849) -> (array=w850:u16[])
            n471 = call <vilib>:"Add State(s) to Queue__jki_lib_state_machine.vi"("State(s) in (\"\")"=w865, "State(s) at Back (\"\")"="Motor Config" ("State(s) at Back (\"\")")) -> ("States Out"=w864:string)  [unwired: 13 in]
            n472 = for {
              tunnel: w861 -> [w894]
              tunnel: w859 -> [w896]
              tunnel: w858 -> [w895]
              shift-right: [w888] -> w856
              shift-left: w860 -> [w893]
              shift-right: [w886] -> w855
              shift-left: w857 -> [w892]
              tunnel: w818 -> [w891] mode=indexing
              tunnel: w853 -> [w887]
              shift-right: [w883] -> w851
              shift-left: w852 -> [w885]
              tunnel: w850 -> [w882]
              tunnel: [w879] -> w848 mode=indexing
              i -> [w880]
              n473 = call-poly <userlib>:"Filter 1D Array__ogtk.vi"("items to filter"=w891, "array"=w894) -> ("filtered item indices"=w897:i32[])  [unwired: 4 in, 1 out]
              n474 = Index Array(array=w897) -> (element=w881:i32)  [unwired: 1 in]
              n475 = Index Array(array=w882, index=w881) -> (element=w879:u16)
              n476 = Index Array(array=w896, index=w881) -> (element=w890:T3)
              n477 = Index Array(array=w895, index=w881) -> (element=w889:T2)
              n478 = Index Array(array=w887, index=w881) -> (element=w884:cluster{"Lower value":sgl, "Upper value":sgl})
              n479 = Replace Array Subset(array=w893, new element=w890, index=w880) -> (w888:T3[])
              n480 = Replace Array Subset(array=w892, new element=w889, index=w880) -> (w886:T2[])
              n481 = Replace Array Subset(array=w885, new element=w884, index=w880) -> (w883:cluster{"Lower value":sgl, "Upper value":sgl}[])
            }
            n482 = Index Array(array=w848, index #1=0 ("index (row)"), index #2=1 ("index (row)"), index #3=2 ("index (row)"), index #4=3 ("index (row)"), index #5=4 ("index (row)"), index #6=5 ("index (row)"), index #7=6 ("index (row)"), index #8=7 ("index (row)"), index #9=8 ("index (row)"), index #10=9 ("index (row)"), index #11=10 ("index (row)"), index #12=11 ("index (row)")) -> (element #1=w835:u16, element #2=w834:u16, element #3=w833:u16, element #4=w832:u16, element #5=w831:u16, element #6=w830:u16, element #7=w829:u16, element #8=w828:u16, element #9=w827:u16, element #10=w826:u16, element #11=w825:u16, element #12=w824:u16)
            n483 = Bundle By Name(cluster=w849, "Motor CCD 1"=w835, "Motor CCD 2"=w834, "Motor CCD 3"=w833, "Motor CCD 4"=w832, "Motor CCD 5"=w831, "Motor CCD 6"=w830, "Motor CCD 7"=w829, "Motor CCD 8"=w828, "Motor CCD 9"=w827, "Motor CCD 10"=w826, "Motor CCD 11"=w825, "Motor CCD 12"=w824) -> (w823:T7)
            n484 = Bundle By Name(cluster=w817, "detection para"=w856, "move properties"=w855, "thresholds"=w851) -> (w854:T36)
            n485 = property on="associated motors" class="Clust (strict)"(error in=w822, "Val(Sgnl)"=w823) -> (error out=w821:errorcluster)  [unwired: 1 in, 1 out]
          }
          frame "Save Config" {
            # "Your code here.\n(You can make a copy of, or modify, this frame)"
            n486 = Unbundle By Name(w916) -> ("move properties"=w903:T2[], "detection para"=w911:T3[], "thresholds"=w900:cluster{"Lower value":sgl, "Upper value":sgl}[])
            n487 = property on="associated motors" class="Clust (strict)"() -> ("Value"=w910:T7)  [unwired: 2 in, 2 out]
            n488 = property on="Save Config" class="Bool (strict)"("Value"=FALSE ("Save Config")) -> ()  [unwired: 2 in, 2 out]
            n489 = local read "CCDs"() -> (w901:string[])
            n490 = call "File Dialog"("error in"=w899, "pattern (all files)"="*.cfg", "pattern label"="config") -> ("selected path"=w905:path, "error out"=w898:errorcluster)  [unwired: 9 in, 2 out]
            n491 = Bundle("CCDs"=w901, "move properties"=w903, "detection para"=w911, "thresholds"=w900, "Value"=w910) -> (w904:T5)  [unwired: 1 in]
            n492 = Open/Create/Replace File(file path (use dialog)=w905, error in=w898, operation (0:open)=T19."replace or create with confirmation") -> (refnum out=w912:refnum<file>, error out=w913:errorcluster)  [unwired: 3 in, 1 out]
            n493 = Write to Binary File(file (use dialog)=w912, data=w904, error in=w913) -> (refnum out=w915:refnum<file>, error out=w914:errorcluster)  [unwired: 3 in, 1 out]
            n494 = Close File(refnum=w915, error in=w914) -> (error out=w908:errorcluster)  [unwired: 1 out]
            n495 = call <vilib>:"Add State(s) to Queue__jki_lib_state_machine.vi"("State(s) in (\"\")"=w918) -> ("States Out"=w917:string)  [unwired: 14 in]
          }
          frame "active" {
            # "Your code here.\n(You can make a copy of, or modify, this frame)"
            n496 = call-poly <userlib>:"Filter 1D Array__ogtk.vi"("items to filter"=w928, "array"=w924) -> ("filtered item indices"=w927:i32[])  [unwired: 4 in, 1 out]
            n497 = Unbundle By Name(w923) -> ("move properties"=w926:T2[], "detection para"=w921:T3[])  [unwired: 1 out]
            n498 = Index Array(array=w927) -> (element=w919:i32)  [unwired: 1 in]
            n499 = Index Array(array=w926, index=w919) -> (element=w925:T2)
            n500 = Index Array(array=w921, index=w919) -> (element=w920:T3)
            n501 = property on="move config" class="Clust (strict)"("Value"=w925) -> ()  [unwired: 2 in, 2 out]
            n502 = property on="beam detection para" class="Clust (strict)"("Value"=w920) -> ()  [unwired: 2 in, 2 out]
            n503 = Bundle By Name(cluster=w923, "active ccd"=w919) -> (w922:T36)
            n504 = call <vilib>:"Add State(s) to Queue__jki_lib_state_machine.vi"("State(s) in (\"\")"=w931) -> ("States Out"=w930:string)  [unwired: 14 in]
          }
          frame "Detection Config" {
            # "Your code here.\n(You can make a copy of, or modify, this frame)"
            n505 = Unbundle By Name(w936) -> ("detection para"=w932:T3[], "active ccd"=w937:i32)
            n506 = Replace Array Subset(array=w932, new element="beam detection para", index=w937) -> (w933:T3[])
            n507 = Bundle By Name(cluster=w936, "detection para"=w933) -> (w935:T36)
            n508 = call <vilib>:"Add State(s) to Queue__jki_lib_state_machine.vi"("State(s) in (\"\")"=w940) -> ("States Out"=w939:string)  [unwired: 14 in]
          }
          frame "Motor Config" {
            # "Your code here.\n(You can make a copy of, or modify, this frame)"
            n509 = Unbundle By Name("associated motors") -> ("Motor CCD 1"=w962:u16, "Motor CCD 2"=w963:u16, "Motor CCD 3"=w964:u16, "Motor CCD 4"=w957:u16, "Motor CCD 5"=w956:u16, "Motor CCD 6"=w955:u16, "Motor CCD 7"=w954:u16, "Motor CCD 8"=w953:u16, "Motor CCD 9"=w952:u16, "Motor CCD 10"=w951:u16, "Motor CCD 11"=w950:u16, "Motor CCD 12"=w949:u16)
            n510 = local read "motor refs"() -> (w960:refnum<vi>[])
            n511 = property on="ActiveMotor" class="Ring (strict)"() -> ("Value"=w943:u16)  [unwired: 2 in, 2 out]
            n512 = property on="ActiveMotor" class="Ring (strict)"() -> ("Strings []"=w945:string[])  [unwired: 2 in, 2 out]
            n513 = Build Array(w962, w963, w964, w957, w956, w955, w954, w953, w952, w951, w950, w949) -> (w948:u16[])
            n514 = Increment(x=w948) -> (x+1=w947:u16[])
            n515 = Index Array(array=w945, index=w943) -> (element=w944:string)
            n516 = for {
              tunnel: w947 -> [w979] mode=indexing
              tunnel: w960 -> [w974]
              tunnel: [w970] -> w946 mode=indexing
              tunnel: [w969] -> w942 mode=indexing
              tunnel: [w968] -> w941 mode=indexing
              n517 = Multiply(x=w979, y=u16 3) -> (x*y=w975:u16)
              n518 = Subtract(x=w975, y=u16 3) -> (x-y=w969:u16)
              n519 = Subtract(x=w975, y=u16 2) -> (x-y=w968:u16)
              n520 = Index Array(array=w974, index=w969) -> (element=w973:refnum<vi>)
              n521 = Index Array(array=w974, index=w968) -> (element=w972:refnum<vi>)
              n522 = Bundle By Name(cluster="active Axis ref", "Ref X"=w973, "Ref Y"=w972) -> (w970:cluster{"Ref X":refnum<vi>, "Ref Y":refnum<vi>})
            }
            "Array" <- w942
            "Array 2" <- w941
            n523 = property on="ActiveMotorName::99" class="Str"("Val(Sgnl)"=w944) -> ()  [unwired: 2 in, 2 out]
            n524 = call <vilib>:"Add State(s) to Queue__jki_lib_state_machine.vi"("State(s) in (\"\")"=w967) -> ("States Out"=w966:string)  [unwired: 14 in]
            n525 = Bundle By Name(cluster=w959, "active axis refs 2"=w946) -> (w958:T36)
          }
          frame "Move Config" {
            # "Your code here.\n(You can make a copy of, or modify, this frame)"
            n526 = Unbundle By Name(w981) -> ("move properties"=w985:T2[], "active ccd"=w984:i32)
            n527 = Replace Array Subset(array=w985, new element="move config", index=w984) -> (w982:T2[])
            n528 = Bundle By Name(cluster=w981, "move properties"=w982) -> (w980:T36)
            n529 = call <vilib>:"Add State(s) to Queue__jki_lib_state_machine.vi"("State(s) in (\"\")"=w988) -> ("States Out"=w987:string)  [unwired: 14 in]
          }
          frame "----------Centroid & Move----------" {
            # "Template Separator\n(You can make a copy of, or modify, this frame)"
            n530 = call <vilib>:"Add State(s) to Queue__jki_lib_state_machine.vi"("State(s) in (\"\")"=w992) -> ("States Out"=w991:string)  [unwired: 14 in]
          }
          frame "detected" {
            n531 = Unbundle By Name(w995) -> ("Offset X"=w1037:dbl[][], "Offset Y"=w1036:dbl[][], "Size"=w1035:dbl[][], "Mean Size"=w1034:dbl[][], "Time"=w1031:timestamp[][], "Motor X"=w1009:dbl[][], "active axis refs 2"=w1008:T12, "Motor Y"=w1007:dbl[][])
            n532 = Spreadsheet String To Array(format string="%s", spreadsheet string=w1013, array type (2D Dbl)=string[] []) -> (array=w1002:string[])  [unwired: 1 in]
            n533 = call-poly <userlib>:"Filter 1D Array__ogtk.vi"("items to filter"=w1002, "array"=w1003) -> ("filtered item indices"=w1000:i32[])  [unwired: 4 in, 1 out]
            n534 = for {
              tunnel: w1003 -> [w1054] mode=indexing
              tunnel: w1002 -> [w1053]
              tunnel: [w1051] -> w1004 mode=indexing
              n535 = for {
                tunnel: w1054 -> [w1057]
                tunnel: [w1056] -> w1052 mode=indexing
                tunnel: w1053 -> [w1055] mode=indexing
                n536 = Equal?(x=w1057, y=w1055) -> (x = y?=w1056:bool)
              }
              n537 = Or Array Elements(Boolean array=w1052) -> (logical OR=w1051:bool)
            }
            n538 = for {
              N: 12 -> [_]
              tunnel: w1000 -> [w1050]
              tunnel: [w1047] -> w999 mode=indexing
              i -> [w1049]
              n539 = Equal?(x=w1050, y=w1049) -> (x = y?=w1048:bool[])
              n540 = Or Array Elements(Boolean array=w1048) -> (logical OR=w1047:bool)
            }
            "Array 3" <- w999
            n541 = call <vilib>:"Build State String with Arguments__jki_lib_state_machine.vi"("Arguments (\"\")"=w1013, "State"="stats") -> ("State with Arguments"=w1012:string)  [unwired: 4 in]
            n542 = Unbundle By Name(w995) -> ("Mean Centroid X"=w1042:dbl[][], "Mean Centroid Y"=w1041:dbl[][], "Centroid X"=w1044:dbl[][], "Centroid Y"=w1043:dbl[][])
            n543 = call <vilib>:"Add State(s) to Queue__jki_lib_state_machine.vi"("State(s) in (\"\")"=w1011, "State(s) at Back (\"\")"=w1012) -> ("States Out"=w1010:string)  [unwired: 13 in]
            n544 = for {
              tunnel: w1044 -> [w1107]
              tunnel: w1043 -> [w1106]
              tunnel: w1042 -> [w1105]
              tunnel: w1041 -> [w1104]
              tunnel: [w1103] -> w1028 mode=indexing
              tunnel: [w1102] -> w1039 mode=indexing
              tunnel: w1038 -> [w1075] mode=indexing
              tunnel: w1037 -> [w1101]
              tunnel: w1036 -> [w1100]
              tunnel: [w1099] -> w1016 mode=indexing
              tunnel: [w1098] -> w1029 mode=indexing
              tunnel: w1035 -> [w1097]
              tunnel: w1034 -> [w1096]
              tunnel: [w1095] -> w1033 mode=indexing
              tunnel: w1031 -> [w1094]
              tunnel: [w1093] -> w1030 mode=indexing
              tunnel: w1009 -> [w1067]
              tunnel: w1008 -> [w1066]
              tunnel: w1007 -> [w1065]
              tunnel: [w1064] -> w1006 mode=indexing
              tunnel: [w1063] -> w1005 mode=indexing
              tunnel: w1004 -> [w1062]
              i -> [w1061]
              n545 = Unbundle By Name(w1075) -> ("Target.X::12"=w1078:refnum<vi>, "Target.Y::12"=w1077:refnum<vi>)
              n546 = Index Array(array=w1067, index (row)=w1061) -> (element=w1070:dbl[])  [unwired: 1 in]
              n547 = Index Array(array=w1066, index=w1061) -> (element=w1069:cluster{"Ref X":refnum<vi>, "Ref Y":refnum<vi>})
              n548 = Index Array(array=w1065, index (row)=w1061) -> (element=w1074:dbl[])  [unwired: 1 in]
              n549 = Index Array(array=w1105, index (row)=w1061) -> (element=w1089:dbl[])  [unwired: 1 in]
              n550 = Index Array(array=w1104, index (row)=w1061) -> (element=w1090:dbl[])  [unwired: 1 in]
              n551 = Index Array(array=w1107, index (row)=w1061) -> (element=w1092:dbl[])  [unwired: 1 in]
              n552 = Index Array(array=w1106, index (row)=w1061) -> (element=w1091:dbl[])  [unwired: 1 in]
              n553 = Index Array(array=w1101, index (row)=w1061) -> (element=w1086:dbl[])  [unwired: 1 in]
              n554 = Index Array(array=w1100, index (row)=w1061) -> (element=w1085:dbl[])  [unwired: 1 in]
              n555 = Index Array(array=w1097, index (row)=w1061) -> (element=w1083:dbl[])  [unwired: 1 in]
              n556 = Index Array(array=w1096, index (row)=w1061) -> (element=w1082:dbl[])  [unwired: 1 in]
              n557 = Index Array(array=w1094, index (row)=w1061) -> (element=w1079:timestamp[])  [unwired: 1 in]
              n558 = Index Array(array=w1062, index=w1061) -> (element=w1060:bool)
              n559 = Unbundle By Name(w1069) -> ("Ref X"=w1068:refnum<vi>, "Ref Y"=w1072:refnum<vi>)
              n560 = property class="DigNum (strict)"(reference=w1078) -> ("Value"=w1059:dbl)  [unwired: 1 in, 2 out]
              n561 = property class="DigNum (strict)"(reference=w1077) -> ("Value"=w1076:dbl)  [unwired: 1 in, 2 out]
              n562 = call <vilib>:"Std Deviation and Variance.vi"("X"=w1092) -> ("mean"=w1058:dbl)  [unwired: 1 in, 2 out]
              n563 = call <vilib>:"Std Deviation and Variance.vi"("X"=w1091) -> ("mean"=w1088:dbl)  [unwired: 1 in, 2 out]
              n564 = call <vilib>:"Std Deviation and Variance.vi"("X"=w1083) -> ("mean"=w1081:dbl)  [unwired: 1 in, 2 out]
              n565 = Get Date/Time In Seconds() -> (seconds since 1Jan1904=w1080:timestamp)
              n566 = property class="DigNum (strict)"(reference=w1068) -> ("Value"=w1071:dbl)  [unwired: 1 in, 2 out]
              n567 = property class="DigNum (strict)"(reference=w1072) -> ("Value"=w1073:dbl)  [unwired: 1 in, 2 out]
              n568 = Subtract(x=w1059, y=w1058) -> (x-y=w1087:dbl)
              n569 = Subtract(x=w1076, y=w1088) -> (x-y=w1084:dbl)
              n570 = case shown="True" w1060 {
                tunnel: [w1125 w1139] -> w1103
                tunnel: [w1124 w1138] -> w1102
                tunnel: [w1123 w1137] -> w1099
                tunnel: [w1122 w1136] -> w1098
                tunnel: [w1121 w1135] -> w1095
                tunnel: [w1120 w1134] -> w1093
                tunnel: w1090 -> [w1119 w1133]
                tunnel: w1089 -> [w1118 w1132]
                tunnel: w1058 -> [w1117 _]
                tunnel: w1088 -> [w1116 _]
                tunnel: w1087 -> [w1115 _]
                tunnel: w1086 -> [w1114 w1131]
                tunnel: w1085 -> [w1113 w1130]
                tunnel: w1084 -> [w1112 _]
                tunnel: w1082 -> [w1111 w1129]
                tunnel: w1081 -> [w1110 _]
                tunnel: w1080 -> [w1109 w1128]
                tunnel: w1079 -> [w1108 w1127]
                frame True {
                  n571 = Build Array (concatenate)(w1118, w1117) -> (w1125:dbl[])
                  n572 = Build Array (concatenate)(w1119, w1116) -> (w1124:dbl[])
                  n573 = Build Array (concatenate)(w1114, w1115) -> (w1123:dbl[])
                  n574 = Build Array (concatenate)(w1113, w1112) -> (w1122:dbl[])
                  n575 = Build Array (concatenate)(w1111, w1110) -> (w1121:dbl[])
                  n576 = Build Array (concatenate)(w1108, w1109) -> (w1120:timestamp[])
                }
                frame False {
                  w1126 = 0.0
                  n577 = Build Array (concatenate)(w1132, w1126) -> (w1139:dbl[])
                  n578 = Build Array (concatenate)(w1133, w1126) -> (w1138:dbl[])
                  n579 = Build Array (concatenate)(w1131, w1126) -> (w1137:dbl[])
                  n580 = Build Array (concatenate)(w1130, w1126) -> (w1136:dbl[])
                  n581 = Build Array (concatenate)(w1129, w1126) -> (w1135:dbl[])
                  n582 = Build Array (concatenate)(w1127, w1128) -> (w1134:timestamp[])
                }
              }
              n583 = Build Array (concatenate)(w1074, w1073) -> (w1063:dbl[])
              n584 = Build Array (concatenate)(w1070, w1071) -> (w1064:dbl[])
            }
            n585 = local write "Numeric"(0.0 ("Numeric")) -> ()
            n586 = Array Size(array=w1016) -> (size(s)=w1027:i32[])
            n587 = Index Array(array=w1027, index=1) -> (element=w1025:i32)
            "History index" <- w1025
            n588 = call <vilib>:"Add State(s) to Queue__jki_lib_state_machine.vi"("State(s) in (\"\")"=w1010, "State(s) at Back (\"\")"="Check Move\ntdms" ("State(s) at Back (\"\")")) -> ("States Out"=w1019:string)  [unwired: 13 in]
            n589 = Unbundle By Name(w995) -> ("img to avg"=w994:i32)
            n590 = Decrement(x=w994) -> (x-1=w993:i32)
            n591 = Initialize Array(0.0 ("element"), 12 ("dimension size"), w993) -> (w996:dbl[][])
            n592 = Greater?(x=w1025, y="History Size") -> (0:w1023:bool)
            n593 = Bundle By Name(cluster=w995, "Centroid X"=w996, "Centroid Y"=w996, "Mean Centroid X"=w1028, "Mean Centroid Y"=w1039, "Offset X"=w1016, "Offset Y"=w1029, "Mean Size"=w1033, "Size"=w996, "Time"=w1030, "Motor X"=w1006, "Motor Y"=w1005) -> (w1040:T36)
            n594 = Select(t="history" ("State(s) at Back (\"\")"), s=w1023, f="") -> (s? t:f=w1020:string)
            n595 = call <vilib>:"Add State(s) to Queue__jki_lib_state_machine.vi"("State(s) in (\"\")"=w1019, "State(s) at Back (\"\")"=w1020) -> ("States Out"=w1018:string)  [unwired: 13 in]
          }
          frame "Check Move" {
            (unwired) "Device Ini" ("State(s) in Front (\"\")")
            # "Your code here.\n(You can make a copy of, or modify, this frame)"
            n596 = Unbundle By Name(w1144) -> ("move properties"=w1147:T2[], "Mean Size"=w1170:dbl[][], "move properties"=w1173:T2[], "Offset X"=w1172:dbl[][], "Offset Y"=w1171:dbl[][], "active cams"=w1151:string[])
            n597 = for {
              tunnel: w1173 -> [w1238]
              tunnel: w1172 -> [w1237]
              tunnel: w1171 -> [w1236]
              tunnel: w1170 -> [w1239]
              tunnel: [w1255] -> w1169 mode=indexing
              tunnel: [w1251] -> w1168 mode=indexing
              tunnel: w1151 -> [w1241] mode=indexing
              tunnel: [w1273] -> w1167 mode=indexing
              tunnel: [w1272] -> w1166 mode=indexing
              tunnel: w1147 -> [w1231]
              tunnel: [w1249] -> w1145 mode=indexing
              tunnel: [w1244] -> w1141 mode=indexing
              tunnel: "Speedmode @" -> [w1243]
              tunnel: w1140 -> [w1242]
              n598 = call-poly <userlib>:"Filter 1D Array__ogtk.vi"("items to filter"=w1241, "array"=w1242) -> ("filtered item indices"=w1240:i32[])  [unwired: 4 in, 1 out]
              n599 = Index Array(array=w1240) -> (element=w1230:i32)  [unwired: 1 in]
              n600 = Index Array(array=w1239, index (row)=w1230) -> (element=w1235:dbl[])  [unwired: 1 in]
              n601 = Index Array(array=w1238, index=w1230) -> (element=w1234:T2)
              n602 = Index Array(array=w1237, index (row)=w1230) -> (element=w1233:dbl[])  [unwired: 1 in]
              n603 = Index Array(array=w1231, index=w1230) -> (element=w1229:T2)
              n604 = Index Array(array=w1236, index (row)=w1230) -> (element=w1232:dbl[])  [unwired: 1 in]
              n605 = Unbundle By Name(w1234) -> ("Tolerance [%]"=w1266:dbl)
              n606 = Reverse 1D Array(array=w1233) -> (reversed array=w1271:dbl[])
              n607 = Reverse 1D Array(array=w1232) -> (reversed array=w1270:dbl[])
              n608 = Reverse 1D Array(array=w1235) -> (reversed array=w1265:dbl[])
              n609 = Unbundle By Name(w1229) -> ("enable feedback"=w1254:bool)
              n610 = Index Array(array=w1271) -> (element=w1269:dbl)  [unwired: 1 in]
              n611 = Index Array(array=w1270) -> (element=w1268:dbl)  [unwired: 1 in]
              n612 = Index Array(array=w1265) -> (element=w1264:dbl)  [unwired: 1 in]
              n613 = Absolute Value(x=w1269) -> (abs(x)=w1250:dbl)
              n614 = Absolute Value(x=w1268) -> (abs(x)=w1247:dbl)
              n615 = Square Root(x=w1264) -> (sqrt(x)=w1263:dbl)
              n616 = Divide(x=w1266, y=100.0) -> (x/y=w1262:dbl)
              n617 = Multiply(x=w1263, y=w1262) -> (x*y=w1246:dbl)
              n618 = Not Equal To 0?(x=w1247) -> (x != 0?=w1252:bool)
              n619 = Not Equal To 0?(x=w1250) -> (x != 0?=w1257:bool)
              n620 = Greater Or Equal?(x=w1250, y=w1246) -> (x >= y?=w1256:bool)
              n621 = Greater Or Equal?(x=w1247, y=w1246) -> (x >= y?=w1253:bool)
              n622 = Divide(x=w1250, y=w1246) -> (x/y=w1248:dbl)
              n623 = Divide(x=w1247, y=w1246) -> (x/y=w1245:dbl)
              n624 = Compound Arithmetic op=AND(w1254, w1257, w1256) -> (w1255:bool)
              n625 = Compound Arithmetic op=AND(w1254, w1253, w1252) -> (w1251:bool)
              n626 = Boolean To (0,1)(Boolean=w1251) -> (0, 1=w1258:i16)
              n627 = Greater?(x=w1248, y=w1243) -> (0:w1249:bool)
              n628 = Greater?(x=w1245, y=w1243) -> (0:w1244:bool)
              n629 = Multiply(x=w1258, y=w1247) -> (x*y=w1259:dbl)
              n630 = Boolean To (0,1)(Boolean=w1255) -> (0, 1=w1261:i16)
              n631 = Multiply(x=w1261, y=w1250) -> (x*y=w1260:dbl)
              n632 = Bundle(w1259, "GUIdevice 8"=w1241) -> (w1272:cluster{dbl, "GUIdevice 8":string})  [unwired: 1 in]
              n633 = Bundle(w1260, "GUIdevice 8"=w1241) -> (w1273:cluster{dbl, "GUIdevice 8":string})  [unwired: 1 in]
            }
            "required X" <- w1169
            "required Y" <- w1168
            "speedmode X" <- w1145
            "speedmode Y" <- w1141
            n634 = case shown="True" "Align" {
              tunnel: w1167 -> [w1181 w1186]
              tunnel: w1166 -> [w1180 w1183]
              tunnel: [w1179 w1185] -> w1163
              tunnel: [w1178 w1182] -> w1157
              frame False {
                n635 = Sort 1D Array(array=w1180) -> (sorted array=w1177:cluster{dbl, "GUIdevice 8":string}[])
                n636 = Sort 1D Array(array=w1181) -> (sorted array=w1176:cluster{dbl, "GUIdevice 8":string}[])
                n637 = Reverse 1D Array(array=w1177) -> (reversed array=w1178:cluster{dbl, "GUIdevice 8":string}[])
                n638 = Reverse 1D Array(array=w1176) -> (reversed array=w1179:cluster{dbl, "GUIdevice 8":string}[])
              }
              frame True {
                w1184 = cluster{dbl, "GUIdevice 8":string}[] [] ("Array")
                n639 = for {
                  shift-right: [w1196] -> w1185
                  shift-left: w1184 -> [w1198]
                  tunnel: w1186 -> [w1197] mode=indexing
                  n640 = Unbundle(w1197) -> (w1200:dbl)  [unwired: 1 out]
                  n641 = Not Equal To 0?(x=w1200) -> (x != 0?=w1199:bool)
                  n642 = case shown="True" w1199 {
                    tunnel: w1198 -> [w1201 w1204]
                    tunnel: w1197 -> [_ w1203]
                    tunnel: [w1201 w1202] -> w1196
                    frame False {
                    }
                    frame True {
                      n643 = Build Array (concatenate)(w1204, w1203) -> (w1202:cluster{dbl, "GUIdevice 8":string}[])
                    }
                  }
                }
                n644 = for {
                  shift-right: [w1187] -> w1182
                  shift-left: w1184 -> [w1189]
                  tunnel: w1183 -> [w1188] mode=indexing
                  n645 = Unbundle(w1188) -> (w1191:dbl)  [unwired: 1 out]
                  n646 = Not Equal To 0?(x=w1191) -> (x != 0?=w1190:bool)
                  n647 = case shown="True" w1190 {
                    tunnel: w1189 -> [w1192 w1195]
                    tunnel: w1188 -> [_ w1194]
                    tunnel: [w1192 w1193] -> w1187
                    frame False {
                    }
                    frame True {
                      n648 = Build Array (concatenate)(w1195, w1194) -> (w1193:cluster{dbl, "GUIdevice 8":string}[])
                    }
                  }
                }
              }
            }
            n649 = call <vilib>:"Add State(s) to Queue__jki_lib_state_machine.vi"("State(s) in (\"\")"=w1150) -> ("States Out"=w1149:string)  [unwired: 14 in]
            n650 = Bundle By Name(cluster=w1144, "speedmode X"=w1145, "speedmode Y"=w1141) -> (w1143:T36)
            n651 = Empty Array?(array=w1163) -> (empty?=w1160:bool)
            n652 = Empty Array?(array=w1157) -> (empty?=w1155:bool)
            n653 = Index Array(array=w1163) -> (element=w1153:cluster{dbl, "GUIdevice 8":string})  [unwired: 1 in]
            n654 = Index Array(array=w1157) -> (element=w1152:cluster{dbl, "GUIdevice 8":string})  [unwired: 1 in]
            n655 = Unbundle(w1153) -> (w1162:dbl)  [unwired: 1 out]
            n656 = Unbundle(w1152) -> (w1158:dbl)  [unwired: 1 out]
            n657 = Equal To 0?(x=w1162) -> (x = 0?=w1161:bool)
            n658 = Equal To 0?(x=w1158) -> (x = 0?=w1156:bool)
            n659 = property on="autodetect" class="Bool (strict)"("Value"=FALSE ("autodetect")) -> ()  [unwired: 2 in, 2 out]
            n660 = Unbundle By Name(w1143) -> ("Feedback global"=w1164:bool)
            n661 = Or(x=w1161, y=w1160) -> (x .or. y?=w1159:bool)
            n662 = Or(x=w1156, y=w1155) -> (x .or. y?=w1154:bool)
            n663 = case shown="True" w1164 {
              tunnel: w1159 -> [_ w1212]
              tunnel: w1163 -> [_ w1211]
              tunnel: w1154 -> [_ w1209]
              tunnel: w1157 -> [_ w1208]
              tunnel: w1149 -> [w1205 w1207]
              tunnel: [w1205 w1206] -> w1165
              frame False {
              }
              frame True {
                n664 = case shown="False" w1212 {
                  tunnel: w1211 -> [w1227 _]
                  tunnel: w1207 -> [w1223 w1228]
                  tunnel: [w1221 w1228] -> w1210
                  frame False {
                    n665 = Index Array(array=w1227) -> (element=w1226:cluster{dbl, "GUIdevice 8":string})  [unwired: 1 in]
                    n666 = Unbundle By Name(w1226) -> ("GUIdevice 8"=w1225:string)
                    n667 = call <vilib>:"Build State String with Arguments__jki_lib_state_machine.vi"("Arguments (\"\")"=w1225, "State"="Move X") -> ("State with Arguments"=w1222:string)  [unwired: 4 in]
                    n668 = call <vilib>:"Add State(s) to Queue__jki_lib_state_machine.vi"("State(s) in (\"\")"=w1223, "State(s) at Back (\"\")"=w1222) -> ("States Out"=w1221:string)  [unwired: 13 in]
                  }
                  frame True {
                  }
                }
                n669 = case shown="False" w1209 {
                  tunnel: w1208 -> [w1219 _]
                  tunnel: w1210 -> [w1215 w1220]
                  tunnel: [w1213 w1220] -> w1206
                  frame False {
                    n670 = Index Array(array=w1219) -> (element=w1218:cluster{dbl, "GUIdevice 8":string})  [unwired: 1 in]
                    n671 = Unbundle By Name(w1218) -> ("GUIdevice 8"=w1217:string)
                    n672 = call <vilib>:"Build State String with Arguments__jki_lib_state_machine.vi"("Arguments (\"\")"=w1217, "State"="Move Y") -> ("State with Arguments"=w1214:string)  [unwired: 4 in]
                    n673 = call <vilib>:"Add State(s) to Queue__jki_lib_state_machine.vi"("State(s) in (\"\")"=w1215, "State(s) at Back (\"\")"=w1214) -> ("States Out"=w1213:string)  [unwired: 13 in]
                  }
                  frame True {
                  }
                }
              }
            }
            n674 = call <vilib>:"Add State(s) to Queue__jki_lib_state_machine.vi"("State(s) in (\"\")"=w1149, "State(s) at Back (\"\")"=w1165) -> ("States Out"=w1175:string)  [unwired: 13 in]
          }
          frame "Move X" {
            # "Your code here.\n(You can make a copy of, or modify, this frame)"
            n675 = Unbundle By Name(w1297) -> ("Offset X"=w1274:dbl[][])
            n676 = call-poly <userlib>:"Filter 1D Array__ogtk.vi"("items to filter"=w1282, "array"=w1301) -> ("filtered item indices"=w1286:i32[])  [unwired: 4 in, 1 out]
            n677 = Unbundle By Name(w1297) -> ("speedmode X"=w1281:bool[], "active axis refs 2"=w1300:T12, "move properties"=w1285:T2[])
            n678 = for {
              tunnel: w1286 -> [w1306] mode=indexing
              tunnel: w1285 -> [w1310]
              shift-right: [w1305] -> w1283
              shift-left: i32[] [] ("filtered item indices") -> [w1308]
              n679 = Index Array(array=w1310, index=w1306) -> (element=w1309:T2)
              n680 = Unbundle By Name(w1309) -> ("enable feedback"=w1307:bool)
              n681 = case shown="True" w1307 {
                tunnel: w1308 -> [w1311 w1314]
                tunnel: w1306 -> [_ w1313]
                tunnel: [w1311 w1312] -> w1305
                frame False {
                }
                frame True {
                  n682 = Build Array (concatenate)(w1314, w1313) -> (w1312:i32[])
                }
              }
            }
            n683 = Index Array(array=w1283) -> (element=w1280:i32)  [unwired: 1 in]
            n684 = Index Array(array=w1274, index (row)=w1280) -> (element=w1296:dbl[])  [unwired: 1 in]
            n685 = Reverse 1D Array(array=w1296) -> (reversed array=w1295:dbl[])
            n686 = Index Array(array=w1300, index=w1280) -> (element=w1299:cluster{"Ref X":refnum<vi>, "Ref Y":refnum<vi>})
            n687 = Index Array(array=w1295) -> (element=w1293:dbl)  [unwired: 1 in]
            n688 = Index Array(array=w1285, index=w1280) -> (element=w1298:T2)
            n689 = Unbundle By Name(w1299) -> ("Ref X"=w1290:refnum<vi>, "Ref Y"=w1289:refnum<vi>)
            n690 = Index Array(array=w1281, index=w1280) -> (element=w1279:bool)
            n691 = Unbundle By Name(w1298) -> ("Invert Direction X"=w1291:bool, "Invert Axis"=w1294:bool, "Stepsize"=w1277:dbl, "enable feedback"=w1288:bool)
            n692 = Greater Or Equal To 0?(x=w1293) -> (x >= 0?=w1292:bool)
            n693 = call <vilib>:"Add State(s) to Queue__jki_lib_state_machine.vi"("State(s) in Front (\"\")"="Wait" ("State(s) in Front (\"\")"), "State(s) in (\"\")"=w1304) -> ("States Out"=w1303:string)  [unwired: 13 in]
            n694 = property on="Speedmode @" class="DigNum (strict)"() -> ("Value"=w1276:dbl)  [unwired: 2 in, 2 out]
            n695 = Multiply(x=w1276, y=w1277) -> (x*y=w1278:dbl)
            n696 = Select(t=w1278, s=w1279, f=w1277) -> (s? t:f=w1275:dbl)
            n697 = case shown="True" w1288 {
              tunnel: w1294 -> [_ w1320]
              tunnel: w1292 -> [_ w1319]
              tunnel: w1275 -> [_ w1318]
              tunnel: w1291 -> [_ w1317]
              tunnel: w1290 -> [_ w1316]
              tunnel: w1289 -> [_ w1315]
              frame False {
              }
              frame True {
                n698 = case shown="False" w1319 {
                  tunnel: w1317 -> [w1328 w1350]
                  tunnel: w1318 -> [w1326 w1348]
                  tunnel: w1320 -> [w1325 w1347]
                  tunnel: w1320 -> [w1324 w1346]
                  tunnel: w1316 -> [w1322 w1344]
                  tunnel: w1315 -> [w1321 w1343]
                  frame True {
                    n699 = case shown="False" w1325 {
                      tunnel: [w1339 w1341] -> w1327
                      tunnel: w1322 -> [w1340 _]
                      tunnel: w1321 -> [_ w1342]
                      frame False {
                        n700 = property class="DigNum (strict)"(reference=w1340) -> ("Value"=w1339:dbl)  [unwired: 1 in, 2 out]
                      }
                      frame True {
                        n701 = property class="DigNum (strict)"(reference=w1342) -> ("Value"=w1341:dbl)  [unwired: 1 in, 2 out]
                      }
                    }
                    n702 = case shown="False" w1328 {
                      tunnel: w1327 -> [w1335 w1338]
                      tunnel: w1326 -> [w1334 w1337]
                      tunnel: [w1333 w1336] -> w1323
                      frame False {
                        n703 = Add(x=w1335, y=w1334) -> (x+y=w1333:dbl)
                      }
                      frame True {
                        n704 = Subtract(x=w1338, y=w1337) -> (x-y=w1336:dbl)
                      }
                    }
                    n705 = case shown="False" w1324 {
                      tunnel: w1323 -> [w1329 w1331]
                      tunnel: w1322 -> [w1330 _]
                      tunnel: w1321 -> [_ w1332]
                      frame False {
                        n706 = property class="DigNum (strict)"(reference=w1330, "Val(Sgnl)"=w1329) -> ()  [unwired: 1 in, 2 out]
                      }
                      frame True {
                        n707 = property class="DigNum (strict)"(reference=w1332, "Val(Sgnl)"=w1331) -> ()  [unwired: 1 in, 2 out]
                      }
                    }
                  }
                  frame False {
                    n708 = case shown="False" w1347 {
                      tunnel: [w1361 w1363] -> w1349
                      tunnel: w1344 -> [w1362 _]
                      tunnel: w1343 -> [_ w1364]
                      frame False {
                        n709 = property class="DigNum (strict)"(reference=w1362) -> ("Value"=w1361:dbl)  [unwired: 1 in, 2 out]
                      }
                      frame True {
                        n710 = property class="DigNum (strict)"(reference=w1364) -> ("Value"=w1363:dbl)  [unwired: 1 in, 2 out]
                      }
                    }
                    n711 = case shown="False" w1350 {
                      tunnel: w1349 -> [w1357 w1360]
                      tunnel: w1348 -> [w1356 w1359]
                      tunnel: [w1355 w1358] -> w1345
                      frame False {
                        n712 = Subtract(x=w1357, y=w1356) -> (x-y=w1355:dbl)
                      }
                      frame True {
                        n713 = Add(x=w1360, y=w1359) -> (x+y=w1358:dbl)
                      }
                    }
                    n714 = case shown="False" w1346 {
                      tunnel: w1345 -> [w1351 w1353]
                      tunnel: w1344 -> [w1352 _]
                      tunnel: w1343 -> [_ w1354]
                      frame False {
                        n715 = property class="DigNum (strict)"(reference=w1352, "Val(Sgnl)"=w1351) -> ()  [unwired: 1 in, 2 out]
                      }
                      frame True {
                        n716 = property class="DigNum (strict)"(reference=w1354, "Val(Sgnl)"=w1353) -> ()  [unwired: 1 in, 2 out]
                      }
                    }
                  }
                }
              }
            }
            "Arguments X" <- w1282
            "Moving X" <- w1282
          }
          frame "Move Y" {
            # "Your code here.\n(You can make a copy of, or modify, this frame)"
            n717 = Unbundle By Name(w1388) -> ("Offset Y"=w1387:dbl[][])
            n718 = call-poly <userlib>:"Filter 1D Array__ogtk.vi"("items to filter"=w1372, "array"=w1392) -> ("filtered item indices"=w1377:i32[])  [unwired: 4 in, 1 out]
            n719 = Unbundle By Name(w1388) -> ("speedmode Y"=w1371:bool[], "active axis refs 2"=w1391:T12, "move properties"=w1375:T2[])
            n720 = for {
              tunnel: w1377 -> [w1397] mode=indexing
              tunnel: w1375 -> [w1401]
              shift-right: [w1396] -> w1376
              shift-left: i32[] [] ("filtered item indices") -> [w1399]
              n721 = Index Array(array=w1401, index=w1397) -> (element=w1400:T2)
              n722 = Unbundle By Name(w1400) -> ("enable feedback"=w1398:bool)
              n723 = case shown="True" w1398 {
                tunnel: w1399 -> [w1402 w1405]
                tunnel: w1397 -> [_ w1404]
                tunnel: [w1402 w1403] -> w1396
                frame False {
                }
                frame True {
                  n724 = Build Array (concatenate)(w1405, w1404) -> (w1403:i32[])
                }
              }
            }
            n725 = Index Array(array=w1376) -> (element=w1370:i32)  [unwired: 1 in]
            n726 = Index Array(array=w1387, index (row)=w1370) -> (element=w1386:dbl[])  [unwired: 1 in]
            n727 = Reverse 1D Array(array=w1386) -> (reversed array=w1385:dbl[])
            n728 = Index Array(array=w1391, index=w1370) -> (element=w1390:cluster{"Ref X":refnum<vi>, "Ref Y":refnum<vi>})
            n729 = Index Array(array=w1385) -> (element=w1383:dbl)  [unwired: 1 in]
            n730 = Index Array(array=w1375, index=w1370) -> (element=w1389:T2)
            n731 = Index Array(array=w1371, index=w1370) -> (element=w1369:bool)
            n732 = Unbundle By Name(w1390) -> ("Ref Y"=w1380:refnum<vi>, "Ref X"=w1379:refnum<vi>)
            n733 = Unbundle By Name(w1389) -> ("Invert Direction Y"=w1381:bool, "Invert Axis"=w1384:bool, "Stepsize"=w1367:dbl, "enable feedback"=w1378:bool)
            n734 = Greater Or Equal To 0?(x=w1383) -> (x >= 0?=w1382:bool)
            n735 = call <vilib>:"Add State(s) to Queue__jki_lib_state_machine.vi"("State(s) in Front (\"\")"="Wait" ("State(s) in Front (\"\")"), "State(s) in (\"\")"=w1395) -> ("States Out"=w1394:string)  [unwired: 13 in]
            n736 = property on="Speedmode @" class="DigNum (strict)"() -> ("Value"=w1366:dbl)  [unwired: 2 in, 2 out]
            n737 = Multiply(x=w1366, y=w1367) -> (x*y=w1365:dbl)
            n738 = Select(t=w1365, s=w1369, f=w1367) -> (s? t:f=w1368:dbl)
            n739 = case shown="True" w1378 {
              tunnel: w1384 -> [_ w1411]
              tunnel: w1382 -> [_ w1410]
              tunnel: w1368 -> [_ w1409]
              tunnel: w1381 -> [_ w1408]
              tunnel: w1380 -> [_ w1407]
              tunnel: w1379 -> [_ w1406]
              frame False {
              }
              frame True {
                n740 = case shown="True" w1410 {
                  tunnel: w1408 -> [w1419 w1441]
                  tunnel: w1409 -> [w1417 w1439]
                  tunnel: w1411 -> [w1416 w1438]
                  tunnel: w1411 -> [w1415 w1437]
                  tunnel: w1407 -> [w1413 w1435]
                  tunnel: w1406 -> [w1412 w1434]
                  frame True {
                    n741 = case shown="False" w1416 {
                      tunnel: [w1430 w1432] -> w1418
                      tunnel: w1413 -> [w1431 _]
                      tunnel: w1412 -> [_ w1433]
                      frame False {
                        n742 = property class="DigNum (strict)"(reference=w1431) -> ("Value"=w1430:dbl)  [unwired: 1 in, 2 out]
                      }
                      frame True {
                        n743 = property class="DigNum (strict)"(reference=w1433) -> ("Value"=w1432:dbl)  [unwired: 1 in, 2 out]
                      }
                    }
                    n744 = case shown="False" w1419 {
                      tunnel: w1418 -> [w1426 w1429]
                      tunnel: w1417 -> [w1425 w1428]
                      tunnel: [w1424 w1427] -> w1414
                      frame False {
                        n745 = Add(x=w1426, y=w1425) -> (x+y=w1424:dbl)
                      }
                      frame True {
                        n746 = Subtract(x=w1429, y=w1428) -> (x-y=w1427:dbl)
                      }
                    }
                    n747 = case shown="False" w1415 {
                      tunnel: w1414 -> [w1420 w1422]
                      tunnel: w1413 -> [w1421 _]
                      tunnel: w1412 -> [_ w1423]
                      frame False {
                        n748 = property class="DigNum (strict)"(reference=w1421, "Val(Sgnl)"=w1420) -> ()  [unwired: 1 in, 2 out]
                      }
                      frame True {
                        n749 = property class="DigNum (strict)"(reference=w1423, "Val(Sgnl)"=w1422) -> ()  [unwired: 1 in, 2 out]
                      }
                    }
                  }
                  frame False {
                    n750 = case shown="False" w1438 {
                      tunnel: [w1452 w1454] -> w1440
                      tunnel: w1435 -> [w1453 _]
                      tunnel: w1434 -> [_ w1455]
                      frame False {
                        n751 = property class="DigNum (strict)"(reference=w1453) -> ("Value"=w1452:dbl)  [unwired: 1 in, 2 out]
                      }
                      frame True {
                        n752 = property class="DigNum (strict)"(reference=w1455) -> ("Value"=w1454:dbl)  [unwired: 1 in, 2 out]
                      }
                    }
                    n753 = case shown="False" w1441 {
                      tunnel: w1440 -> [w1448 w1451]
                      tunnel: w1439 -> [w1447 w1450]
                      tunnel: [w1446 w1449] -> w1436
                      frame False {
                        n754 = Subtract(x=w1448, y=w1447) -> (x-y=w1446:dbl)
                      }
                      frame True {
                        n755 = Add(x=w1451, y=w1450) -> (x+y=w1449:dbl)
                      }
                    }
                    n756 = case shown="False" w1437 {
                      tunnel: w1436 -> [w1442 w1444]
                      tunnel: w1435 -> [w1443 _]
                      tunnel: w1434 -> [_ w1445]
                      frame False {
                        n757 = property class="DigNum (strict)"(reference=w1443, "Val(Sgnl)"=w1442) -> ()  [unwired: 1 in, 2 out]
                      }
                      frame True {
                        n758 = property class="DigNum (strict)"(reference=w1445, "Val(Sgnl)"=w1444) -> ()  [unwired: 1 in, 2 out]
                      }
                    }
                  }
                }
              }
            }
            "Arguments Y" <- w1372
            "Moving Y" <- w1372
          }
          frame "Wait" {
            # "Your code here.\n(You can make a copy of, or modify, this frame)"
            n759 = flat-sequence {
              frame #0 {
                n760 = Wait (ms)(milliseconds to wait=u32 300) -> ()  [unwired: 1 out]
              }
              frame #1 {
                n761 = property on="Moving Y" class="Str"("Value"="") -> ()  [unwired: 2 in, 2 out]
                n762 = property on="Moving X" class="Str"("Value"="") -> ()  [unwired: 2 in, 2 out]
              }
            }
            n763 = call <vilib>:"Add State(s) to Queue__jki_lib_state_machine.vi"("State(s) in (\"\")"=w1461) -> ("States Out"=w1460:string)  [unwired: 14 in]
            n764 = local read "Mean Centroid X"() -> (w1456:dbl[][])
            n765 = Bundle By Name(cluster=w1458, "Mean Centroid X"=w1456, "Mean Centroid Y"=w1456) -> (w1457:T36)
          }
          frame "stats" {
            # "Your code here.\n(You can make a copy of, or modify, this frame)"
            n766 = Unbundle By Name(w1470) -> ("Offset X"=w1469:dbl[][], "Offset Y"=w1468:dbl[][], "Time"=w1467:timestamp[][], "Motor X"=w1466:dbl[][], "Motor Y"=w1465:dbl[][])
            n767 = for {
              tunnel: w1468 -> [w1508]
              tunnel: w1467 -> [w1509]
              tunnel: w1469 -> [w1510]
              tunnel: [w1513] -> w1496 mode=indexing
              tunnel: w1466 -> [w1507]
              tunnel: w1465 -> [w1506]
              tunnel: w1471 -> [_] mode=indexing
              i -> [w1500]
              n768 = Index Array(array=w1508, index (row)=w1500) -> (element=w1504:dbl[])  [unwired: 1 in]
              n769 = Index Array(array=w1507, index (row)=w1500) -> (element=w1502:dbl[])  [unwired: 1 in]
              n770 = Index Array(array=w1506, index (row)=w1500) -> (element=w1501:dbl[])  [unwired: 1 in]
              n771 = Index Array(array=w1510, index (row)=w1500) -> (element=w1505:dbl[])  [unwired: 1 in]
              n772 = Index Array(array=w1509, index (row)=w1500) -> (element=w1503:timestamp[])  [unwired: 1 in]
              n773 = Bundle("Time"=w1503, "Motor X"=w1502) -> (w1512:cluster{"Time":timestamp[], "Motor X":dbl[]})  [unwired: 1 in]
              n774 = Bundle("Time"=w1503, "Motor Y"=w1501) -> (w1511:cluster{"Time":timestamp[], "Motor Y":dbl[]})  [unwired: 1 in]
              n775 = Bundle("Time"=w1503, "Offset X"=w1505) -> (w1514:cluster{"Time":timestamp[], "Offset X":dbl[]})  [unwired: 1 in]
              n776 = Bundle("Time"=w1503, "Offset Y"=w1504) -> (w1515:cluster{"Time":timestamp[], "Offset Y":dbl[]})  [unwired: 1 in]
              n777 = Build Array(w1515, w1514, w1512, w1511) -> (w1513:cluster{"Time":timestamp[], "Motor Y":dbl[]}[])
            }
            n778 = call <vilib>:"Add State(s) to Queue__jki_lib_state_machine.vi"("State(s) in (\"\")"=w1499) -> ("States Out"=w1498:string)  [unwired: 14 in]
            n779 = Index Array(array=w1496, index (row) #1=0 ("index (row)"), index (row) #2=1 ("index (row)"), index (row) #3=2 ("index (row)"), index (row) #4=3 ("index (row)"), index (row) #5=4 ("index (row)"), index (row) #6=5 ("index (row)"), index (row) #7=6 ("index (row)"), index (row) #8=7 ("index (row)"), index (row) #9=8 ("index (row)"), index (row) #10=9 ("index (row)"), index (row) #11=10 ("index (row)"), index (row) #12=11 ("index (row)")) -> (element #1=→"CCD 1":cluster{"Time":timestamp[], "Motor Y":dbl[]}[], element #2=→"CCD 2":cluster{"Time":timestamp[], "Motor Y":dbl[]}[], element #3=→"CCD 3":cluster{"Time":timestamp[], "Motor Y":dbl[]}[], element #4=→"CCD 4":cluster{"Time":timestamp[], "Motor Y":dbl[]}[], element #5=→"CCD 5":cluster{"Time":timestamp[], "Motor Y":dbl[]}[], element #6=→"CCD 6":cluster{"Time":timestamp[], "Motor Y":dbl[]}[], element #7=→"CCD 7":cluster{"Time":timestamp[], "Motor Y":dbl[]}[], element #8=→"CCD 8":cluster{"Time":timestamp[], "Motor Y":dbl[]}[], element #9=→"CCD 9":cluster{"Time":timestamp[], "Motor Y":dbl[]}[], element #10=→"CCD 10":cluster{"Time":timestamp[], "Motor Y":dbl[]}[], element #11=→"CCD 11":cluster{"Time":timestamp[], "Motor Y":dbl[]}[], element #12=→"CCD 12":cluster{"Time":timestamp[], "Motor Y":dbl[]}[])  [unwired: 12 in]
          }
          frame "---------------Statistics--------------" {
            # "Template Separator\n(You can make a copy of, or modify, this frame)"
            n780 = call <vilib>:"Add State(s) to Queue__jki_lib_state_machine.vi"("State(s) in (\"\")"=w1519) -> ("States Out"=w1518:string)  [unwired: 14 in]
          }
          frame "Save Stats" {
            # "Your code here.\n(You can make a copy of, or modify, this frame)"
            n781 = property on="CCD 1" class="XYGraph (strict)"() -> ("Value"=w1529:cluster{timestamp[], dbl[]}[])  [unwired: 2 in, 2 out]
            n782 = property on="CCD 2" class="XYGraph (strict)"() -> ("Value"=w1528:cluster{timestamp[], dbl[]}[])  [unwired: 2 in, 2 out]
            n783 = property on="CCD 3" class="XYGraph (strict)"() -> ("Value"=w1527:cluster{timestamp[], dbl[]}[])  [unwired: 2 in, 2 out]
            n784 = property on="CCD 4" class="XYGraph (strict)"() -> ("Value"=w1526:cluster{timestamp[], dbl[]}[])  [unwired: 2 in, 2 out]
            n785 = property on="CCD 5" class="XYGraph (strict)"() -> ("Value"=w1525:cluster{timestamp[], dbl[]}[])  [unwired: 2 in, 2 out]
            n786 = property on="CCD 6" class="XYGraph (strict)"() -> ("Value"=w1524:cluster{timestamp[], dbl[]}[])  [unwired: 2 in, 2 out]
            n787 = property on="CCD 7" class="XYGraph (strict)"() -> ("Value"=w1523:cluster{timestamp[], dbl[]}[])  [unwired: 2 in, 2 out]
            n788 = property on="CCD 8" class="XYGraph (strict)"() -> ("Value"=w1522:cluster{timestamp[], dbl[]}[])  [unwired: 2 in, 2 out]
            n789 = Build Array(w1529, w1528, w1527, w1526, w1525, w1524, w1523, w1522) -> (w1521:cluster{timestamp[], dbl[]}[][])
            n790 = for {
              tunnel: w1521 -> [w1537] mode=indexing
              tunnel: w1520 -> [w1536] mode=indexing
              n791 = Empty String/Path?(string/path=w1536) -> (empty?=w1535:bool)
              n792 = case shown="False" w1535 {
                tunnel: w1537 -> [w1543 _]
                tunnel: w1536 -> [w1541 _]
                frame False {
                  n793 = Index Array(array=w1543, index #1=0 ("index"), index #2=1 ("index"), index #3=2 ("index"), index #4=3 ("index")) -> (element #1=w1578:cluster{timestamp[], dbl[]}, element #2=w1572:cluster{timestamp[], dbl[]}, element #3=w1571:cluster{timestamp[], dbl[]}, element #4=w1570:cluster{timestamp[], dbl[]})  [unwired: 1 in, 1 out]
                  n794 = Concatenate Strings(w1541, ".dat" ("string")) -> (w1539:string)
                  n795 = Unbundle(w1578) -> (w1577:timestamp[], w1555:dbl[])
                  n796 = Unbundle(w1572) -> (w1546:dbl[])  [unwired: 1 out]
                  n797 = Unbundle(w1571) -> (w1545:dbl[])  [unwired: 1 out]
                  n798 = Unbundle(w1570) -> (w1544:dbl[])  [unwired: 1 out]
                  n799 = Build Path(base path="save path", name or relative path=w1539) -> (appended path=w1538:path)
                  n800 = for {
                    tunnel: w1577 -> [w1580] mode=indexing
                    tunnel: [w1579] -> w1553 mode=indexing
                    n801 = Format Date/Time String(time format string (%c)="%Y%m%d%H%M%S", seconds (now)=w1580) -> (date/time string=w1579:string)  [unwired: 1 in]
                  }
                  n802 = Array Size(array=w1555) -> (size(s)=w1556:i32)
                  n803 = Number To Fractional String(number=w1555) -> (F-format string=w1552:string[])  [unwired: 3 in]
                  n804 = Number To Fractional String(number=w1546) -> (F-format string=w1549:string[])  [unwired: 3 in]
                  n805 = Number To Fractional String(number=w1545) -> (F-format string=w1548:string[])  [unwired: 3 in]
                  n806 = Number To Fractional String(number=w1544) -> (F-format string=w1547:string[])  [unwired: 3 in]
                  n807 = Initialize Array("", w1556, 5 ("dimension size")) -> (w1554:string[][])
                  n808 = Insert Into Array(array=w1554, index (col)=0 ("disabled index (col)"), new element=w1553) -> (w1564:string[][])  [unwired: 1 in]
                  n809 = Insert Into Array(array=w1564, index (col)=1 ("disabled index (col)"), new element=w1552) -> (w1563:string[][])  [unwired: 1 in]
                  n810 = Insert Into Array(array=w1563, index (col)=2 ("disabled index (col)"), new element=w1549) -> (w1567:string[][])  [unwired: 1 in]
                  n811 = Insert Into Array(array=w1567, index (col)=3 ("disabled index (col)"), new element=w1548) -> (w1568:string[][])  [unwired: 1 in]
                  n812 = Insert Into Array(array=w1568, index (col)=4 ("disabled index (col)"), new element=w1547) -> (w1569:string[][])  [unwired: 1 in]
                  n813 = Insert Into Array(array=w1569, index (row)=0, new element=string[] ["time", "Centroid X", "Centroid Y", "Motor Axis 1", "Motor Axis 2"] ("new element/subarray 2")) -> (w1551:string[][])  [unwired: 1 in]
                  n814 = call-poly <vilib>:"Write To Spreadsheet File.vi"("2D data"=w1551, "file path (dialog if empty)"=w1538) -> ()  [unwired: 6 in, 1 out]
                }
                frame True {
                }
              }
            }
            n815 = call <vilib>:"Add State(s) to Queue__jki_lib_state_machine.vi"("State(s) in (\"\")"=w1534) -> ("States Out"=w1533:string)  [unwired: 14 in]
            n816 = property on="Save Stats" class="Bool (strict)"("Value"=FALSE ("Save Stats")) -> ()  [unwired: 2 in, 2 out]
          }
          frame "tdms" {
            w1607 = 21600.0 ("new tdms")
            # "Your code here.\n(You can make a copy of, or modify, this frame)"
            n817 = Unbundle By Name(w1597) -> ("Data Value Reference out"=w1620:refnum<k34>, "Offset X"=w1622:dbl[][], "Offset Y"=w1617:dbl[][], "active axis refs 2"=w1619:T12)
            n818 = for {
              tunnel: w1622 -> [w1666]
              tunnel: w1617 -> [w1665]
              tunnel: w1621 -> [w1629] mode=indexing
              tunnel: w1620 -> [w1630]
              tunnel: w1619 -> [w1651]
              tunnel: w1618 -> [w1635]
              tunnel: [w1633] -> w1616
              i -> [w1652]
              n819 = Index Array(array=w1666, index (row)=w1652) -> (element=w1664:dbl[])  [unwired: 1 in]
              n820 = Index Array(array=w1665, index (row)=w1652) -> (element=w1663:dbl[])  [unwired: 1 in]
              n821 = Index Array(array=w1651, index=w1652) -> (element=w1650:cluster{"Ref X":refnum<vi>, "Ref Y":refnum<vi>})
              n822 = Reverse 1D Array(array=w1663) -> (reversed array=w1661:dbl[])
              n823 = Reverse 1D Array(array=w1664) -> (reversed array=w1662:dbl[])
              n824 = Unbundle By Name(w1650) -> ("Ref X"=w1649:refnum<vi>, "Ref Y"=w1648:refnum<vi>)
              n825 = Index Array(array=w1662) -> (element=w1660:dbl)  [unwired: 1 in]
              n826 = Index Array(array=w1661) -> (element=w1659:dbl)  [unwired: 1 in]
              n827 = property class="DigNum (strict)"(reference=w1649, error in=w1635) -> (error out=w1634:errorcluster, "Value"=w1643:dbl)  [unwired: 1 out]
              n828 = Build Array(w1660) -> (w1632:dbl[])
              n829 = Build Array(w1659) -> (w1654:dbl[])
              n830 = Get Date/Time In Seconds() -> (seconds since 1Jan1904=w1631:timestamp)
              n831 = Build Array(w1631) -> (w1627:timestamp[])
              n832 = property class="DigNum (strict)"(reference=w1648, error in=w1634) -> (error out=w1625:errorcluster, "Value"=w1637:dbl)  [unwired: 1 out]
              n833 = Build Array(w1643) -> (w1642:dbl[])
              n834 = TDMS Write(0:w1630, 5:w1629, 7:"time", 9:w1627, 11:w1625) -> (4:w1626:refnum<k34>, 15:w1624:errorcluster)  [unwired: 1 in, 2 out]
              n835 = Build Array(w1637) -> (w1636:dbl[])
              n836 = TDMS Write(0:w1626, 5:w1629, 7:"centroid X", 9:w1632, 11:w1624) -> (4:w1657:refnum<k34>, 6:w1656:string, 15:w1655:errorcluster)  [unwired: 1 in, 1 out]
              n837 = TDMS Write(0:w1657, 5:w1656, 7:"centroid Y", 9:w1654, 11:w1655) -> (4:w1646:refnum<k34>, 6:w1645:string, 15:w1647:errorcluster)  [unwired: 1 in, 1 out]
              n838 = TDMS Write(0:w1646, 5:w1645, 7:"Motor Axis 1", 9:w1642, 11:w1647) -> (4:w1641:refnum<k34>, 6:w1640:string, 15:w1638:errorcluster)  [unwired: 1 in, 1 out]
              n839 = TDMS Write(0:w1641, 5:w1640, 7:"Motor Axis 2", 9:w1636, 11:w1638) -> (15:w1633:errorcluster)  [unwired: 1 in, 3 out]
            }
            n840 = Unbundle By Name(w1597) -> ("img to avg"=w1595:i32)
            n841 = property on="millisecond timer value" class="DigNum (strict)"() -> ("Value"=w1584:u32)  [unwired: 2 in, 2 out]
            n842 = local read "millisecond timer 2"() -> (w1613:u32)
            n843 = Tick Count (ms)() -> (millisecond timer value=w1598:u32)
            n844 = call <userlib>:"Tick Count (ms)__ogtk.vi"("error in (no error)"=w1616) -> ("error out"=w1583:errorcluster, "millisecond timer value"=w1615:u32)  [unwired: 9 in]
            n845 = Subtract(x=w1598, y=w1584) -> (x-y=w1612:u32)
            n846 = Subtract(x=w1598, y=w1584) -> (x-y=w1599:u32)
            n847 = Subtract(x=w1615, y=w1613) -> (x-y=→"Waveform Chart":u32)
            n848 = Multiply(x=5.0 ("new tdms"), y=w1595) -> (x*y=w1593:dbl)
            n849 = Divide(x=w1612, y=u32 1000) -> (x/y=w1610:dbl)
            n850 = Divide(x=w1599, y=u32 1000) -> (x/y=w1601:dbl)
            n851 = Quotient & Remainder(x=w1610, y=w1607) -> (x-y*floor(x/y)=w1609:dbl)  [unwired: 1 out]
            n852 = Quotient & Remainder(x=w1601, y=w1593) -> (x-y*floor(x/y)=w1594:dbl)  [unwired: 1 out]
            "x-y*floor(x/y)" <- w1594
            n853 = Subtract(x=w1593, y=2.0) -> (x-y=w1591:dbl)
            n854 = Greater?(x=w1594, y=w1591) -> (0:w1590:bool)
            n855 = call <vilib>:"Clear Errors.vi"("error in (no error)"=w1583) -> ("error out"=w1582:errorcluster)  [unwired: 6 in]
            n856 = Subtract(x=w1607, y=20.0) -> (x-y=w1605:dbl)
            n857 = Greater?(x=w1609, y=w1605) -> (0:w1608:bool)
            n858 = Select(t="Device Ini", s=w1590, f="") -> (s? t:f=w1587:string)
            n859 = Select(t="newtdms", s=w1608, f="") -> (s? t:f=w1602:string)
            n860 = call <vilib>:"Add State(s) to Queue__jki_lib_state_machine.vi"("State(s) in (\"\")"=w1623, "State(s) at Back (\"\")"=w1602) -> ("States Out"=w1586:string)  [unwired: 13 in]
            n861 = call <vilib>:"Add State(s) to Queue__jki_lib_state_machine.vi"("State(s) in Front (\"\")"=w1587, "State(s) in (\"\")"=w1586) -> ("States Out"=w1585:string)  [unwired: 13 in]
          }
          frame "Reset History" {
            # "Your code here.\n(You can make a copy of, or modify, this frame)"
            n862 = for {
              N: 1 -> [_]
              shift-right: [w1676] -> w1668
              shift-left: timestamp[][] [] ("Time") -> [w1678]
              n863 = for {
                N: 12 -> [_]
                tunnel: w1678 -> [w1681] mode=indexing
                tunnel: [w1679] -> w1676 mode=indexing
                n864 = Get Date/Time In Seconds() -> (seconds since 1Jan1904=w1680:timestamp)
                n865 = Build Array (concatenate)(w1681, w1680) -> (w1679:timestamp[])
              }
            }
            n866 = local read "Offset X"() -> (w1667:dbl[][])
            n867 = Bundle By Name(cluster=w1672, "Offset X"=w1667, "Offset Y"=w1667, "Time"=w1668, "Motor X"=w1667) -> (w1671:T36)
            n868 = call <vilib>:"Add State(s) to Queue__jki_lib_state_machine.vi"("State(s) in (\"\")"=w1675) -> ("States Out"=w1674:string)  [unwired: 14 in]
          }
          frame "New Category: 2" {
            # "Your code here.\n(You can make a copy of, or modify, this frame)"
            n869 = call <vilib>:"Add State(s) to Queue__jki_lib_state_machine.vi"("State(s) in (\"\")"=w1685) -> ("States Out"=w1684:string)  [unwired: 14 in]
          }
          frame "ImgToAvg" {
            # "Your code here.\n(You can make a copy of, or modify, this frame)"
            n870 = Decimal String To Number(string=w1689) -> (number=w1686:i32)  [unwired: 2 in, 1 out]
            n871 = Bundle By Name(cluster=w1688, "img to avg"=w1686) -> (w1687:T36)
            n872 = call <vilib>:"Add State(s) to Queue__jki_lib_state_machine.vi"("State(s) in (\"\")"=w1692) -> ("States Out"=w1691:string)  [unwired: 14 in]
          }
          frame "newtdms" {
            # "Your code here.\n(You can make a copy of, or modify, this frame)"
            n873 = Unbundle By Name(w1713) -> ("Data Value Reference out"=w1712:refnum<k34>, "active cams"=w1707:string[])
            n874 = TDMS Close(8:w1711, 11:w1712) -> (0:w1694:errorcluster)  [unwired: 1 out]
            n875 = Get Date/Time In Seconds() -> (seconds since 1Jan1904=w1705:timestamp)
            n876 = Format Date/Time String(time format string (%c)="%Y%m%d", seconds (now)=w1705) -> (date/time string=w1703:string)  [unwired: 1 in]
            n877 = Format Date/Time String(time format string (%c)="%Y%m%d%H%M", seconds (now)=w1705) -> (date/time string=w1715:string)  [unwired: 1 in]
            n878 = call <vilib>:"Clear Errors.vi"("error in (no error)"=w1694) -> ("error out"=w1693:errorcluster)  [unwired: 6 in]
            n879 = Build Path(base path=w1704, name or relative path=w1703) -> (appended path=w1702:path)
            n880 = Concatenate Strings(w1715, "Beampointing_Pico.tdms" ("string")) -> (w1721:string)
            n881 = String To Path(string=w1721) -> (path=w1722:path)
            n882 = call <vilib>:"Check if File or Folder Exists.vi"("error in (no error)"=w1693, "path"=w1702) -> ("error out"=w1698:errorcluster, "file or folder exists?"=w1701:bool, "dup path"=w1700:path)  [unwired: 7 in]
            n883 = case shown="False" w1701 {
              tunnel: w1700 -> [w1729 w1731]
              tunnel: [w1728 w1731] -> w1699
              tunnel: w1698 -> [w1727 w1730]
              tunnel: [w1726 w1730] -> w1697
              frame False {
                n884 = Create Folder(path (use dialog)=w1729, error in=w1727) -> (created path=w1728:path, error out=w1726:errorcluster)  [unwired: 1 in, 1 out]
              }
              frame True {
              }
            }
            n885 = call <vilib>:"Add State(s) to Queue__jki_lib_state_machine.vi"("State(s) in (\"\")"=w1725) -> ("States Out"=w1724:string)  [unwired: 14 in]
            n886 = Build Path(base path=w1699, name or relative path=w1722) -> (appended path=w1716:path)
            n887 = TDMS Open(6:FALSE ("disable buffering (T)"), 7:enum16{"1.0", "2.0"}."2.0" ("file format version (2.0)"), 8:w1697, 10:T17."create or replace" ("operation"), 11:w1716) -> (0:w1708:errorcluster, 3:w1710:refnum<k34>)  [unwired: 2 in]
            n888 = call "TDMSbuffersize.vi"("error in (no error)"=w1708, "group names"=w1707, "Data Value Reference in"=w1710) -> ("error out"=w1696:errorcluster, "Data Value Reference out"=w1709:refnum<k34>)  [unwired: 7 in]
            n889 = Bundle By Name(cluster=w1713, "Data Value Reference out"=w1709) -> (w1714:T36)
            n890 = call <vilib>:"Clear Errors.vi"("error in (no error)"=w1696) -> ("error out"=w1695:errorcluster)  [unwired: 6 in]
          }
          frame "Center" {
            # "Your code here.\n(You can make a copy of, or modify, this frame)"
            n891 = property on="Center" class="Bool (strict)"("Value"=FALSE ("Center")) -> ()  [unwired: 2 in, 2 out]
            n892 = control-ref of="image::1"() -> (w1746:refnum<vi>)
            n893 = control-ref of="image::2"() -> (w1745:refnum<vi>)
            n894 = control-ref of="image::3"() -> (w1744:refnum<vi>)
            n895 = control-ref of="image::4"() -> (w1743:refnum<vi>)
            n896 = control-ref of="image::5"() -> (w1742:refnum<vi>)
            n897 = control-ref of="image::6"() -> (w1741:refnum<vi>)
            n898 = control-ref of="image::7"() -> (w1740:refnum<vi>)
            n899 = control-ref of="image::8"() -> (w1739:refnum<vi>)
            n900 = control-ref of="image::9"() -> (w1738:refnum<vi>)
            n901 = control-ref of="image::10"() -> (w1737:refnum<vi>)
            n902 = control-ref of="image::11"() -> (w1736:refnum<vi>)
            n903 = control-ref of="image::12"() -> (w1735:refnum<vi>)
            n904 = for {
              tunnel: w1732 -> [w1759] mode=indexing
              tunnel: [w1754] -> w1747 mode=indexing
              n905 = Unbundle By Name(w1759) -> ("Target.X::12"=w1758:refnum<vi>, "Target.Y::12"=w1757:refnum<vi>)
              n906 = property class="DigNum (strict)"(reference=w1758) -> ("Value"=w1756:dbl)  [unwired: 1 in, 2 out]
              n907 = property class="DigNum (strict)"(reference=w1757) -> ("Value"=w1755:dbl)  [unwired: 1 in, 2 out]
              n908 = Bundle("Value"=w1756, "Value"=w1755) -> (w1754:cluster{"Value":dbl, "Value":dbl})  [unwired: 1 in]
            }
            n909 = call <vilib>:"Add State(s) to Queue__jki_lib_state_machine.vi"("State(s) in (\"\")"=w1751) -> ("States Out"=w1750:string)  [unwired: 14 in]
            n910 = Build Array(w1746, w1745, w1744, w1743, w1742, w1741, w1740, w1739, w1738, w1737, w1736, w1735) -> (w1734:refnum<vi>[])
            n911 = for {
              tunnel: w1734 -> [w1753] mode=indexing
              tunnel: w1747 -> [w1752] mode=indexing
              n912 = property class="ImageControl"(reference=w1753, "Image Center Position"=w1752) -> ()  [unwired: 1 in, 2 out]
            }
          }
          frame "history" {
            # "Your code here.\n(You can make a copy of, or modify, this frame)"
            n913 = Unbundle By Name(w1769) -> ("Offset X"=w1775:dbl[][], "Offset Y"=w1774:dbl[][], "Mean Centroid X"=w1773:dbl[][], "Mean Centroid Y"=w1772:dbl[][], "Motor X"=w1771:dbl[][], "Motor Y"=w1770:dbl[][], "Time"=w1761:timestamp[][])
            n914 = for {
              tunnel: w1775 -> [w1793] mode=indexing
              tunnel: w1774 -> [w1791] mode=indexing
              tunnel: w1773 -> [w1790] mode=indexing
              tunnel: w1772 -> [w1789] mode=indexing
              tunnel: w1771 -> [w1788] mode=indexing
              tunnel: w1770 -> [w1787] mode=indexing
              tunnel: [w1792] -> w1767 mode=indexing
              tunnel: [w1786] -> w1766 mode=indexing
              tunnel: [w1782] -> w1765 mode=indexing
              tunnel: [w1785] -> w1764 mode=indexing
              tunnel: [w1784] -> w1763 mode=indexing
              tunnel: [w1783] -> w1762 mode=indexing
              tunnel: w1761 -> [w1781] mode=indexing
              tunnel: [w1779] -> w1760 mode=indexing
              w1780 = 0
              n915 = Delete From Array(array=w1788, index=w1780) -> (array with subset deleted=w1784:dbl[])  [unwired: 1 in, 1 out]
              n916 = Delete From Array(array=w1787, index=w1780) -> (array with subset deleted=w1783:dbl[])  [unwired: 1 in, 1 out]
              n917 = Delete From Array(array=w1781, index=w1780) -> (array with subset deleted=w1779:timestamp[])  [unwired: 1 in, 1 out]
              n918 = Delete From Array(array=w1790, index=w1780) -> (array with subset deleted=w1782:dbl[])  [unwired: 1 in, 1 out]
              n919 = Delete From Array(array=w1789, index=w1780) -> (array with subset deleted=w1785:dbl[])  [unwired: 1 in, 1 out]
              n920 = Delete From Array(array=w1791, index=w1780) -> (array with subset deleted=w1786:dbl[])  [unwired: 1 in, 1 out]
              n921 = Delete From Array(array=w1793, index=w1780) -> (array with subset deleted=w1792:dbl[])  [unwired: 1 in, 1 out]
            }
            n922 = call <vilib>:"Add State(s) to Queue__jki_lib_state_machine.vi"("State(s) in (\"\")"=w1778) -> ("States Out"=w1777:string)  [unwired: 14 in]
            n923 = Bundle By Name(cluster=w1769, "Offset X"=w1767, "Offset Y"=w1766, "Mean Centroid X"=w1765, "Mean Centroid Y"=w1764, "Motor X"=w1763, "Motor Y"=w1762, "Time"=w1760) -> (w1768:T36)
          }
        }
        n924 = property on="Box" class="Arr (strict)"() -> ("Value"=w266:T6)  [unwired: 2 in, 2 out]
        n925 = for {
          tunnel: w268 -> [w296]
          tunnel: w267 -> [w297]
          tunnel: w259 -> [w289] mode=indexing
          tunnel: w266 -> [w290] mode=indexing
          n926 = call-poly <userlib>:"Filter 1D Array__ogtk.vi"("items to filter"=w289, "array"=w297) -> ("filtered item indices"=w298:i32[])  [unwired: 4 in, 1 out]
          n927 = Index Array(array=w298) -> (element=w292:i32)  [unwired: 1 in]
          n928 = Index Array(array=w296, index=w292) -> (element=w295:T30)
          n929 = Unbundle By Name(w295) -> ("Target.X::12"=w300:refnum<vi>, "Target.Y::12"=w299:refnum<vi>)
          n930 = property class="DigNum (strict)"(reference=w300) -> ("Value"=w294:dbl)  [unwired: 1 in, 2 out]
          n931 = property class="DigNum (strict)"(reference=w299) -> ("Value"=w293:dbl)  [unwired: 1 in, 2 out]
          n932 = call "draw crosshair imaq.vi"("Color"=u32 16774656, "Target.Y"=w293, "size"=cluster{"xhair size":dbl, "xhair size 2":dbl} {"xhair size"=25.0, "xhair size 2"=25.0}, "Target.X"=w294, "Bounding Rectangle"=T15 {"Left"=0, "Top"=0, "Right"=0, "Bottom"=0}, "image in"=w289) -> ("error out"=→"error out":errorcluster, "image out"=w288:T9)  [unwired: 4 in]
          n933 = call "draw box imaq.vi"("Color"=u32 1244928, "Rectangle"=w290, "image in"=w288) -> ()  [unwired: 7 in, 2 out]
        }
        n934 = property on="ActiveMotor" class="Ring (strict)"() -> ("Strings []"=w261:string[])  [unwired: 2 in, 2 out]
        n935 = Index Array(array=w261, index="ActiveMotor") -> (element=w262:string)
        n936 = Not Equal?(x="ActiveMotorName::99", y=w262) -> (x != y?=w263:bool)
        n937 = case shown="True" w263 {
          tunnel: w261 -> [_ w285]
          tunnel: "ActiveMotorName::99" -> [_ w284]
          frame False {
          }
          frame True {
            n938 = Search 1D Array(1D array=w285, element=w284) -> (index of element=w283:i32)  [unwired: 1 in]
            n939 = property on="ActiveMotor" class="Ring (strict)"("Value"=w283) -> ()  [unwired: 2 in, 2 out]
          }
        }
        n940 = property on="ActiveMotor 2" class="Ring (strict)"() -> ("Strings []"=w252:string[])  [unwired: 2 in, 2 out]
        n941 = Index Array(array=w252, index="ActiveMotor 2") -> (element=w256:string)
        n942 = Not Equal?(x="ActiveMotorName::98", y=w256) -> (x != y?=w255:bool)
        n943 = case shown="True" w255 {
          tunnel: w252 -> [_ w282]
          tunnel: "ActiveMotorName::98" -> [_ w281]
          frame False {
          }
          frame True {
            n944 = Search 1D Array(1D array=w282, element=w281) -> (index of element=w280:i32)  [unwired: 1 in]
            n945 = property on="ActiveMotor 2" class="Ring (strict)"("Value"=w280) -> ()  [unwired: 2 in, 2 out]
          }
        }
      }
      n946 = control-ref of="This Application"() -> (w243:refnum<vi>)
      n947 = control-ref of="This VI"() -> (w247:refnum<vi>)
      n948 = Current VI's Menubar() -> (w246:refnum<k9>)
      n949 = call "GUI_Master_subvi_reentrant_queues.vi"("This Application"=w243, "error in (no error)"=w244, "tcp data event"=w242, "Caller menu reference"=w246, "Caller VI ref"=w247) -> ("error out"=→"error IO 2":errorcluster)  [unwired: 6 in]
      n950 = Unbundle By Name(w132) -> ("Data Value Reference out"=w131:refnum<k34>)
      n951 = for {
        tunnel: w161 -> [w251] mode=indexing
        tunnel: w160 -> [w250]
        tunnel: [w249] -> w130
        n952 = call "IMAQ Dispose"("Image"=w251, "error in (no error)"=w250) -> ("error out"=w249:errorcluster)  [unwired: 4 in]
      }
      n953 = TDMS Close(8:w130, 11:w131) -> (0:→"error out 2":errorcluster)  [unwired: 1 out]
    }
  }
